vi "NMS_1_1_LTbridge_DiagonalLinearSweep.vi"(1 "Offset":dbl, 4 "b, pF":dbl, 5 "k, pF/V":dbl, 6 "LT bridge\ncalibration":bool, 7 "sweep rate, /min":dbl, 8 "sweep to:":dbl, 9 "sweep":T3(radio)) -> (2 "intercept":dbl, 3 "slope":dbl)   [LabVIEW 2010]
uses:
  Users/Geliang/geliang 1/Desktop/NMS_1_0/Channel.ctl
  Users/Geliang/geliang 1/Desktop/NMS_1_0/Measure.ctl
  Users/Geliang/geliang 1/Desktop/NMS_1_0/HULK SMS/SMScontrols.ctl
  Users/Geliang/geliang 1/Desktop/NMS_1_0/Source.ctl
  <vilib>/Utility/file.llb/Write To Spreadsheet File (DBL).vi
  <vilib>/gmath/NI_Gmath.lvlib
  <vilib>/Analysis/NI_AALPro.lvlib
panel:
  in  "DC bias neg (V)":dbl
  in  "wait to set voltage, msec":u32=3000
  in  "2182A 4":bool
  in  "2182A 3":bool
  in  "2182A 2":bool
  in  "2182A 1":bool
  in  "Slave Channel":T1
  in  "DC bias pos (V)":dbl
  in  "DC_resistance":bool
  in  "Slope":dbl
  in  "Double Sweep":bool
  out "read buffer MercuryIPS":string
  out "MercuryIPS_Error":errorcluster
  in  "MercuryITC":refnum<visa-resource-name>
  in  "MercuryIPS":refnum<visa-resource-name>
  in  "MercuryIPS":bool
  out "x-y*floor(x/y)":i32
  out "XY Graph 2":T2(graph)
  out "R-square total":dbl
  out "XY Graph":T2(graph)
  out "off-zero voltage":dbl
  out "C sample, pF":dbl
  out "R-square":dbl
  in  "pm":dbl=0.04
  in  "points":i16
  in  "C ref, pF":dbl=0.24169
  in  "V exc sample":dbl=0.2
  in  "V exc ref (SR830_2)":dbl=0.18
  in  "LT bridge":bool
  out "Word from HULK!":string
  out "CRYogenic:(":errorcluster
  in  "2182A 5 addr":u8=15
  in  "Hulk_B_meas (Vnano)":bool
  in  "Hulk_SMS_addr":refnum<visa-resource-name>="TCPIP0::10.99.75.17::inst0::INSTR"
  in  "lower limit":dbl
  in  "upper limit":dbl
  in  "continuous":bool
  in  "auto\nrange B":bool
  out "status 2":bool
  out "status":bool
  in  "Show cursor":bool
  in  "time/point, sec":dbl
  out "sweep value":dbl
  out "time delay, ms":dbl
  out "current time":timestamp format="%<%H:%M:%S%1u>T"
  in  "Pause":bool
  in  "LS332 A":bool
  in  "LS332 B":bool
  in  "LS332 addr":u8=28
  in  "LS340 B":bool
  in  "LS340 A":bool
  in  "LS340 addr":u8=28
  in  "AH2700A addr":u8=29
  in  "AH2700A C and L":bool
  in  "AH2500 addr":u8=28
  in  "AH2500 C and L":bool
  in  "2182A 4 ch2":bool
  in  "2182A 4 ch1":bool
  in  "2182A 3 ch2":bool
  in  "2182A 3 ch1":bool
  in  "2182A 2 ch2":bool
  in  "2182A 2 ch1":bool
  in  "2182A 4 addr":u8=18
  in  "2182A 3 addr":u8=17
  in  "2182A 2 addr":u8=16
  in  "2182A 1 addr":u8=15
  in  "2182A 1 ch2":bool
  in  "2182A 1 ch1":bool
  in  "2400 3 addr":u8=14
  in  "2400 2 addr":u8=13
  in  "2400 1 addr":u8=12
  in  "2336A addr":refnum<visa-resource-name>="TCPIP0::10.99.75.17::inst0::INSTR"
  in  "measure time":bool
  in  "2636A smub meas i":bool
  in  "2636A smub meas v":bool
  in  "2636A smua meas i":bool
  in  "2636A smua meas v":bool
  in  "2400 3 meas i":bool
  in  "2400 2 meas i":bool
  in  "2400 2 meas v":bool
  in  "2400 3 meas v":bool
  in  "2400 1 meas i":bool
  in  "2400 1 meas v":bool
  in  "auto\nrange A":bool
  in  "SR830 5 oop":bool
  in  "SR830 5 ip":bool
  in  "SR830 4 oop":bool
  in  "SR830 4 ip":bool
  in  "SR830 3 oop":bool
  in  "SR830 3 ip":bool
  in  "SR830 2 oop":bool
  in  "SR830 2 ip":bool
  in  "SR830 1 oop":bool
  in  "SR830 1 ip":bool
  in  "SR830 5 addr":u8=5
  in  "SR830 4 addr":u8=4
  in  "SR830 3 addr":u8=3
  in  "SR830 2 addr":u8=2
  in  "SR830 1 addr":u8=1
  in  "Y_axis_formula":string
  in  "X_axis_formula":string
  in  "formula_variables":string[](array[string])
  in  "stop":bool
  in  "ready/go":bool
  in  "oldStyle":bool
  out "Data file:":path=path "C:/Users/Artem/data/Year2012/July2012/Jul1312/Jul1312x034.dat"
  in  "Yaxis":u16(ring) caption="Y-axis:" items=["V_sweep_2636a_smub", "2636A_smua_v", "2636A_smua_i", "2636A_smub_v", "2636A_smub_i", "formula"]
  out "data":dbl[](array[numeric])
  out "XY Graph":cluster{dbl[], dbl[]}(graph)
  in  "Xaxis":u16(ring) caption="X-axis:" items=["V_sweep_2636a_smub", "2636A_smua_v", "2636A_smua_i", "2636A_smub_v", "2636A_smub_i", "formula"]
  out "Figure_axis":string[](array[string])
  out "data_caption":string
  # "measure DC res (commute)"
  # "source 2400_2"
  # "SourceMeters"
  # "address"
  # "Hulk_SMS"
  # "MercuryIPS"
  # "2400_1"
  # "2400_2"
  # "2400_3"
  # "2636A_smua"
  # "2636A_smub"
  # "time"
  # "sweep"
  # "measure"
  # "voltage (_v)"
  # "measure with\n2182A_5_ch1"
  # "Field"
  # "current (_i)"
  # "Temperature"
  # "for 2636A_smub slave"
  # "address"
  # "measure"
  # "LS332"
  # "LS340"
  # "MercuryITC"
  # "input A (_A)"
  # "input B (_B)"
  # "LT capacitance bridge on chip"
  # "Capacitance"
  # "with SR830_1"
  # "address"
  # "LTbridge"
  # "measure"
  # "AH2500"
  # "AH2700A"
  # "capacitance (_c)"
  # "and loss (_l)"
  # "every"
  # "Nanovoltmeters"
  # "address"
  # "measure"
  # "2182A_1"
  # "2182A_2"
  # "2182A_3"
  # "2182A_4"
  # "channel 1 (_ch1)"
  # "channel 2 (_ch2)"
  # "(not recommended, slow)"
  # "Lock-in amplifiers"
  # "address"
  # "measure"
  # "SR830_1"
  # "SR830_2"
  # "SR830_3"
  # "SR830_4"
  # "SR830_5"
  # "in phase (_ip)"
  # "out of phase (_oop)"
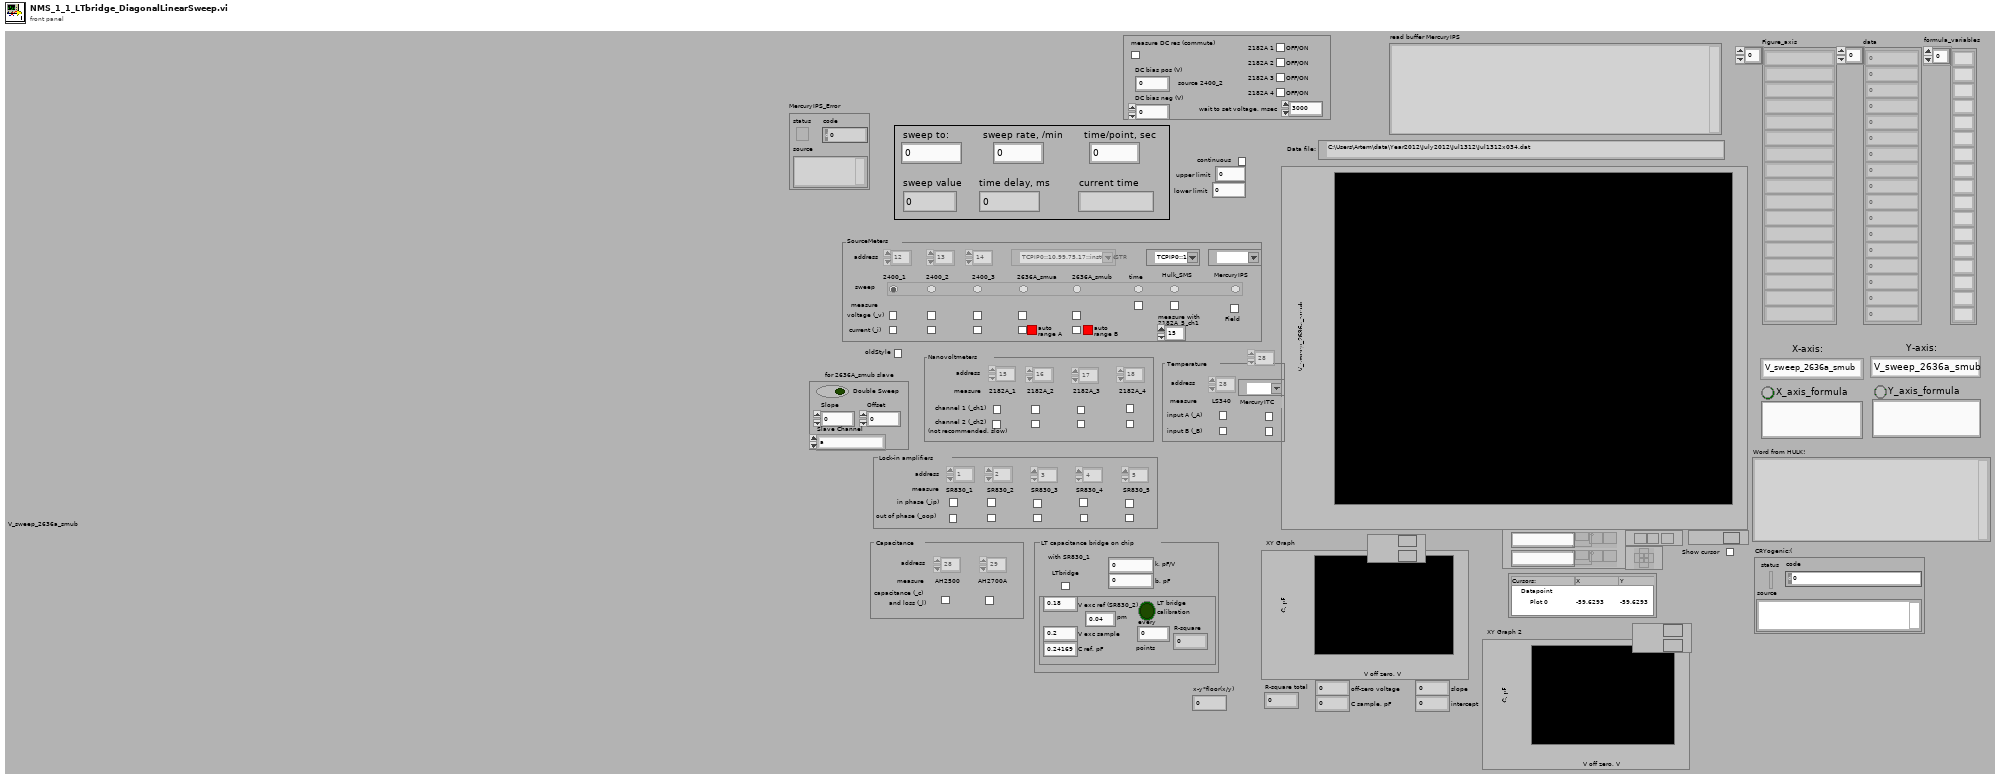
[diagram p1: front panel]
types:
  T1 = typedef "Channel.ctl" = enum16{"a", "b"}
  T2 = cluster{"emty array for LT bridge calibration":dbl[], "Best Linear Fit":dbl[]}[]
  T3 = enum32{"Radio Selection 1", "Radio Selection 2", "Radio Selection 3", "Radio Selection 4", "Radio Selection 5", "Radio Selection 6", "Radio Selection 7", "Radio Selection 8"}
  T4 = typedef "Measure.ctl" = enum16{"Voltage", "Current", "Resistance", "Power"}
  T5 = typedef "SMScontrols.ctl" = enum16{"UPDATE", "GET OUTPUT", "RAMP ZERO", "RAMP MID", "RAMP MAX", "RAMP STATUS", "PAUSE OFF", "PAUSE ON", "HEATER OFF", "HEATER ON", "TESLA OFF", "TESLA ON", "DIRECTION +", "DIRECTION -", "DIRECTION 0", "SET MID", "SET MAX", "SET RAMP", "SET LIMIT", "SET TPA", "SET HEATER"}
  T6 = enum8{"Enabled", "Disabled", "Disabled and Grayed Out"}
  T7 = enum32{"Radio Selection 1", "Radio Selection 2", "Radio Selection 3", "Radio Selection 4", "Radio Selection 5", "Radio Selection 6", "Radio Selection 7"}
  T8 = typedef "Source.ctl" = enum16{"Current", "Voltage"}
  T9 = cluster{"emty array for LT bridge calibration":dbl[], "emty array for LT bridge calibration":dbl[]}
  T10 = cluster{"emty array for LT bridge calibration":dbl[], "Best Linear Fit":dbl[]}
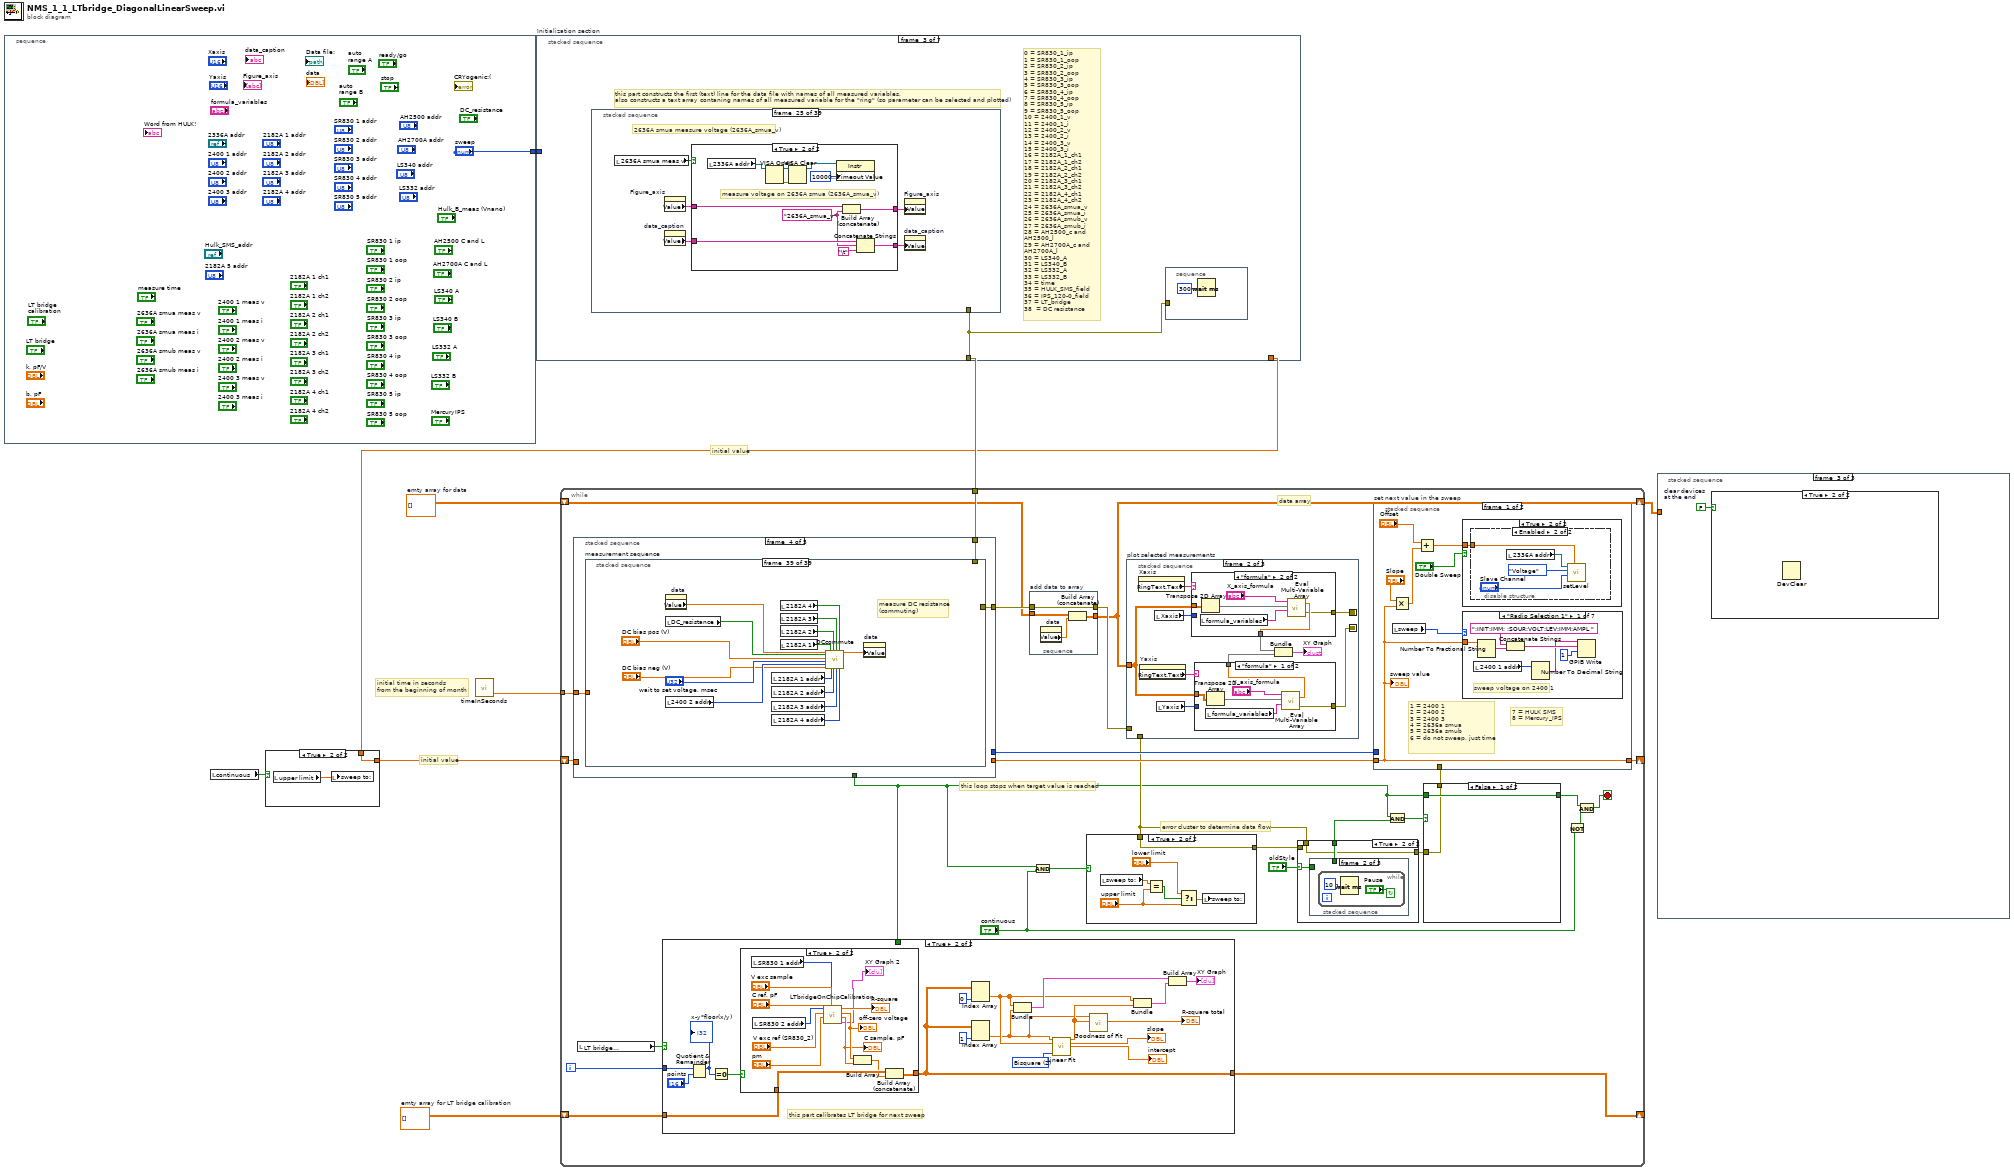
[diagram p0: block diagram]
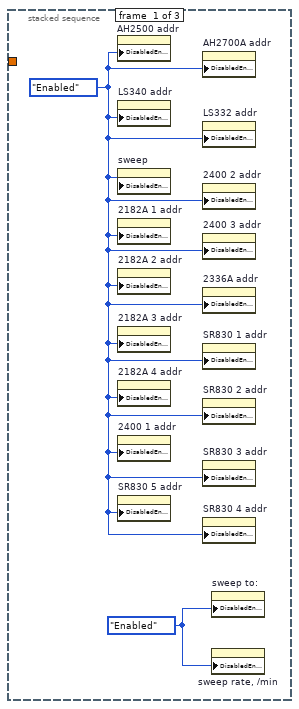
[diagram p3: hidden frame]
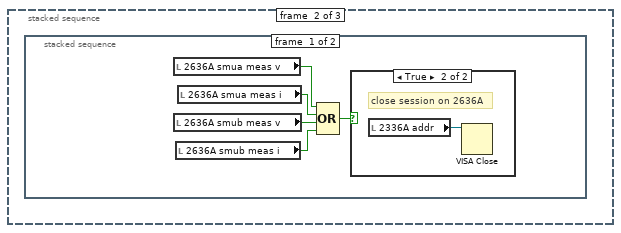
[diagram p4: hidden frame]
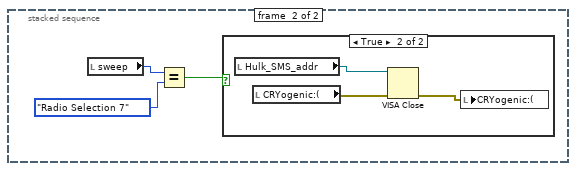
[diagram p6: hidden frame]
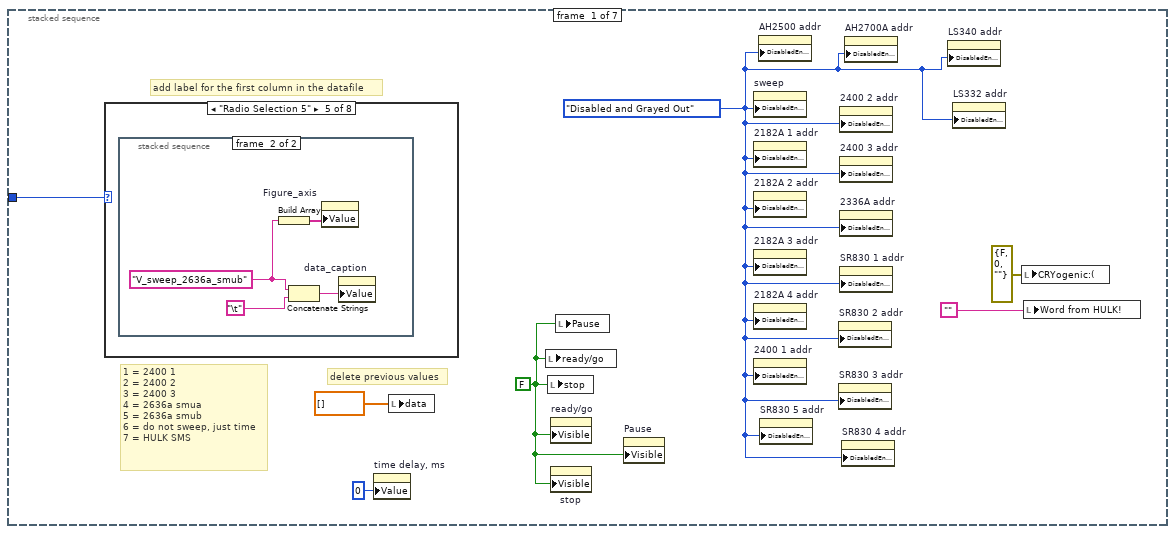
[diagram p9: hidden frame]
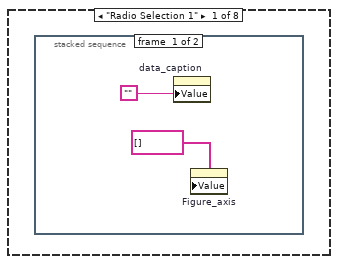
[diagram p10: hidden frame]
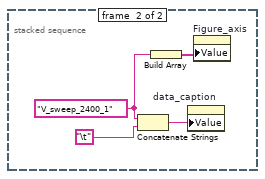
[diagram p11: hidden frame]
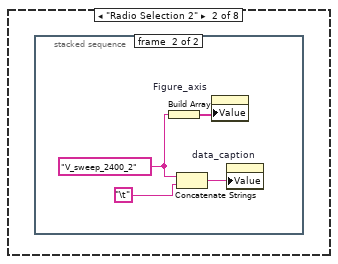
[diagram p12: hidden frame]
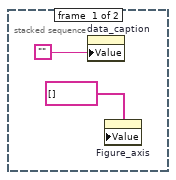
[diagram p13: hidden frame]
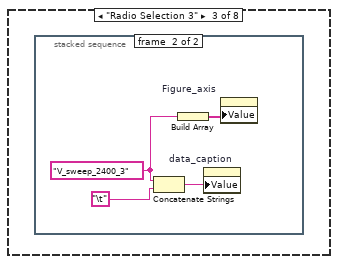
[diagram p14: hidden frame]
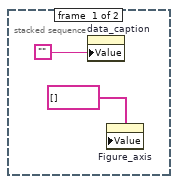
[diagram p15: hidden frame]
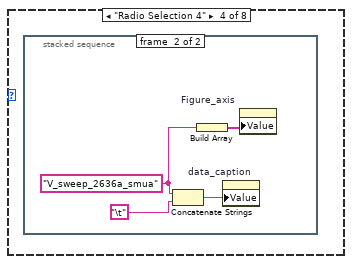
[diagram p16: hidden frame]
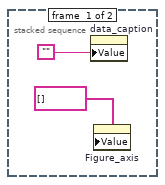
[diagram p17: hidden frame]
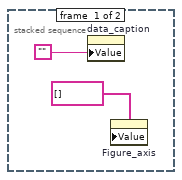
[diagram p18: hidden frame]
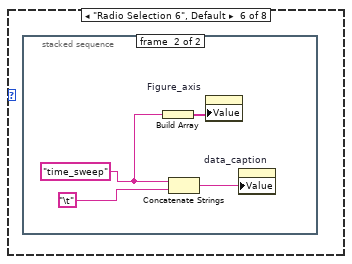
[diagram p19: hidden frame]
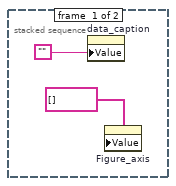
[diagram p20: hidden frame]
diagram:
  w1 = dbl[][] []  # emty array for LT bridge calibration
  w8 = dbl[][] []  # emty array for data
  # "initial value"
  # "initial value"
  # "initial time in seconds\nfrom the beginning of month"
  n1 = stacked-sequence {
    tunnel: ["sweep"] -> w6
    frame #0 {
    }
  }
  n2 = local read "continuous"() -> (w4:bool)
  n3 = call "timeInSeconds.vi"() -> ("Numeric"=w7:dbl)  [unwired: 2 in, 1 out]
  n4 = stacked-sequence "Initialization section" {
    tunnel: [_ _ w79 _ _ _ _] -> w9
    tunnel: [_ _ _ w672 _ _ _] -> w3
    tunnel: w6 -> [w16 _ _ _ _ _ _]
    frame #0 {
      w14 = T6."Disabled and Grayed Out" ("Disabled")
      w15 = FALSE ("stop")
      # "add label for the first column in the datafile"
      # "1 = 2400 1\n2 = 2400 2\n3 = 2400 3\n4 = 2636a smua\n5 = 2636a smub\n6 = do not sweep, just time\n7 = HULK SMS"
      # "delete previous values"
      n5 = case shown="\"Radio Selection 5\"" w16 {
        frame "Radio Selection 1" {
          n6 = stacked-sequence {
            frame #0 {
              n7 = property on="data_caption" class="Str"("Value"="") -> ()  [unwired: 2 in, 2 out]
              n8 = property on="Figure_axis" class="Arr (strict)"("Value"=string[] [] ("Figure_axis_string")) -> ()  [unwired: 2 in, 2 out]
            }
            frame #1 {
              w20 = "V_sweep_2400_1" ("V_sweep")
              n9 = Concatenate Strings(w20, "\t") -> (w22:string)
              n10 = Build Array(w20) -> (w21:string[])
              n11 = property on="data_caption" class="Str"("Value"=w22) -> ()  [unwired: 2 in, 2 out]
              n12 = property on="Figure_axis" class="Arr (strict)"("Value"=w21) -> ()  [unwired: 2 in, 2 out]
            }
          }
        }
        frame "Radio Selection 2" {
          n13 = stacked-sequence {
            frame #0 {
              n14 = property on="data_caption" class="Str"("Value"="") -> ()  [unwired: 2 in, 2 out]
              n15 = property on="Figure_axis" class="Arr (strict)"("Value"=string[] [] ("Figure_axis_string")) -> ()  [unwired: 2 in, 2 out]
            }
            frame #1 {
              w26 = "V_sweep_2400_2" ("V_sweep")
              n16 = Build Array(w26) -> (w27:string[])
              n17 = Concatenate Strings(w26, "\t") -> (w29:string)
              n18 = property on="Figure_axis" class="Arr (strict)"("Value"=w27) -> ()  [unwired: 2 in, 2 out]
              n19 = property on="data_caption" class="Str"("Value"=w29) -> ()  [unwired: 2 in, 2 out]
            }
          }
        }
        frame "Radio Selection 3" {
          n20 = stacked-sequence {
            frame #0 {
              n21 = property on="data_caption" class="Str"("Value"="") -> ()  [unwired: 2 in, 2 out]
              n22 = property on="Figure_axis" class="Arr (strict)"("Value"=string[] [] ("Figure_axis_string")) -> ()  [unwired: 2 in, 2 out]
            }
            frame #1 {
              w32 = "V_sweep_2400_3" ("V_sweep")
              n23 = Concatenate Strings(w32, "\t") -> (w35:string)
              n24 = Build Array(w32) -> (w33:string[])
              n25 = property on="data_caption" class="Str"("Value"=w35) -> ()  [unwired: 2 in, 2 out]
              n26 = property on="Figure_axis" class="Arr (strict)"("Value"=w33) -> ()  [unwired: 2 in, 2 out]
            }
          }
        }
        frame "Radio Selection 4" {
          n27 = stacked-sequence {
            frame #0 {
              n28 = property on="data_caption" class="Str"("Value"="") -> ()  [unwired: 2 in, 2 out]
              n29 = property on="Figure_axis" class="Arr (strict)"("Value"=string[] [] ("Figure_axis_string")) -> ()  [unwired: 2 in, 2 out]
            }
            frame #1 {
              w38 = "V_sweep_2636a_smua" ("V_sweep")
              n30 = Concatenate Strings(w38, "\t") -> (w41:string)
              n31 = Build Array(w38) -> (w39:string[])
              n32 = property on="data_caption" class="Str"("Value"=w41) -> ()  [unwired: 2 in, 2 out]
              n33 = property on="Figure_axis" class="Arr (strict)"("Value"=w39) -> ()  [unwired: 2 in, 2 out]
            }
          }
        }
        frame "Radio Selection 5" {
          n34 = stacked-sequence {
            frame #0 {
              n35 = property on="data_caption" class="Str"("Value"="") -> ()  [unwired: 2 in, 2 out]
              n36 = property on="Figure_axis" class="Arr (strict)"("Value"=string[] [] ("Figure_axis_string")) -> ()  [unwired: 2 in, 2 out]
            }
            frame #1 {
              w44 = "V_sweep_2636a_smub" ("V_sweep")
              n37 = Build Array(w44) -> (w45:string[])
              n38 = Concatenate Strings(w44, "\t") -> (w47:string)
              n39 = property on="Figure_axis" class="Arr (strict)"("Value"=w45) -> ()  [unwired: 2 in, 2 out]
              n40 = property on="data_caption" class="Str"("Value"=w47) -> ()  [unwired: 2 in, 2 out]
            }
          }
        }
        frame "Radio Selection 6", Default {
          n41 = stacked-sequence {
            frame #0 {
              n42 = property on="data_caption" class="Str"("Value"="") -> ()  [unwired: 2 in, 2 out]
              n43 = property on="Figure_axis" class="Arr (strict)"("Value"=string[] [] ("Figure_axis_string")) -> ()  [unwired: 2 in, 2 out]
            }
            frame #1 {
              w50 = "time_sweep" ("V_sweep")
              n44 = Build Array(w50) -> (w51:string[])
              n45 = Concatenate Strings(w50, "\t") -> (w52:string)
              n46 = property on="Figure_axis" class="Arr (strict)"("Value"=w51) -> ()  [unwired: 2 in, 2 out]
              n47 = property on="data_caption" class="Str"("Value"=w52) -> ()  [unwired: 2 in, 2 out]
            }
          }
        }
        frame "Radio Selection 7" {
          # "sweep Hulk SMS"
          n48 = stacked-sequence {
            frame #0 {
              n49 = property on="data_caption" class="Str"("Value"="") -> ()  [unwired: 2 in, 2 out]
              n50 = property on="Figure_axis" class="Arr (strict)"("Value"=string[] [] ("Figure_axis_string")) -> ()  [unwired: 2 in, 2 out]
            }
            frame #1 {
              w56 = "HULK_SMS_output" ("V_sweep")
              n51 = Build Array(w56) -> (w57:string[])
              n52 = Concatenate Strings(w56, "\t") -> (w59:string)
              n53 = property on="Figure_axis" class="Arr (strict)"("Value"=w57) -> ()  [unwired: 2 in, 2 out]
              n54 = property on="data_caption" class="Str"("Value"=w59) -> ()  [unwired: 2 in, 2 out]
            }
          }
        }
        frame "Radio Selection 8" {
          # "sweep Mercury IPS"
          n55 = stacked-sequence {
            frame #0 {
              n56 = property on="data_caption" class="Str"("Value"="") -> ()  [unwired: 2 in, 2 out]
              n57 = property on="Figure_axis" class="Arr (strict)"("Value"=string[] [] ("Figure_axis_string")) -> ()  [unwired: 2 in, 2 out]
            }
            frame #1 {
              w62 = "B_Sweep_Mercury_IPS" ("V_sweep")
              n58 = Build Array(w62) -> (w63:string[])
              n59 = Concatenate Strings(w62, "\t") -> (w65:string)
              n60 = property on="Figure_axis" class="Arr (strict)"("Value"=w63) -> ()  [unwired: 2 in, 2 out]
              n61 = property on="data_caption" class="Str"("Value"=w65) -> ()  [unwired: 2 in, 2 out]
            }
          }
        }
      }
      n62 = property on="time delay, ms" class="DigNum (strict)"("Value"=u32 0 ("delib time delay")) -> ()  [unwired: 2 in, 2 out]
      n63 = local write "data"(dbl[] [] ("data")) -> ()
      n64 = local write "ready/go"(w15) -> ()
      n65 = local write "stop"(w15) -> ()
      n66 = property on="ready/go" class="Bool (strict)"("Visible"=w15) -> ()  [unwired: 2 in, 2 out]
      n67 = property on="stop" class="Bool (strict)"("Visible"=w15) -> ()  [unwired: 2 in, 2 out]
      n68 = local write "Pause"(w15) -> ()
      n69 = property on="Pause" class="Bool (strict)"("Visible"=w15) -> ()  [unwired: 2 in, 2 out]
      n70 = property on="sweep" class="RadioBtnsControl (strict)"("DisabledEnum"=w14) -> ()  [unwired: 2 in, 2 out]
      n71 = property on="2182A 1 addr" class="DigNum (strict)"("DisabledEnum"=w14) -> ()  [unwired: 2 in, 2 out]
      n72 = property on="2182A 2 addr" class="DigNum (strict)"("DisabledEnum"=w14) -> ()  [unwired: 2 in, 2 out]
      n73 = property on="2182A 3 addr" class="DigNum (strict)"("DisabledEnum"=w14) -> ()  [unwired: 2 in, 2 out]
      n74 = property on="2182A 4 addr" class="DigNum (strict)"("DisabledEnum"=w14) -> ()  [unwired: 2 in, 2 out]
      n75 = property on="2400 1 addr" class="DigNum (strict)"("DisabledEnum"=w14) -> ()  [unwired: 2 in, 2 out]
      n76 = property on="AH2500 addr" class="DigNum (strict)"("DisabledEnum"=w14) -> ()  [unwired: 2 in, 2 out]
      n77 = property on="SR830 5 addr" class="DigNum (strict)"("DisabledEnum"=w14) -> ()  [unwired: 2 in, 2 out]
      n78 = property on="SR830 2 addr" class="DigNum (strict)"("DisabledEnum"=w14) -> ()  [unwired: 2 in, 2 out]
      n79 = property on="SR830 3 addr" class="DigNum (strict)"("DisabledEnum"=w14) -> ()  [unwired: 2 in, 2 out]
      n80 = property on="2400 2 addr" class="DigNum (strict)"("DisabledEnum"=w14) -> ()  [unwired: 2 in, 2 out]
      n81 = property on="2400 3 addr" class="DigNum (strict)"("DisabledEnum"=w14) -> ()  [unwired: 2 in, 2 out]
      n82 = property on="2336A addr" class="VISAName"("DisabledEnum"=w14) -> ()  [unwired: 2 in, 2 out]
      n83 = property on="SR830 1 addr" class="DigNum (strict)"("DisabledEnum"=w14) -> ()  [unwired: 2 in, 2 out]
      n84 = property on="SR830 4 addr" class="DigNum (strict)"("DisabledEnum"=w14) -> ()  [unwired: 2 in, 2 out]
      n85 = property on="AH2700A addr" class="DigNum (strict)"("DisabledEnum"=w14) -> ()  [unwired: 2 in, 2 out]
      n86 = property on="LS340 addr" class="DigNum (strict)"("DisabledEnum"=w14) -> ()  [unwired: 2 in, 2 out]
      n87 = property on="LS332 addr" class="DigNum (strict)"("DisabledEnum"=w14) -> ()  [unwired: 2 in, 2 out]
      n88 = local write "CRYogenic:("(errorcluster {"status"=FALSE, "code"=0, "source"=""} ("CRYogenic:(")) -> ()
      n89 = local write "Word from HULK!"("") -> ()
    }
    frame #1 {
      n90 = local read "2636A smua meas v"() -> (w71:bool)
      n91 = local read "2636A smub meas v"() -> (w69:bool)
      n92 = local read "2636A smub meas i"() -> (w68:bool)
      n93 = local read "2636A smua meas i"() -> (w70:bool)
      n94 = Compound Arithmetic op=OR(w71, w70, w69, w68) -> (w67:bool)
      n95 = case shown="True" w67 {
        frame False {
        }
        frame True {
          # "opens session for 2636a system sourcemeter"
          n96 = local read "2336A addr"() -> (w78:refnum<visa-resource-name>)
          n97 = VISA Close(VISA resource name=w78) -> ()  [unwired: 1 in, 1 out]
        }
      }
      n98 = local read "MercuryIPS"() -> (w66:bool)
      n99 = case shown="True" w66 {
        frame False {
        }
        frame True {
          n100 = local read "MercuryIPS"() -> (w74:refnum<visa-resource-name>)
          n101 = VISA Close(VISA resource name=w74) -> (error out=w73:errorcluster)  [unwired: 1 in]
          n102 = flat-sequence {
            tunnel: w73 -> [w76]
            tunnel: [w76] -> w72
            frame #0 {
              n103 = Wait (ms)(milliseconds to wait=u32 200) -> ()  [unwired: 1 out]
            }
          }
          n104 = VISA Open(error in (no error)=w72, VISA resource name=w74) -> (error out=w75:errorcluster)  [unwired: 3 in, 1 out]
          n105 = local write "MercuryIPS_Error"(w75) -> ()
        }
      }
    }
    frame #2 {
      # "0 = SR830_1_ip\n1 = SR830_1_oop\n2 = SR830_2_ip\n3 = SR830_2_oop\n4 = SR830_3_ip\n5 = SR830_3_oop\n6 = SR830_4_ip \n7 = SR830_4_oop \n8 = SR830_5_ip \n9 = SR830_5_oop \n10 = 2400_1_v \n11 = 2400_1_i \n12 = 2400_2_v\n13 = 2400_2_i \n14 = 2400_3_v \n15 = 2400_3_i \n16 = 2182A_1_ch1 \n17 = 2182A_1_ch2 \n18 = 2182A_2_ch1 \n19 = 2182A_2_ch2\n20 = 2182A_3_ch1 \n21 = 2182A_3_ch2 \n22 = 2182A_4_ch1 \n23 = 2182A_4_ch2 \n24 = 2636A_smua_v \n25 = 2636A_smua_i \n26 = 2636A_smub_v \n27 = 2636A_smub_i \n28 = AH2500_c and AH2500_l \n29 = AH2700A_c and AH2700A_l\n30 = LS340_A\n31 = LS340_B\n32 = LS332_A\n33 = LS332_B\n34 = time\n35 = HULK_SMS_field\n36 = IPS_120-0_field\n37 = LT_bridge\n38  = DC resistance"
      # "this part constructs the first (text) line for the data file with names of all measured variables,\nalso constructs a text array contaning names of all measured variable for the \"ring\" (so parameter can be selected and plotted)"
      n106 = stacked-sequence {
        tunnel: [w81 _ _ _ _ _ _ _ _ _ _ _ _ _ _ _ _ _ _ _ _ _ _ _ _ _ _ _ _ _ _ _ _ _ _ _ _ _ _] -> w79
        frame #0 {
          # "SR830 1 in phase (SR830_1_ip)"
          n107 = local read "SR830 1 ip"() -> (w86:bool)
          n108 = property on="Figure_axis" class="Arr (strict)"() -> ("Value"=w83:string[])  [unwired: 2 in, 2 out]
          n109 = property on="data_caption" class="Str"() -> ("Value"=w85:string)  [unwired: 2 in, 2 out]
          n110 = case shown="True" w86 {
            tunnel: w85 -> [w88 w94]
            tunnel: [w88 w93] -> w84
            tunnel: w83 -> [w87 w91]
            tunnel: [w87 w89] -> w82
            frame False {
              # "not measure SR830 1 in phase signal (SR830_1_ip)"
            }
            frame True {
              w90 = "SR830_1_ip"
              # "measure SR830 1 in phase signal (SR830_1_ip)"
              n111 = local read "SR830 1 addr"() -> (w95:u8)
              n112 = Number To Decimal String(number=w95) -> (decimal integer string=w96:string)  [unwired: 1 in]
              n113 = GPIB Clear(3:w96) -> ()  [unwired: 1 in, 2 out]
              n114 = Build Array (concatenate)(w91, w90) -> (w89:string[])
              n115 = Concatenate Strings(w94, w90, "\t") -> (w93:string)
            }
          }
          n116 = property on="Figure_axis" class="Arr (strict)"("Value"=w82) -> ()  [unwired: 2 in, 2 out]
          n117 = property on="data_caption" class="Str"("Value"=w84) -> (error out=w81:errorcluster)  [unwired: 2 in, 1 out]
        }
        frame #1 {
          # "SR830 1 out of phase (SR830_1_oop)"
          n118 = local read "SR830 1 oop"() -> (w101:bool)
          n119 = property on="Figure_axis" class="Arr (strict)"() -> ("Value"=w98:string[])  [unwired: 2 in, 2 out]
          n120 = property on="data_caption" class="Str"() -> ("Value"=w100:string)  [unwired: 2 in, 2 out]
          n121 = case shown="True" w101 {
            tunnel: w100 -> [w103 w109]
            tunnel: [w103 w108] -> w99
            tunnel: w98 -> [w102 w106]
            tunnel: [w102 w104] -> w97
            frame False {
              # "not measure SR830 1 out of phase signal (SR830_1_oop)"
            }
            frame True {
              w105 = "SR830_1_oop"
              # "measure SR830 1 out of phase signal (SR830_1_oop)"
              n122 = local read "SR830 1 addr"() -> (w110:u8)
              n123 = Number To Decimal String(number=w110) -> (decimal integer string=w111:string)  [unwired: 1 in]
              n124 = GPIB Clear(3:w111) -> ()  [unwired: 1 in, 2 out]
              n125 = Build Array (concatenate)(w106, w105) -> (w104:string[])
              n126 = Concatenate Strings(w109, w105, "\t") -> (w108:string)
            }
          }
          n127 = property on="Figure_axis" class="Arr (strict)"("Value"=w97) -> ()  [unwired: 2 in, 2 out]
          n128 = property on="data_caption" class="Str"("Value"=w99) -> ()  [unwired: 2 in, 2 out]
        }
        frame #2 {
          # "SR830 2 in phase (SR830_2_ip)"
          n129 = local read "SR830 2 ip"() -> (w116:bool)
          n130 = property on="Figure_axis" class="Arr (strict)"() -> ("Value"=w113:string[])  [unwired: 2 in, 2 out]
          n131 = property on="data_caption" class="Str"() -> ("Value"=w115:string)  [unwired: 2 in, 2 out]
          n132 = case shown="False" w116 {
            tunnel: w115 -> [w118 w124]
            tunnel: [w118 w123] -> w114
            tunnel: w113 -> [w117 w121]
            tunnel: [w117 w119] -> w112
            frame False {
              # "not measure SR830 2 in phase signal (SR830_2_ip)"
            }
            frame True {
              w120 = "SR830_2_ip"
              # "measure SR830 2 in phase signal (SR830_2_ip)"
              n133 = local read "SR830 2 addr"() -> (w125:u8)
              n134 = Number To Decimal String(number=w125) -> (decimal integer string=w126:string)  [unwired: 1 in]
              n135 = GPIB Clear(3:w126) -> ()  [unwired: 1 in, 2 out]
              n136 = Build Array (concatenate)(w121, w120) -> (w119:string[])
              n137 = Concatenate Strings(w124, w120, "\t") -> (w123:string)
            }
          }
          n138 = property on="Figure_axis" class="Arr (strict)"("Value"=w112) -> ()  [unwired: 2 in, 2 out]
          n139 = property on="data_caption" class="Str"("Value"=w114) -> ()  [unwired: 2 in, 2 out]
        }
        frame #3 {
          # "SR830 2 out of phase (SR830_2_oop)"
          n140 = local read "SR830 2 oop"() -> (w131:bool)
          n141 = property on="Figure_axis" class="Arr (strict)"() -> ("Value"=w128:string[])  [unwired: 2 in, 2 out]
          n142 = property on="data_caption" class="Str"() -> ("Value"=w130:string)  [unwired: 2 in, 2 out]
          n143 = case shown="True" w131 {
            tunnel: w130 -> [w133 w139]
            tunnel: [w133 w138] -> w129
            tunnel: w128 -> [w132 w136]
            tunnel: [w132 w134] -> w127
            frame False {
              # "not measure SR830 2 out of phase signal (SR830_2_oop)"
            }
            frame True {
              w135 = "SR830_2_oop"
              # "measure SR830 2 out of phase signal (SR830_2_oop)"
              n144 = local read "SR830 2 addr"() -> (w140:u8)
              n145 = Number To Decimal String(number=w140) -> (decimal integer string=w141:string)  [unwired: 1 in]
              n146 = GPIB Clear(3:w141) -> ()  [unwired: 1 in, 2 out]
              n147 = Build Array (concatenate)(w136, w135) -> (w134:string[])
              n148 = Concatenate Strings(w139, w135, "\t") -> (w138:string)
            }
          }
          n149 = property on="Figure_axis" class="Arr (strict)"("Value"=w127) -> ()  [unwired: 2 in, 2 out]
          n150 = property on="data_caption" class="Str"("Value"=w129) -> ()  [unwired: 2 in, 2 out]
        }
        frame #4 {
          # "SR830 3 in phase (SR830_3_ip)"
          n151 = local read "SR830 3 ip"() -> (w146:bool)
          n152 = property on="Figure_axis" class="Arr (strict)"() -> ("Value"=w143:string[])  [unwired: 2 in, 2 out]
          n153 = property on="data_caption" class="Str"() -> ("Value"=w145:string)  [unwired: 2 in, 2 out]
          n154 = case shown="False" w146 {
            tunnel: w145 -> [w148 w154]
            tunnel: [w148 w153] -> w144
            tunnel: w143 -> [w147 w151]
            tunnel: [w147 w149] -> w142
            frame False {
              # "not measure SR830 3 in phase signal (SR830_3_ip)"
            }
            frame True {
              w150 = "SR830_3_ip"
              # "measure SR830 3 in phase signal (SR830_3_ip)"
              n155 = local read "SR830 3 addr"() -> (w155:u8)
              n156 = Number To Decimal String(number=w155) -> (decimal integer string=w156:string)  [unwired: 1 in]
              n157 = GPIB Clear(3:w156) -> ()  [unwired: 1 in, 2 out]
              n158 = Build Array (concatenate)(w151, w150) -> (w149:string[])
              n159 = Concatenate Strings(w154, w150, "\t") -> (w153:string)
            }
          }
          n160 = property on="Figure_axis" class="Arr (strict)"("Value"=w142) -> ()  [unwired: 2 in, 2 out]
          n161 = property on="data_caption" class="Str"("Value"=w144) -> ()  [unwired: 2 in, 2 out]
        }
        frame #5 {
          # "SR830 3 out of phase (SR830_3_oop)"
          n162 = local read "SR830 3 oop"() -> (w161:bool)
          n163 = property on="Figure_axis" class="Arr (strict)"() -> ("Value"=w158:string[])  [unwired: 2 in, 2 out]
          n164 = property on="data_caption" class="Str"() -> ("Value"=w160:string)  [unwired: 2 in, 2 out]
          n165 = case shown="True" w161 {
            tunnel: w160 -> [w163 w169]
            tunnel: [w163 w168] -> w159
            tunnel: w158 -> [w162 w166]
            tunnel: [w162 w164] -> w157
            frame False {
              # "not measure SR830 3 out of phase signal (SR830_3_oop)"
            }
            frame True {
              w165 = "SR830_3_oop"
              # "measure SR830 3 out phase signal (SR830_3_oop)"
              n166 = local read "SR830 3 addr"() -> (w170:u8)
              n167 = Number To Decimal String(number=w170) -> (decimal integer string=w171:string)  [unwired: 1 in]
              n168 = GPIB Clear(3:w171) -> ()  [unwired: 1 in, 2 out]
              n169 = Build Array (concatenate)(w166, w165) -> (w164:string[])
              n170 = Concatenate Strings(w169, w165, "\t") -> (w168:string)
            }
          }
          n171 = property on="Figure_axis" class="Arr (strict)"("Value"=w157) -> ()  [unwired: 2 in, 2 out]
          n172 = property on="data_caption" class="Str"("Value"=w159) -> ()  [unwired: 2 in, 2 out]
        }
        frame #6 {
          # "SR830 4 in phase (SR830_4_ip)"
          n173 = local read "SR830 4 ip"() -> (w176:bool)
          n174 = property on="Figure_axis" class="Arr (strict)"() -> ("Value"=w173:string[])  [unwired: 2 in, 2 out]
          n175 = property on="data_caption" class="Str"() -> ("Value"=w175:string)  [unwired: 2 in, 2 out]
          n176 = case shown="True" w176 {
            tunnel: w175 -> [w178 w184]
            tunnel: [w178 w183] -> w174
            tunnel: w173 -> [w177 w181]
            tunnel: [w177 w179] -> w172
            frame False {
              # "not measure SR830 4 in phase signal (SR830_4_ip)"
            }
            frame True {
              w180 = "SR830_4_ip"
              # "measure SR830 4 in phase signal (SR830_4_ip)"
              n177 = local read "SR830 4 addr"() -> (w185:u8)
              n178 = Number To Decimal String(number=w185) -> (decimal integer string=w186:string)  [unwired: 1 in]
              n179 = GPIB Clear(3:w186) -> ()  [unwired: 1 in, 2 out]
              n180 = Build Array (concatenate)(w181, w180) -> (w179:string[])
              n181 = Concatenate Strings(w184, w180, "\t") -> (w183:string)
            }
          }
          n182 = property on="Figure_axis" class="Arr (strict)"("Value"=w172) -> ()  [unwired: 2 in, 2 out]
          n183 = property on="data_caption" class="Str"("Value"=w174) -> ()  [unwired: 2 in, 2 out]
        }
        frame #7 {
          # "SR830 4 out of phase (SR830_4_oop)"
          n184 = local read "SR830 4 oop"() -> (w191:bool)
          n185 = property on="Figure_axis" class="Arr (strict)"() -> ("Value"=w188:string[])  [unwired: 2 in, 2 out]
          n186 = property on="data_caption" class="Str"() -> ("Value"=w190:string)  [unwired: 2 in, 2 out]
          n187 = case shown="True" w191 {
            tunnel: w190 -> [w193 w199]
            tunnel: [w193 w198] -> w189
            tunnel: w188 -> [w192 w196]
            tunnel: [w192 w194] -> w187
            frame False {
              # "not measure SR830 4 out of phase signal (SR830_4_oop)"
            }
            frame True {
              w195 = "SR830_4_oop"
              # "measure SR830 4 out of phase signal (SR830_4_oop)"
              n188 = local read "SR830 4 addr"() -> (w200:u8)
              n189 = Number To Decimal String(number=w200) -> (decimal integer string=w201:string)  [unwired: 1 in]
              n190 = GPIB Clear(3:w201) -> ()  [unwired: 1 in, 2 out]
              n191 = Build Array (concatenate)(w196, w195) -> (w194:string[])
              n192 = Concatenate Strings(w199, w195, "\t") -> (w198:string)
            }
          }
          n193 = property on="Figure_axis" class="Arr (strict)"("Value"=w187) -> ()  [unwired: 2 in, 2 out]
          n194 = property on="data_caption" class="Str"("Value"=w189) -> ()  [unwired: 2 in, 2 out]
        }
        frame #8 {
          # "SR830 5 in phase (SR830_5_ip)"
          n195 = local read "SR830 5 ip"() -> (w206:bool)
          n196 = property on="Figure_axis" class="Arr (strict)"() -> ("Value"=w203:string[])  [unwired: 2 in, 2 out]
          n197 = property on="data_caption" class="Str"() -> ("Value"=w205:string)  [unwired: 2 in, 2 out]
          n198 = case shown="True" w206 {
            tunnel: w205 -> [w208 w214]
            tunnel: [w208 w213] -> w204
            tunnel: w203 -> [w207 w211]
            tunnel: [w207 w209] -> w202
            frame False {
              # "not measure SR830 5 in phase signal (SR830_5_ip)"
            }
            frame True {
              w210 = "SR830_5_ip"
              # "measure SR830 5 in phase signal (SR830_5_ip)"
              n199 = local read "SR830 5 addr"() -> (w215:u8)
              n200 = Number To Decimal String(number=w215) -> (decimal integer string=w216:string)  [unwired: 1 in]
              n201 = GPIB Clear(3:w216) -> ()  [unwired: 1 in, 2 out]
              n202 = Build Array (concatenate)(w211, w210) -> (w209:string[])
              n203 = Concatenate Strings(w214, w210, "\t") -> (w213:string)
            }
          }
          n204 = property on="Figure_axis" class="Arr (strict)"("Value"=w202) -> ()  [unwired: 2 in, 2 out]
          n205 = property on="data_caption" class="Str"("Value"=w204) -> ()  [unwired: 2 in, 2 out]
        }
        frame #9 {
          # "SR830 5 out of phase (SR830_5_oop)"
          n206 = local read "SR830 5 oop"() -> (w221:bool)
          n207 = property on="Figure_axis" class="Arr (strict)"() -> ("Value"=w218:string[])  [unwired: 2 in, 2 out]
          n208 = property on="data_caption" class="Str"() -> ("Value"=w220:string)  [unwired: 2 in, 2 out]
          n209 = case shown="False" w221 {
            tunnel: w220 -> [w223 w229]
            tunnel: [w223 w228] -> w219
            tunnel: w218 -> [w222 w226]
            tunnel: [w222 w224] -> w217
            frame False {
              # "not measure SR830 5 out of phase signal (SR830_5_oop)"
            }
            frame True {
              w225 = "SR830_5_oop"
              # "measure SR830 5 out of phase signal (SR830_5_oop)"
              n210 = local read "SR830 5 addr"() -> (w230:u8)
              n211 = Number To Decimal String(number=w230) -> (decimal integer string=w231:string)  [unwired: 1 in]
              n212 = GPIB Clear(3:w231) -> ()  [unwired: 1 in, 2 out]
              n213 = Build Array (concatenate)(w226, w225) -> (w224:string[])
              n214 = Concatenate Strings(w229, w225, "\t") -> (w228:string)
            }
          }
          n215 = property on="Figure_axis" class="Arr (strict)"("Value"=w217) -> ()  [unwired: 2 in, 2 out]
          n216 = property on="data_caption" class="Str"("Value"=w219) -> ()  [unwired: 2 in, 2 out]
        }
        frame #10 {
          # "2400 1 voltage measure (2400_1_v)"
          n217 = local read "2400 1 meas v"() -> (w236:bool)
          n218 = property on="Figure_axis" class="Arr (strict)"() -> ("Value"=w233:string[])  [unwired: 2 in, 2 out]
          n219 = property on="data_caption" class="Str"() -> ("Value"=w235:string)  [unwired: 2 in, 2 out]
          n220 = case shown="True" w236 {
            tunnel: w235 -> [w238 w244]
            tunnel: [w238 w243] -> w234
            tunnel: w233 -> [w237 w241]
            tunnel: [w237 w239] -> w232
            frame False {
              # "not measure 2400 1 voltage (2400_1_v)"
            }
            frame True {
              w240 = "2400_1_v"
              # "measure 2400 1 voltage (2400_1_v)"
              n221 = local read "2400 1 addr"() -> (w245:u8)
              n222 = Number To Decimal String(number=w245) -> (decimal integer string=w246:string)  [unwired: 1 in]
              n223 = GPIB Clear(3:w246) -> ()  [unwired: 1 in, 2 out]
              n224 = Build Array (concatenate)(w241, w240) -> (w239:string[])
              n225 = Concatenate Strings(w244, w240, "\t") -> (w243:string)
            }
          }
          n226 = property on="Figure_axis" class="Arr (strict)"("Value"=w232) -> ()  [unwired: 2 in, 2 out]
          n227 = property on="data_caption" class="Str"("Value"=w234) -> ()  [unwired: 2 in, 2 out]
        }
        frame #11 {
          # "2400 1 current measure (2400_1_i)"
          n228 = local read "2400 1 meas i"() -> (w251:bool)
          n229 = property on="Figure_axis" class="Arr (strict)"() -> ("Value"=w248:string[])  [unwired: 2 in, 2 out]
          n230 = property on="data_caption" class="Str"() -> ("Value"=w250:string)  [unwired: 2 in, 2 out]
          n231 = case shown="True" w251 {
            tunnel: w250 -> [w253 w259]
            tunnel: [w253 w258] -> w249
            tunnel: w248 -> [w252 w256]
            tunnel: [w252 w254] -> w247
            frame False {
              # "not measure 2400 1 current (2400_1_i)"
            }
            frame True {
              w255 = "2400_1_i"
              # "measure 2400 1 current (2400_1_i)"
              n232 = local read "2400 1 addr"() -> (w260:u8)
              n233 = Number To Decimal String(number=w260) -> (decimal integer string=w261:string)  [unwired: 1 in]
              n234 = GPIB Clear(3:w261) -> ()  [unwired: 1 in, 2 out]
              n235 = Build Array (concatenate)(w256, w255) -> (w254:string[])
              n236 = Concatenate Strings(w259, w255, "\t") -> (w258:string)
            }
          }
          n237 = property on="Figure_axis" class="Arr (strict)"("Value"=w247) -> ()  [unwired: 2 in, 2 out]
          n238 = property on="data_caption" class="Str"("Value"=w249) -> ()  [unwired: 2 in, 2 out]
        }
        frame #12 {
          # "2400 2 voltage measure (2400_2_v)"
          n239 = local read "2400 2 meas v"() -> (w266:bool)
          n240 = property on="Figure_axis" class="Arr (strict)"() -> ("Value"=w263:string[])  [unwired: 2 in, 2 out]
          n241 = property on="data_caption" class="Str"() -> ("Value"=w265:string)  [unwired: 2 in, 2 out]
          n242 = case shown="True" w266 {
            tunnel: w265 -> [w268 w274]
            tunnel: [w268 w273] -> w264
            tunnel: w263 -> [w267 w271]
            tunnel: [w267 w269] -> w262
            frame False {
              # "not measure 2400 2 voltage (2400_2_v)"
            }
            frame True {
              w270 = "2400_2_v"
              # "measure 2400 2 voltage (2400_2_v)"
              n243 = local read "2400 2 addr"() -> (w275:u8)
              n244 = Number To Decimal String(number=w275) -> (decimal integer string=w276:string)  [unwired: 1 in]
              n245 = GPIB Clear(3:w276) -> ()  [unwired: 1 in, 2 out]
              n246 = Build Array (concatenate)(w271, w270) -> (w269:string[])
              n247 = Concatenate Strings(w274, w270, "\t") -> (w273:string)
            }
          }
          n248 = property on="Figure_axis" class="Arr (strict)"("Value"=w262) -> ()  [unwired: 2 in, 2 out]
          n249 = property on="data_caption" class="Str"("Value"=w264) -> ()  [unwired: 2 in, 2 out]
        }
        frame #13 {
          # "2400 2 current measure (2400_2_i)"
          n250 = local read "2400 2 meas i"() -> (w281:bool)
          n251 = property on="Figure_axis" class="Arr (strict)"() -> ("Value"=w278:string[])  [unwired: 2 in, 2 out]
          n252 = property on="data_caption" class="Str"() -> ("Value"=w280:string)  [unwired: 2 in, 2 out]
          n253 = case shown="True" w281 {
            tunnel: w280 -> [w283 w289]
            tunnel: [w283 w288] -> w279
            tunnel: w278 -> [w282 w286]
            tunnel: [w282 w284] -> w277
            frame False {
              # "not measure 2400 2 current (2400_2_i)"
            }
            frame True {
              w285 = "2400_2_i"
              # "measure 2400 2 current (2400_2_i)"
              n254 = local read "2400 2 addr"() -> (w290:u8)
              n255 = Number To Decimal String(number=w290) -> (decimal integer string=w291:string)  [unwired: 1 in]
              n256 = GPIB Clear(3:w291) -> ()  [unwired: 1 in, 2 out]
              n257 = Build Array (concatenate)(w286, w285) -> (w284:string[])
              n258 = Concatenate Strings(w289, w285, "\t") -> (w288:string)
            }
          }
          n259 = property on="Figure_axis" class="Arr (strict)"("Value"=w277) -> ()  [unwired: 2 in, 2 out]
          n260 = property on="data_caption" class="Str"("Value"=w279) -> ()  [unwired: 2 in, 2 out]
        }
        frame #14 {
          # "2400 3 voltage measure (2400_3_v)"
          n261 = local read "2400 3 meas v"() -> (w296:bool)
          n262 = property on="Figure_axis" class="Arr (strict)"() -> ("Value"=w293:string[])  [unwired: 2 in, 2 out]
          n263 = property on="data_caption" class="Str"() -> ("Value"=w295:string)  [unwired: 2 in, 2 out]
          n264 = case shown="False" w296 {
            tunnel: w295 -> [w298 w304]
            tunnel: [w298 w303] -> w294
            tunnel: w293 -> [w297 w301]
            tunnel: [w297 w299] -> w292
            frame False {
              # "not measure 2400 3 voltage (2400_3_v)"
            }
            frame True {
              w300 = "2400_3_v"
              # "measure 2400 3 voltage (2400_3_v)"
              n265 = local read "2400 3 addr"() -> (w305:u8)
              n266 = Number To Decimal String(number=w305) -> (decimal integer string=w306:string)  [unwired: 1 in]
              n267 = GPIB Clear(3:w306) -> ()  [unwired: 1 in, 2 out]
              n268 = Build Array (concatenate)(w301, w300) -> (w299:string[])
              n269 = Concatenate Strings(w304, w300, "\t") -> (w303:string)
            }
          }
          n270 = property on="Figure_axis" class="Arr (strict)"("Value"=w292) -> ()  [unwired: 2 in, 2 out]
          n271 = property on="data_caption" class="Str"("Value"=w294) -> ()  [unwired: 2 in, 2 out]
        }
        frame #15 {
          # "2400 3 current measure (2400_3_i)"
          n272 = local read "2400 3 meas i"() -> (w311:bool)
          n273 = property on="Figure_axis" class="Arr (strict)"() -> ("Value"=w308:string[])  [unwired: 2 in, 2 out]
          n274 = property on="data_caption" class="Str"() -> ("Value"=w310:string)  [unwired: 2 in, 2 out]
          n275 = case shown="True" w311 {
            tunnel: w310 -> [w313 w319]
            tunnel: [w313 w318] -> w309
            tunnel: w308 -> [w312 w316]
            tunnel: [w312 w314] -> w307
            frame False {
              # "not measure 2400 3 current (2400_3_i)"
            }
            frame True {
              w315 = "2400_3_i"
              # "measure 2400 3 current (2400_3_i)"
              n276 = local read "2400 3 addr"() -> (w320:u8)
              n277 = Number To Decimal String(number=w320) -> (decimal integer string=w321:string)  [unwired: 1 in]
              n278 = GPIB Clear(3:w321) -> ()  [unwired: 1 in, 2 out]
              n279 = Build Array (concatenate)(w316, w315) -> (w314:string[])
              n280 = Concatenate Strings(w319, w315, "\t") -> (w318:string)
            }
          }
          n281 = property on="Figure_axis" class="Arr (strict)"("Value"=w307) -> ()  [unwired: 2 in, 2 out]
          n282 = property on="data_caption" class="Str"("Value"=w309) -> ()  [unwired: 2 in, 2 out]
        }
        frame #16 {
          # "2182A 1 channel 1 measure (2182A_1_ch1)"
          n283 = local read "2182A 1 ch1"() -> (w326:bool)
          n284 = property on="Figure_axis" class="Arr (strict)"() -> ("Value"=w323:string[])  [unwired: 2 in, 2 out]
          n285 = property on="data_caption" class="Str"() -> ("Value"=w325:string)  [unwired: 2 in, 2 out]
          n286 = case shown="False" w326 {
            tunnel: w325 -> [w328 w334]
            tunnel: [w328 w333] -> w324
            tunnel: w323 -> [w327 w331]
            tunnel: [w327 w329] -> w322
            frame False {
              # "not measure 2182A 1 channel 1 (2182A_1_ch1)"
            }
            frame True {
              w330 = "2182A_1_ch1"
              # "measure 2182A 1 channel 1 (2182A_1_ch1)"
              n287 = local read "2182A 1 addr"() -> (w335:u8)
              n288 = Number To Decimal String(number=w335) -> (decimal integer string=w336:string)  [unwired: 1 in]
              n289 = GPIB Clear(3:w336) -> ()  [unwired: 1 in, 2 out]
              n290 = Build Array (concatenate)(w331, w330) -> (w329:string[])
              n291 = Concatenate Strings(w334, w330, "\t") -> (w333:string)
            }
          }
          n292 = property on="Figure_axis" class="Arr (strict)"("Value"=w322) -> ()  [unwired: 2 in, 2 out]
          n293 = property on="data_caption" class="Str"("Value"=w324) -> ()  [unwired: 2 in, 2 out]
        }
        frame #17 {
          # "2182A 1 channel 2 measure (2182A_1_ch2)"
          n294 = local read "2182A 1 ch2"() -> (w341:bool)
          n295 = property on="Figure_axis" class="Arr (strict)"() -> ("Value"=w338:string[])  [unwired: 2 in, 2 out]
          n296 = property on="data_caption" class="Str"() -> ("Value"=w340:string)  [unwired: 2 in, 2 out]
          n297 = case shown="True" w341 {
            tunnel: w340 -> [w343 w349]
            tunnel: [w343 w348] -> w339
            tunnel: w338 -> [w342 w346]
            tunnel: [w342 w344] -> w337
            frame False {
              # "not measure 2182A 1 channel 2 (2182A_1_ch2)"
            }
            frame True {
              w345 = "2182A_1_ch2"
              # "measure 2182A 1 channel 2 (2182A_1_ch2)"
              n298 = local read "2182A 1 addr"() -> (w350:u8)
              n299 = Number To Decimal String(number=w350) -> (decimal integer string=w351:string)  [unwired: 1 in]
              n300 = GPIB Clear(3:w351) -> ()  [unwired: 1 in, 2 out]
              n301 = Build Array (concatenate)(w346, w345) -> (w344:string[])
              n302 = Concatenate Strings(w349, w345, "\t") -> (w348:string)
            }
          }
          n303 = property on="Figure_axis" class="Arr (strict)"("Value"=w337) -> ()  [unwired: 2 in, 2 out]
          n304 = property on="data_caption" class="Str"("Value"=w339) -> ()  [unwired: 2 in, 2 out]
        }
        frame #18 {
          # "2182A 2 channel 1 measure (2182A_2_ch1)"
          n305 = local read "2182A 2 ch1"() -> (w356:bool)
          n306 = property on="Figure_axis" class="Arr (strict)"() -> ("Value"=w353:string[])  [unwired: 2 in, 2 out]
          n307 = property on="data_caption" class="Str"() -> ("Value"=w355:string)  [unwired: 2 in, 2 out]
          n308 = case shown="True" w356 {
            tunnel: w355 -> [w358 w364]
            tunnel: [w358 w363] -> w354
            tunnel: w353 -> [w357 w361]
            tunnel: [w357 w359] -> w352
            frame False {
              # "not measure 2182A 2 channel 1 (2182A_2_ch1)"
            }
            frame True {
              w360 = "2182A_2_ch1"
              # "measure 2182A 2 channel 1 (2182A_2_ch1)"
              n309 = local read "2182A 2 addr"() -> (w365:u8)
              n310 = Number To Decimal String(number=w365) -> (decimal integer string=w366:string)  [unwired: 1 in]
              n311 = GPIB Clear(3:w366) -> ()  [unwired: 1 in, 2 out]
              n312 = Build Array (concatenate)(w361, w360) -> (w359:string[])
              n313 = Concatenate Strings(w364, w360, "\t") -> (w363:string)
            }
          }
          n314 = property on="Figure_axis" class="Arr (strict)"("Value"=w352) -> ()  [unwired: 2 in, 2 out]
          n315 = property on="data_caption" class="Str"("Value"=w354) -> ()  [unwired: 2 in, 2 out]
        }
        frame #19 {
          # "2182A 2 channel 2 measure (2182A_2_ch2)"
          n316 = local read "2182A 2 ch2"() -> (w371:bool)
          n317 = property on="Figure_axis" class="Arr (strict)"() -> ("Value"=w368:string[])  [unwired: 2 in, 2 out]
          n318 = property on="data_caption" class="Str"() -> ("Value"=w370:string)  [unwired: 2 in, 2 out]
          n319 = case shown="True" w371 {
            tunnel: w370 -> [w373 w379]
            tunnel: [w373 w378] -> w369
            tunnel: w368 -> [w372 w376]
            tunnel: [w372 w374] -> w367
            frame False {
              # "not measure 2182A 2 channel 2 (2182A_2_ch2)"
            }
            frame True {
              w375 = "2182A_2_ch2"
              # "measure 2182A 2 channel 2 (2182A_2_ch2)"
              n320 = local read "2182A 2 addr"() -> (w380:u8)
              n321 = Number To Decimal String(number=w380) -> (decimal integer string=w381:string)  [unwired: 1 in]
              n322 = GPIB Clear(3:w381) -> ()  [unwired: 1 in, 2 out]
              n323 = Build Array (concatenate)(w376, w375) -> (w374:string[])
              n324 = Concatenate Strings(w379, w375, "\t") -> (w378:string)
            }
          }
          n325 = property on="Figure_axis" class="Arr (strict)"("Value"=w367) -> ()  [unwired: 2 in, 2 out]
          n326 = property on="data_caption" class="Str"("Value"=w369) -> ()  [unwired: 2 in, 2 out]
        }
        frame #20 {
          # "2182A 3 channel 1 measure (2182A_3_ch1)"
          n327 = local read "2182A 3 ch1"() -> (w386:bool)
          n328 = property on="Figure_axis" class="Arr (strict)"() -> ("Value"=w383:string[])  [unwired: 2 in, 2 out]
          n329 = property on="data_caption" class="Str"() -> ("Value"=w385:string)  [unwired: 2 in, 2 out]
          n330 = case shown="True" w386 {
            tunnel: w385 -> [w388 w394]
            tunnel: [w388 w393] -> w384
            tunnel: w383 -> [w387 w391]
            tunnel: [w387 w389] -> w382
            frame False {
              # "not measure 2182A 3 channel 1 (2182A_3_ch1)"
            }
            frame True {
              w390 = "2182A_3_ch1"
              # "measure 2182A 3 channel 1 (2182A_3_ch1)"
              n331 = local read "2182A 3 addr"() -> (w395:u8)
              n332 = Number To Decimal String(number=w395) -> (decimal integer string=w396:string)  [unwired: 1 in]
              n333 = GPIB Clear(3:w396) -> ()  [unwired: 1 in, 2 out]
              n334 = Build Array (concatenate)(w391, w390) -> (w389:string[])
              n335 = Concatenate Strings(w394, w390, "\t") -> (w393:string)
            }
          }
          n336 = property on="Figure_axis" class="Arr (strict)"("Value"=w382) -> ()  [unwired: 2 in, 2 out]
          n337 = property on="data_caption" class="Str"("Value"=w384) -> ()  [unwired: 2 in, 2 out]
        }
        frame #21 {
          # "2182A 3 channel 2 measure (2182A_3_ch2)"
          n338 = local read "2182A 3 ch2"() -> (w401:bool)
          n339 = property on="Figure_axis" class="Arr (strict)"() -> ("Value"=w398:string[])  [unwired: 2 in, 2 out]
          n340 = property on="data_caption" class="Str"() -> ("Value"=w400:string)  [unwired: 2 in, 2 out]
          n341 = case shown="False" w401 {
            tunnel: w400 -> [w403 w409]
            tunnel: [w403 w408] -> w399
            tunnel: w398 -> [w402 w406]
            tunnel: [w402 w404] -> w397
            frame False {
              # "not measure 2182A 3 channel 2 (2182A_3_ch2)"
            }
            frame True {
              w405 = "2182A_3_ch2"
              # "measure 2182A 3 channel 2 (2182A_3_ch2)"
              n342 = local read "2182A 3 addr"() -> (w410:u8)
              n343 = Number To Decimal String(number=w410) -> (decimal integer string=w411:string)  [unwired: 1 in]
              n344 = GPIB Clear(3:w411) -> ()  [unwired: 1 in, 2 out]
              n345 = Build Array (concatenate)(w406, w405) -> (w404:string[])
              n346 = Concatenate Strings(w409, w405, "\t") -> (w408:string)
            }
          }
          n347 = property on="Figure_axis" class="Arr (strict)"("Value"=w397) -> ()  [unwired: 2 in, 2 out]
          n348 = property on="data_caption" class="Str"("Value"=w399) -> ()  [unwired: 2 in, 2 out]
        }
        frame #22 {
          # "2182A 4 channel 1 measure (2182A_4_ch1)"
          n349 = local read "2182A 4 ch1"() -> (w416:bool)
          n350 = property on="Figure_axis" class="Arr (strict)"() -> ("Value"=w413:string[])  [unwired: 2 in, 2 out]
          n351 = property on="data_caption" class="Str"() -> ("Value"=w415:string)  [unwired: 2 in, 2 out]
          n352 = case shown="True" w416 {
            tunnel: w415 -> [w418 w424]
            tunnel: [w418 w423] -> w414
            tunnel: w413 -> [w417 w421]
            tunnel: [w417 w419] -> w412
            frame False {
              # "not measure 2182A 4 channel 1 (2182A_4_ch1)"
            }
            frame True {
              w420 = "2182A_4_ch1"
              # "measure 2182A 4 channel 1 (2182A_4_ch1)"
              n353 = local read "2182A 4 addr"() -> (w425:u8)
              n354 = Number To Decimal String(number=w425) -> (decimal integer string=w426:string)  [unwired: 1 in]
              n355 = GPIB Clear(3:w426) -> ()  [unwired: 1 in, 2 out]
              n356 = Build Array (concatenate)(w421, w420) -> (w419:string[])
              n357 = Concatenate Strings(w424, w420, "\t") -> (w423:string)
            }
          }
          n358 = property on="Figure_axis" class="Arr (strict)"("Value"=w412) -> ()  [unwired: 2 in, 2 out]
          n359 = property on="data_caption" class="Str"("Value"=w414) -> ()  [unwired: 2 in, 2 out]
        }
        frame #23 {
          # "2182A 4 channel 2 measure (2182A_4_ch2)"
          n360 = local read "2182A 4 ch2"() -> (w431:bool)
          n361 = property on="Figure_axis" class="Arr (strict)"() -> ("Value"=w428:string[])  [unwired: 2 in, 2 out]
          n362 = property on="data_caption" class="Str"() -> ("Value"=w430:string)  [unwired: 2 in, 2 out]
          n363 = case shown="True" w431 {
            tunnel: w430 -> [w433 w439]
            tunnel: [w433 w438] -> w429
            tunnel: w428 -> [w432 w436]
            tunnel: [w432 w434] -> w427
            frame False {
              # "not measure 2182A 4 channel 2 (2182A_4_ch2)"
            }
            frame True {
              w435 = "2182A_4_ch2"
              # "measure 2182A 4 channel 2 (2182A_4_ch2)"
              n364 = local read "2182A 4 addr"() -> (w440:u8)
              n365 = Number To Decimal String(number=w440) -> (decimal integer string=w441:string)  [unwired: 1 in]
              n366 = GPIB Clear(3:w441) -> ()  [unwired: 1 in, 2 out]
              n367 = Build Array (concatenate)(w436, w435) -> (w434:string[])
              n368 = Concatenate Strings(w439, w435, "\t") -> (w438:string)
            }
          }
          n369 = property on="Figure_axis" class="Arr (strict)"("Value"=w427) -> ()  [unwired: 2 in, 2 out]
          n370 = property on="data_caption" class="Str"("Value"=w429) -> ()  [unwired: 2 in, 2 out]
        }
        frame #24 {
          # "2636A smua measure voltage (2636A_smua_v)"
          n371 = local read "2636A smua meas v"() -> (w446:bool)
          n372 = property on="Figure_axis" class="Arr (strict)"() -> ("Value"=w443:string[])  [unwired: 2 in, 2 out]
          n373 = property on="data_caption" class="Str"() -> ("Value"=w445:string)  [unwired: 2 in, 2 out]
          n374 = case shown="True" w446 {
            tunnel: w445 -> [w448 w459]
            tunnel: [w448 w458] -> w444
            tunnel: w443 -> [w447 w456]
            tunnel: [w447 w454] -> w442
            frame False {
              # "not measure voltage on 2636A smua (2636A_smua_v)"
            }
            frame True {
              w455 = "2636A_smua_v"
              # "measure voltage on 2636A smua (2636A_smua_v)"
              n375 = local read "2336A addr"() -> (w450:refnum<visa-resource-name>)
              n376 = VISA Open(VISA resource name=w450) -> (VISA resource name=w449:refnum<visa-resource-name>, error out=w451:errorcluster)  [unwired: 4 in]
              n377 = VISA Clear(VISA resource name=w449, error in (no error)=w451) -> (VISA resource name out=w453:refnum<visa-resource-name>)  [unwired: 1 out]
              n378 = property class="Instr"(reference=w453, "General Settings:Timeout Value"=u32 10000) -> ()  [unwired: 1 in, 2 out]
              n379 = Build Array (concatenate)(w456, w455) -> (w454:string[])
              n380 = Concatenate Strings(w459, w455, "\t") -> (w458:string)
            }
          }
          n381 = property on="Figure_axis" class="Arr (strict)"("Value"=w442) -> ()  [unwired: 2 in, 2 out]
          n382 = property on="data_caption" class="Str"("Value"=w444) -> ()  [unwired: 2 in, 2 out]
        }
        frame #25 {
          # "2636A smua measure current (2636A_smua_i)"
          n383 = local read "2636A smua meas i"() -> (w464:bool)
          n384 = property on="Figure_axis" class="Arr (strict)"() -> ("Value"=w461:string[])  [unwired: 2 in, 2 out]
          n385 = property on="data_caption" class="Str"() -> ("Value"=w463:string)  [unwired: 2 in, 2 out]
          n386 = case shown="True" w464 {
            tunnel: w463 -> [w466 w477]
            tunnel: [w466 w476] -> w462
            tunnel: w461 -> [w465 w474]
            tunnel: [w465 w472] -> w460
            frame False {
              # "not measure current on 2636A smua (2636A_smua_i)"
            }
            frame True {
              w473 = "2636A_smua_i"
              # "measure current on 2636A smua (2636A_smua_i)"
              n387 = local read "2336A addr"() -> (w469:refnum<visa-resource-name>)
              n388 = VISA Open(VISA resource name=w469) -> (VISA resource name=w468:refnum<visa-resource-name>, error out=w467:errorcluster)  [unwired: 4 in]
              n389 = VISA Clear(VISA resource name=w468, error in (no error)=w467) -> (VISA resource name out=w470:refnum<visa-resource-name>)  [unwired: 1 out]
              n390 = Build Array (concatenate)(w474, w473) -> (w472:string[])
              n391 = property class="Instr"(reference=w470, "General Settings:Timeout Value"=u32 10000) -> ()  [unwired: 1 in, 2 out]
              n392 = Concatenate Strings(w477, w473, "\t") -> (w476:string)
            }
          }
          n393 = property on="Figure_axis" class="Arr (strict)"("Value"=w460) -> ()  [unwired: 2 in, 2 out]
          n394 = property on="data_caption" class="Str"("Value"=w462) -> ()  [unwired: 2 in, 2 out]
        }
        frame #26 {
          # "2636A smub measure voltage (2636A_smub_v)"
          n395 = local read "2636A smub meas v"() -> (w482:bool)
          n396 = property on="Figure_axis" class="Arr (strict)"() -> ("Value"=w479:string[])  [unwired: 2 in, 2 out]
          n397 = property on="data_caption" class="Str"() -> ("Value"=w481:string)  [unwired: 2 in, 2 out]
          n398 = case shown="True" w482 {
            tunnel: w481 -> [w484 w495]
            tunnel: [w484 w494] -> w480
            tunnel: w479 -> [w483 w492]
            tunnel: [w483 w490] -> w478
            frame False {
              # "not measure voltage on 2636A smub (2636A_smub_v)"
            }
            frame True {
              w491 = "2636A_smub_v"
              # "measure voltage on 2636A smub (2636A_smub_v)"
              n399 = local read "2336A addr"() -> (w486:refnum<visa-resource-name>)
              n400 = VISA Open(VISA resource name=w486) -> (VISA resource name=w485:refnum<visa-resource-name>, error out=w487:errorcluster)  [unwired: 4 in]
              n401 = VISA Clear(VISA resource name=w485, error in (no error)=w487) -> (VISA resource name out=w488:refnum<visa-resource-name>)  [unwired: 1 out]
              n402 = Build Array (concatenate)(w492, w491) -> (w490:string[])
              n403 = property class="Instr"(reference=w488, "General Settings:Timeout Value"=u32 10000) -> ()  [unwired: 1 in, 2 out]
              n404 = Concatenate Strings(w495, w491, "\t") -> (w494:string)
            }
          }
          n405 = property on="Figure_axis" class="Arr (strict)"("Value"=w478) -> ()  [unwired: 2 in, 2 out]
          n406 = property on="data_caption" class="Str"("Value"=w480) -> ()  [unwired: 2 in, 2 out]
        }
        frame #27 {
          # "2636A smub measure current (2636A_smub_i)"
          n407 = local read "2636A smub meas i"() -> (w500:bool)
          n408 = property on="Figure_axis" class="Arr (strict)"() -> ("Value"=w497:string[])  [unwired: 2 in, 2 out]
          n409 = property on="data_caption" class="Str"() -> ("Value"=w499:string)  [unwired: 2 in, 2 out]
          n410 = case shown="True" w500 {
            tunnel: w499 -> [w502 w513]
            tunnel: [w502 w512] -> w498
            tunnel: w497 -> [w501 w510]
            tunnel: [w501 w508] -> w496
            frame False {
              # "not measure current on 2636A smub (2636A_smub_i)"
            }
            frame True {
              w509 = "2636A_smub_i"
              # "measure current on 2636A smub (2636A_smub_i)"
              n411 = local read "2336A addr"() -> (w503:refnum<visa-resource-name>)
              n412 = VISA Open(VISA resource name=w503) -> (VISA resource name=w504:refnum<visa-resource-name>, error out=w505:errorcluster)  [unwired: 4 in]
              n413 = VISA Clear(VISA resource name=w504, error in (no error)=w505) -> (VISA resource name out=w506:refnum<visa-resource-name>)  [unwired: 1 out]
              n414 = Build Array (concatenate)(w510, w509) -> (w508:string[])
              n415 = property class="Instr"(reference=w506, "General Settings:Timeout Value"=u32 10000) -> ()  [unwired: 1 in, 2 out]
              n416 = Concatenate Strings(w513, w509, "\t") -> (w512:string)
            }
          }
          n417 = property on="Figure_axis" class="Arr (strict)"("Value"=w496) -> ()  [unwired: 2 in, 2 out]
          n418 = property on="data_caption" class="Str"("Value"=w498) -> ()  [unwired: 2 in, 2 out]
        }
        frame #28 {
          # "presision capacitance bridge AH2500 measure capacitance and loss (AH2500_c) and (AH2500_l)"
          n419 = local read "AH2500 C and L"() -> (w518:bool)
          n420 = property on="Figure_axis" class="Arr (strict)"() -> ("Value"=w515:string[])  [unwired: 2 in, 2 out]
          n421 = property on="data_caption" class="Str"() -> ("Value"=w517:string)  [unwired: 2 in, 2 out]
          n422 = case shown="True" w518 {
            tunnel: w517 -> [w520 w527]
            tunnel: [w520 w526] -> w516
            tunnel: w515 -> [w519 w525]
            tunnel: [w519 w523] -> w514
            frame False {
              # "AH2700A measure neither capacitance (AH2700A_c)\nnor loss (AH2700A_l)"
            }
            frame True {
              w522 = "AH2500_l"
              w521 = "\t"
              w524 = "AH2500_c"
              # "measure AH2500 capacitance and loss \n(AH2500_c) and/or (AH2500_l)"
              n423 = local read "AH2500 addr"() -> (w528:u8)
              n424 = Number To Decimal String(number=w528) -> (decimal integer string=w529:string)  [unwired: 1 in]
              n425 = GPIB Clear(3:w529) -> ()  [unwired: 1 in, 2 out]
              n426 = Build Array (concatenate)(w525, w524, w522) -> (w523:string[])
              n427 = Concatenate Strings(w527, w524, w521, w522, w521) -> (w526:string)
            }
          }
          n428 = property on="Figure_axis" class="Arr (strict)"("Value"=w514) -> ()  [unwired: 2 in, 2 out]
          n429 = property on="data_caption" class="Str"("Value"=w516) -> ()  [unwired: 2 in, 2 out]
        }
        frame #29 {
          # "presision capacitance bridge AH2700A measure capacitance and loss (AH2700A_c) and (AH2700A_l)"
          n430 = local read "AH2700A C and L"() -> (w530:bool)
          n431 = property on="Figure_axis" class="Arr (strict)"() -> ("Value"=w532:string[])  [unwired: 2 in, 2 out]
          n432 = property on="data_caption" class="Str"() -> ("Value"=w534:string)  [unwired: 2 in, 2 out]
          n433 = case shown="True" w530 {
            tunnel: w534 -> [w536 w543]
            tunnel: [w536 w542] -> w533
            tunnel: w532 -> [w535 w541]
            tunnel: [w535 w539] -> w531
            frame False {
              # "AH2700A measure neither capacitance (AH2700A_c)\nnor loss (AH2700A_l)"
            }
            frame True {
              w538 = "AH2700A_l"
              w537 = "\t"
              w540 = "AH2700A_c"
              # "measure AH2700A capacitance and loss \n(AH2700A_c) and/or (AH2700A_l)"
              n434 = local read "AH2700A addr"() -> (w544:u8)
              n435 = Number To Decimal String(number=w544) -> (decimal integer string=w545:string)  [unwired: 1 in]
              n436 = GPIB Clear(3:w545) -> ()  [unwired: 1 in, 2 out]
              n437 = Build Array (concatenate)(w541, w540, w538) -> (w539:string[])
              n438 = Concatenate Strings(w543, w540, w537, w538, w537) -> (w542:string)
            }
          }
          n439 = property on="Figure_axis" class="Arr (strict)"("Value"=w531) -> ()  [unwired: 2 in, 2 out]
          n440 = property on="data_caption" class="Str"("Value"=w533) -> ()  [unwired: 2 in, 2 out]
        }
        frame #30 {
          # "measure temperature in K on LS340 input A (LS340_A)"
          n441 = local read "LS340 A"() -> (w546:bool)
          n442 = property on="Figure_axis" class="Arr (strict)"() -> ("Value"=w548:string[])  [unwired: 2 in, 2 out]
          n443 = property on="data_caption" class="Str"() -> ("Value"=w550:string)  [unwired: 2 in, 2 out]
          n444 = case shown="True" w546 {
            tunnel: w550 -> [w552 w558]
            tunnel: [w552 w557] -> w549
            tunnel: w548 -> [w551 w556]
            tunnel: [w551 w554] -> w547
            frame False {
              # "do not measure temperature in K on LS340 input A (LS340_A)"
            }
            frame True {
              w555 = "LS340_A"
              # "measure temperature in K on LS340 input A (LS340_A)"
              n445 = local read "LS340 addr"() -> (w559:u8)
              n446 = Number To Decimal String(number=w559) -> (decimal integer string=w560:string)  [unwired: 1 in]
              n447 = GPIB Clear(3:w560) -> ()  [unwired: 1 in, 2 out]
              n448 = Build Array (concatenate)(w556, w555) -> (w554:string[])
              n449 = Concatenate Strings(w558, w555, "\t") -> (w557:string)
            }
          }
          n450 = property on="Figure_axis" class="Arr (strict)"("Value"=w547) -> ()  [unwired: 2 in, 2 out]
          n451 = property on="data_caption" class="Str"("Value"=w549) -> ()  [unwired: 2 in, 2 out]
        }
        frame #31 {
          # "measure temperature in K on LS340 input B (LS340_B)"
          n452 = local read "LS340 B"() -> (w561:bool)
          n453 = property on="Figure_axis" class="Arr (strict)"() -> ("Value"=w563:string[])  [unwired: 2 in, 2 out]
          n454 = property on="data_caption" class="Str"() -> ("Value"=w565:string)  [unwired: 2 in, 2 out]
          n455 = case shown="True" w561 {
            tunnel: w565 -> [w567 w573]
            tunnel: [w567 w572] -> w564
            tunnel: w563 -> [w566 w571]
            tunnel: [w566 w569] -> w562
            frame False {
              # "do not measure temperature in K on LS340 input B (LS340_B)"
            }
            frame True {
              w570 = "LS340_B"
              # "measure temperature in K on LS340 input B (LS340_B)"
              n456 = local read "LS340 addr"() -> (w574:u8)
              n457 = Number To Decimal String(number=w574) -> (decimal integer string=w575:string)  [unwired: 1 in]
              n458 = GPIB Clear(3:w575) -> ()  [unwired: 1 in, 2 out]
              n459 = Build Array (concatenate)(w571, w570) -> (w569:string[])
              n460 = Concatenate Strings(w573, w570, "\t") -> (w572:string)
            }
          }
          n461 = property on="Figure_axis" class="Arr (strict)"("Value"=w562) -> ()  [unwired: 2 in, 2 out]
          n462 = property on="data_caption" class="Str"("Value"=w564) -> ()  [unwired: 2 in, 2 out]
        }
        frame #32 {
          # "measure temperature in K on LS332 input A (LS332_A)"
          n463 = local read "LS332 A"() -> (w576:bool)
          n464 = property on="Figure_axis" class="Arr (strict)"() -> ("Value"=w578:string[])  [unwired: 2 in, 2 out]
          n465 = property on="data_caption" class="Str"() -> ("Value"=w580:string)  [unwired: 2 in, 2 out]
          n466 = case shown="True" w576 {
            tunnel: w580 -> [w582 w588]
            tunnel: [w582 w587] -> w579
            tunnel: w578 -> [w581 w586]
            tunnel: [w581 w584] -> w577
            frame False {
              # "do not measure temperature in K on LS332 input A (LS332_A)"
            }
            frame True {
              w585 = "LS332_A"
              # "measure temperature in K on LS332 input A (LS332_A)"
              n467 = local read "LS332 addr"() -> (w589:u8)
              n468 = Number To Decimal String(number=w589) -> (decimal integer string=w590:string)  [unwired: 1 in]
              n469 = GPIB Clear(3:w590) -> ()  [unwired: 1 in, 2 out]
              n470 = Build Array (concatenate)(w586, w585) -> (w584:string[])
              n471 = Concatenate Strings(w588, w585, "\t") -> (w587:string)
            }
          }
          n472 = property on="Figure_axis" class="Arr (strict)"("Value"=w577) -> ()  [unwired: 2 in, 2 out]
          n473 = property on="data_caption" class="Str"("Value"=w579) -> ()  [unwired: 2 in, 2 out]
        }
        frame #33 {
          # "measure temperature in K on LS332 input B (LS332_B)"
          n474 = local read "LS332 B"() -> (w591:bool)
          n475 = property on="Figure_axis" class="Arr (strict)"() -> ("Value"=w593:string[])  [unwired: 2 in, 2 out]
          n476 = property on="data_caption" class="Str"() -> ("Value"=w595:string)  [unwired: 2 in, 2 out]
          n477 = case shown="True" w591 {
            tunnel: w595 -> [w597 w603]
            tunnel: [w597 w602] -> w594
            tunnel: w593 -> [w596 w601]
            tunnel: [w596 w599] -> w592
            frame False {
              # "do not measure temperature in K on LS332 input B (LS332_B)"
            }
            frame True {
              w600 = "LS332_B"
              # "measure temperature in K on LS332 input B (LS332_B)"
              n478 = local read "LS332 addr"() -> (w604:u8)
              n479 = Number To Decimal String(number=w604) -> (decimal integer string=w605:string)  [unwired: 1 in]
              n480 = GPIB Clear(3:w605) -> ()  [unwired: 1 in, 2 out]
              n481 = Build Array (concatenate)(w601, w600) -> (w599:string[])
              n482 = Concatenate Strings(w603, w600, "\t") -> (w602:string)
            }
          }
          n483 = property on="Figure_axis" class="Arr (strict)"("Value"=w592) -> ()  [unwired: 2 in, 2 out]
          n484 = property on="data_caption" class="Str"("Value"=w594) -> ()  [unwired: 2 in, 2 out]
        }
        frame #34 {
          # "measure time"
          n485 = local read "measure time"() -> (w610:bool)
          n486 = property on="Figure_axis" class="Arr (strict)"() -> ("Value"=w607:string[])  [unwired: 2 in, 2 out]
          n487 = property on="data_caption" class="Str"() -> ("Value"=w609:string)  [unwired: 2 in, 2 out]
          n488 = case shown="True" w610 {
            tunnel: w609 -> [w612 w618]
            tunnel: [w612 w617] -> w608
            tunnel: w607 -> [w611 w615]
            tunnel: [w611 w613] -> w606
            frame False {
              # "not measuring time"
            }
            frame True {
              w614 = "time"
              # "measuring time"
              n489 = Build Array (concatenate)(w615, w614) -> (w613:string[])
              n490 = Concatenate Strings(w618, w614, "\t") -> (w617:string)
            }
          }
          n491 = property on="Figure_axis" class="Arr (strict)"("Value"=w606) -> ()  [unwired: 2 in, 2 out]
          n492 = property on="data_caption" class="Str"("Value"=w608) -> ()  [unwired: 2 in, 2 out]
        }
        frame #35 {
          # "2182A 5 channel 1 to measure HULK SMS field"
          n493 = local read "Hulk_B_meas (Vnano)"() -> (w623:bool)
          n494 = property on="Figure_axis" class="Arr (strict)"() -> ("Value"=w620:string[])  [unwired: 2 in, 2 out]
          n495 = property on="data_caption" class="Str"() -> ("Value"=w622:string)  [unwired: 2 in, 2 out]
          n496 = case shown="True" w623 {
            tunnel: w622 -> [w625 w631]
            tunnel: [w625 w630] -> w621
            tunnel: w620 -> [w624 w628]
            tunnel: [w624 w626] -> w619
            frame False {
              # "do not use 2182A 5 channel 1 to measure HULK SMS field"
            }
            frame True {
              w627 = "HULK_SMS_field"
              # "use 2182A 5 channel 1 to measure HULK SMS field"
              n497 = local read "2182A 5 addr"() -> (w632:u8)
              n498 = Number To Decimal String(number=w632) -> (decimal integer string=w633:string)  [unwired: 1 in]
              n499 = GPIB Clear(3:w633) -> ()  [unwired: 1 in, 2 out]
              n500 = Build Array (concatenate)(w628, w627) -> (w626:string[])
              n501 = Concatenate Strings(w631, w627, "\t") -> (w630:string)
            }
          }
          n502 = property on="Figure_axis" class="Arr (strict)"("Value"=w619) -> ()  [unwired: 2 in, 2 out]
          n503 = property on="data_caption" class="Str"("Value"=w621) -> ()  [unwired: 2 in, 2 out]
        }
        frame #36 {
          # "Measure magnetic field on IPS120-0"
          n504 = local read "MercuryIPS"() -> (w638:bool)
          n505 = property on="Figure_axis" class="Arr (strict)"() -> ("Value"=w635:string[])  [unwired: 2 in, 2 out]
          n506 = property on="data_caption" class="Str"() -> ("Value"=w637:string)  [unwired: 2 in, 2 out]
          n507 = case shown="True" w638 {
            tunnel: w637 -> [w640 w646]
            tunnel: [w640 w645] -> w636
            tunnel: w635 -> [w639 w643]
            tunnel: [w639 w641] -> w634
            frame False {
              # "do not Measure magnetic field on MercuryIPS"
            }
            frame True {
              w642 = "MercuryIPS_Field"
              # "Measure magnetic field on MercuryIPS"
              n508 = Build Array (concatenate)(w643, w642) -> (w641:string[])
              n509 = Concatenate Strings(w646, w642, "\t") -> (w645:string)
            }
          }
          n510 = property on="Figure_axis" class="Arr (strict)"("Value"=w634) -> ()  [unwired: 2 in, 2 out]
          n511 = property on="data_caption" class="Str"("Value"=w636) -> ()  [unwired: 2 in, 2 out]
        }
        frame #37 {
          # "measure capacitance with LT bridge"
          n512 = local read "LT bridge\ncalibration"() -> (w650:bool)
          n513 = local read "LT bridge"() -> (w648:bool)
          n514 = property on="Figure_axis" class="Arr (strict)"() -> ("Value"=w652:string[])  [unwired: 2 in, 2 out]
          n515 = property on="data_caption" class="Str"() -> ("Value"=w654:string)  [unwired: 2 in, 2 out]
          n516 = Not(x=w650) -> (.not. x?=w649:bool)
          n517 = And(x=w649, y=w648) -> (x .and. y?=w647:bool)
          n518 = case shown="True" w647 {
            tunnel: w654 -> [w656 w662]
            tunnel: [w656 w661] -> w653
            tunnel: w652 -> [w655 w659]
            tunnel: [w655 w657] -> w651
            frame False {
              # "not measuring capacitance with LT bridge"
            }
            frame True {
              w658 = "LT_bridge"
              # "measuring capacitance with LT bridge"
              n519 = Build Array (concatenate)(w659, w658) -> (w657:string[])
              n520 = Concatenate Strings(w662, w658, "\t") -> (w661:string)
            }
          }
          n521 = property on="Figure_axis" class="Arr (strict)"("Value"=w651) -> ()  [unwired: 2 in, 2 out]
          n522 = property on="data_caption" class="Str"("Value"=w653) -> ()  [unwired: 2 in, 2 out]
        }
        frame #38 {
          # "measure DC resistance"
          n523 = property on="Figure_axis" class="Arr (strict)"() -> ("Value"=w667:string[])  [unwired: 2 in, 2 out]
          n524 = property on="data_caption" class="Str"() -> ("Value"=w664:string)  [unwired: 2 in, 2 out]
          n525 = local read "DC_resistance"() -> (w665:bool)
          n526 = call "DCcommuteLabels.vi"("2182A 4"="2182A 4", "2182A 2"="2182A 2", "2182A 3"="2182A 3", "2182A 1"="2182A 1", "DC_resistance"=w665, "FigureCaptionsIn"=w667, "AxesCaptionsIn"=w664) -> ("FigureCaptionsOut"=w666:string[], "AxesCaptionsOut"=w663:string)  [unwired: 3 in]
          n527 = property on="data_caption" class="Str"("Value"=w663) -> ()  [unwired: 2 in, 2 out]
          n528 = property on="Figure_axis" class="Arr (strict)"("Value"=w666) -> ()  [unwired: 2 in, 2 out]
        }
      }
      n529 = stacked-sequence {
        tunnel: w79 -> [_]
        frame #0 {
          n530 = Wait (ms)(milliseconds to wait=u32 300) -> ()  [unwired: 1 out]
        }
      }
    }
    frame #3 {
      # "1 = 2400 1\n2 = 2400 2\n3 = 2400 3\n4 = 2636a smua\n5 = 2636a smub\n6 = do not sweep, just time\n7 = HULK SMS"
      n531 = local read "sweep"() -> (w673:T3)
      n532 = case "reads current value from instrument which will be sweeping" shown="\"Radio Selection 5\"" w673 {
        tunnel: [w674 w683 w692 w701 w705 0.0 ("Measuremet") w710 w786] -> w672
        frame "Radio Selection 1", Default {
          # "reads the voltage on 2400 1"
          n533 = local read "2400 1 addr"() -> (w678:u8)
          n534 = Number To Decimal String(number=w678) -> (decimal integer string=w679:string)  [unwired: 1 in]
          n535 = GPIB Write(0:w679, 1:":READ?") -> (6:w675:errorcluster)  [unwired: 3 in, 1 out]
          n536 = GPIB Read(0:w679, 1:3200, 3:w675) -> (5:w681:string)  [unwired: 2 in, 2 out]
          n537 = String Subset(string=w681, length (rest)=13) -> (substring=w682:string)  [unwired: 1 in]
          n538 = Fract/Exp String To Number(string=w682) -> (number=w674:dbl)  [unwired: 3 in, 1 out]
        }
        frame "Radio Selection 2" {
          # "reads the voltage on 2400 2"
          n539 = local read "2400 2 addr"() -> (w687:u8)
          n540 = Number To Decimal String(number=w687) -> (decimal integer string=w688:string)  [unwired: 1 in]
          n541 = GPIB Write(0:w688, 1:":READ?") -> (6:w684:errorcluster)  [unwired: 3 in, 1 out]
          n542 = GPIB Read(0:w688, 1:3200, 3:w684) -> (5:w690:string)  [unwired: 2 in, 2 out]
          n543 = String Subset(string=w690, length (rest)=13) -> (substring=w691:string)  [unwired: 1 in]
          n544 = Fract/Exp String To Number(string=w691) -> (number=w683:dbl)  [unwired: 3 in, 1 out]
        }
        frame "Radio Selection 3" {
          # "reads the voltage on 2400 3"
          n545 = local read "2400 3 addr"() -> (w696:u8)
          n546 = Number To Decimal String(number=w696) -> (decimal integer string=w697:string)  [unwired: 1 in]
          n547 = GPIB Write(0:w697, 1:":READ?") -> (6:w693:errorcluster)  [unwired: 3 in, 1 out]
          n548 = GPIB Read(0:w697, 1:3200, 3:w693) -> (5:w699:string)  [unwired: 2 in, 2 out]
          n549 = String Subset(string=w699, length (rest)=13) -> (substring=w700:string)  [unwired: 1 in]
          n550 = Fract/Exp String To Number(string=w700) -> (number=w692:dbl)  [unwired: 3 in, 1 out]
        }
        frame "Radio Selection 4" {
          # "reads the voltage on 2636a smua"
          n551 = local read "2336A addr"() -> (w704:refnum<visa-resource-name>)
          n552 = call "SinglePointMeasurement.vi"("Measure"=Measure."Voltage", "Channel"=Channel."a", "VISA resource name 2"=w704) -> ("Measuremet"=w701:dbl)  [unwired: 3 in, 4 out]
        }
        frame "Radio Selection 5" {
          # "reads the voltage on 2636a smub"
          n553 = local read "2336A addr"() -> (w708:refnum<visa-resource-name>)
          n554 = call "SinglePointMeasurement.vi"("Measure"=Measure."Voltage", "Channel"=Channel."b", "VISA resource name 2"=w708) -> ("Measuremet"=w705:dbl)  [unwired: 3 in, 4 out]
        }
        frame "Radio Selection 6" {
        }
        frame "Radio Selection 7" {
          # "preparing HULK SMS!"
          n555 = stacked-sequence {
            tunnel: [_ _ _ _ _ _ _ w768 _] -> w710
            frame #0 {
              # "initialize interface of HULK SMS"
              n556 = local read "Hulk_SMS_addr"() -> (w717:refnum<visa-resource-name>)
              n557 = VISA Open(VISA resource name=w717) -> (VISA resource name=w716:refnum<visa-resource-name>, error out=w715:errorcluster)  [unwired: 4 in]
              n558 = VISA Clear(VISA resource name=w716, error in (no error)=w715) -> (VISA resource name out=w713:refnum<visa-resource-name>, error out=w712:errorcluster)
              n559 = property class="Instr"(reference=w713, error in=w712, "General Settings:Timeout Value"=u32 2000) -> (error out=w711:errorcluster)  [unwired: 1 out]
              n560 = local write "CRYogenic:("(w711) -> ()
            }
            frame #1 {
              w718 = SMScontrols."UPDATE" ("SMS controls")
              # "check intialization"
              n561 = local read "Hulk_SMS_addr"() -> (w722:refnum<visa-resource-name>)
              n562 = local read "CRYogenic:("() -> (w721:errorcluster)
              n563 = call "SMSsendCommand.vi"("HULK SMS address in"=w722, "SMS controls"=w718, "error in"=w721) -> ("HULK SMS address out"=w723:refnum<visa-resource-name>, "error out"=w724:errorcluster)  [unwired: 14 in, 1 out]
              n564 = call "WaitRS232.vi"("error in"=w724, "delay[160 ms]"=u32 1000) -> ("error out"=w726:errorcluster)  [unwired: 1 in]
              n565 = call "SMSread.vi"("HULK SMS address in"=w723, "SMS controls"=w718, "error in"=w726) -> ("read buffer"=w719:string, "error out"=w720:errorcluster)  [unwired: 11 in, 4 out]
              n566 = local write "Word from HULK!"(w719) -> ()
              n567 = local write "CRYogenic:("(w720) -> ()
            }
            frame #2 {
              n568 = Wait (ms)(milliseconds to wait=u32 200) -> ()  [unwired: 1 out]
            }
            frame #3 {
              w728 = SMScontrols."TESLA ON" ("SMS controls")
              # "set units to tesla"
              n569 = local read "Hulk_SMS_addr"() -> (w732:refnum<visa-resource-name>)
              n570 = local read "CRYogenic:("() -> (w731:errorcluster)
              n571 = call "SMSsendCommand.vi"("HULK SMS address in"=w732, "SMS controls"=w728, "error in"=w731) -> ("HULK SMS address out"=w733:refnum<visa-resource-name>, "error out"=w734:errorcluster)  [unwired: 14 in, 1 out]
              n572 = call "WaitRS232.vi"("error in"=w734, "delay[160 ms]"=u32 1000) -> ("error out"=w736:errorcluster)  [unwired: 1 in]
              n573 = call "SMSread.vi"("HULK SMS address in"=w733, "SMS controls"=w728, "error in"=w736) -> ("read buffer"=w729:string, "error out"=w730:errorcluster)  [unwired: 11 in, 4 out]
              n574 = local write "Word from HULK!"(w729) -> ()
              n575 = local write "CRYogenic:("(w730) -> ()
            }
            frame #4 {
              w737 = T6."Disabled and Grayed Out" ("Disabled")
              # "sorry, no control of sweep rate and target\nvalue during sweeping\n\n!!! do not forget to reactivate it in the PAUSE mode!!!"
              n576 = property on="sweep to:" class="DigNum (strict)"("DisabledEnum"=w737) -> ()  [unwired: 2 in, 2 out]
              n577 = property on="sweep rate, /min" class="DigNum (strict)"("DisabledEnum"=w737) -> ()  [unwired: 2 in, 2 out]
            }
            frame #5 {
              w741 = SMScontrols."SET RAMP" ("SMS controls")
              # "actual sweep rate"
              # "1sec delay\nbecause HULK is not very bright"
              # "sets sweep rate for HULK SMS"
              n578 = local read "sweep rate, /min"() -> (w755:dbl)
              n579 = local read "Hulk_SMS_addr"() -> (w754:refnum<visa-resource-name>)
              n580 = local read "CRYogenic:("() -> (w752:errorcluster)
              n581 = call "SweepRateConversion.vi"("RAMP rate in"=w755, "T/min to A/s (True)"=TRUE) -> ("RAMP rate out"=w753:dbl)
              n582 = call "SMSsendCommand.vi"("HULK SMS address in"=w754, "SMS controls"=w741, "error in"=w752, "RAMP rate"=w753) -> ("HULK SMS address out"=w748:refnum<visa-resource-name>, "error out"=w749:errorcluster)  [unwired: 13 in, 1 out]
              n583 = call "WaitRS232.vi"("error in"=w749, "delay[160 ms]"=u32 1000) -> ("error out"=w751:errorcluster)  [unwired: 1 in]
              n584 = call "SMSread.vi"("HULK SMS address in"=w748, "SMS controls"=w741, "error in"=w751) -> ("read buffer"=w744:string, "error out"=w745:errorcluster)  [unwired: 11 in, 4 out]
              n585 = Match Pattern(string=w744, regular expression="RAMP RATE:") -> (after substring=w747:string)  [unwired: 1 in, 3 out]
              n586 = local write "Word from HULK!"(w744) -> ()
              n587 = Scan From String(format string="%.f", input string=w747, error in=w745) -> (error out=w742:errorcluster, output 1=w740:dbl)  [unwired: 2 in, 2 out]
              n588 = local write "CRYogenic:("(w742) -> ()
              n589 = call "SweepRateConversion.vi"("RAMP rate in"=w740, "T/min to A/s (True)"=FALSE) -> ("RAMP rate out"=w738:dbl)
              n590 = local write "sweep rate, /min"(w738) -> ()
            }
            frame #6 {
              w757 = SMScontrols."SET MID" ("SMS controls")
              # "sets target value for B field sweep"
              n591 = local read "Hulk_SMS_addr"() -> (w760:refnum<visa-resource-name>)
              n592 = local read "CRYogenic:("() -> (w761:errorcluster)
              n593 = local read "sweep to:"() -> (w759:dbl)
              n594 = call "SMSsendCommand.vi"("HULK SMS address in"=w760, "SMS controls"=w757, "error in"=w761, "MID field value"=w759) -> ("HULK SMS address out"=w765:refnum<visa-resource-name>, "error out"=w763:errorcluster)  [unwired: 13 in, 1 out]
              n595 = call "WaitRS232.vi"("error in"=w763, "delay[160 ms]"=u32 1000) -> ("error out"=w764:errorcluster)  [unwired: 1 in]
              n596 = call "SMSread.vi"("HULK SMS address in"=w765, "SMS controls"=w757, "error in"=w764) -> ("read buffer"=w758:string, "error out"=w762:errorcluster)  [unwired: 11 in, 4 out]
              n597 = local write "CRYogenic:("(w762) -> ()
              n598 = local write "Word from HULK!"(w758) -> ()
            }
            frame #7 {
              # "acquires current output value"
              n599 = local read "Hulk_SMS_addr"() -> (w771:refnum<visa-resource-name>)
              n600 = local read "CRYogenic:("() -> (w770:errorcluster)
              n601 = call "SMS_GET_OUTPUT.vi"("CRYogenic:("=w770, "Hulk_SMS_addr"=w771) -> ("error IO"=w767:errorcluster, "read buffer"=w769:string, "Numeric"=w768:dbl)
              n602 = local write "Word from HULK!"(w769) -> ()
              n603 = local write "CRYogenic:("(w767) -> ()
            }
            frame #8 {
              # "activates ramping"
              n604 = local read "sweep to:"() -> (w779:dbl)
              n605 = Equal?(x=w779, y=0.0) -> (x = y?=w777:bool)
              n606 = Select(t=SMScontrols."RAMP ZERO" ("SMS controls"), s=w777, f=SMScontrols."RAMP MID" ("SMS controls")) -> (s? t:f=w774:T5)
              n607 = local read "Hulk_SMS_addr"() -> (w781:refnum<visa-resource-name>)
              n608 = local read "CRYogenic:("() -> (w780:errorcluster)
              n609 = call "SMSsendCommand.vi"("HULK SMS address in"=w781, "SMS controls"=w774, "error in"=w780) -> ("HULK SMS address out"=w784:refnum<visa-resource-name>, "error out"=w783:errorcluster)  [unwired: 14 in, 1 out]
              n610 = call "WaitRS232.vi"("error in"=w783, "delay[160 ms]"=u32 1000) -> ("error out"=w785:errorcluster)  [unwired: 1 in]
              n611 = call "SMSread.vi"("HULK SMS address in"=w784, "SMS controls"=w774, "error in"=w785) -> ("read buffer"=w772:string, "error out"=w773:errorcluster)  [unwired: 11 in, 4 out]
              n612 = local write "Word from HULK!"(w772) -> ()
              n613 = local write "CRYogenic:("(w773) -> ()
            }
          }
        }
        frame "Radio Selection 8" {
          n614 = local read "MercuryIPS"() -> (w788:refnum<visa-resource-name>)
          n615 = VISA Clear(VISA resource name=w788) -> (VISA resource name out=w792:refnum<visa-resource-name>, error out=w791:errorcluster)  [unwired: 1 in]
          n616 = Concatenate Strings("READ:DEV:GRPZ:PSU" ("string"), "\r", "\n") -> (w801:string)
          n617 = VISA Write(VISA resource name=w792, write buffer=w801, error in (no error)=w791) -> (VISA resource name out=w793:refnum<visa-resource-name>, error out=w794:errorcluster)  [unwired: 1 out]
          n618 = VISA Read(VISA resource name=w793, byte count=u32 450, error in (no error)=w794) -> (read buffer=w787:string, error out=w789:errorcluster)  [unwired: 2 out]
          n619 = Match Pattern(string=w787, regular expression=":PCUR:") -> (after substring=w797:string)  [unwired: 1 in, 3 out]
          n620 = Match Pattern(string=w787, regular expression=":ATOB:") -> (after substring=w799:string)  [unwired: 1 in, 3 out]
          n621 = Fract/Exp String To Number(string=w797) -> (number=w796:dbl)  [unwired: 3 in, 1 out]
          n622 = Fract/Exp String To Number(string=w799) -> (number=w795:dbl)  [unwired: 3 in, 1 out]
          n623 = Divide(x=w796, y=w795) -> (x/y=w786:dbl)
          n624 = local write "read buffer MercuryIPS"(w787) -> ()
          n625 = local write "MercuryIPS_Error"(w789) -> ()
        }
      }
    }
    frame #4 {
      w809 = path "C:/Users/Artem/data"  # Location of "data" folder
      # "Reserve a name for new data file:"
      n626 = call "AutoNamerDatExtraArtem.vi"("ExtraString"="", "Custom User Path"=w809) -> ("String"=w807:string, "Path"=w808:path)
      n627 = Path To String(path=w808) -> (string=w812:string)
      n628 = Concatenate Strings(w812, "\\", w807) -> (w810:string)
      n629 = String To Path(string=w810) -> (path=w805:path)
      n630 = local write "Data file:"(w805) -> ()
    }
    frame #5 {
      # "add \"formula\" string to the axis rings"
      n631 = property on="Figure_axis" class="Arr (strict)"() -> ("Value"=w815:string[])  [unwired: 2 in, 2 out]
      n632 = Build Array (concatenate)(w815, "formula") -> (w813:string[])
      n633 = property on="Figure_axis" class="Arr (strict)"("Value"=w813) -> ()  [unwired: 2 in, 2 out]
    }
    frame #6 {
      # "passes array to ring"
      # "records the fist line into the data file"
      n634 = property on="data_caption" class="Str"() -> ("Value"=w817:string)  [unwired: 2 in, 2 out]
      n635 = local read "Data file:"() -> (w818:path)
      n636 = Concatenate Strings(w817, "\r") -> (w820:string)
      n637 = Write to Text File(file (use dialog)=w818, text=w820) -> ()  [unwired: 2 in, 3 out]
      n638 = property on="Figure_axis" class="Arr (strict)"() -> ("Value"=w816:string[])  [unwired: 2 in, 2 out]
      n639 = property on="Xaxis" class="Ring (strict)"("Strings []"=w816) -> ()  [unwired: 2 in, 2 out]
      n640 = property on="Yaxis" class="Ring (strict)"("Strings []"=w816) -> ()  [unwired: 2 in, 2 out]
    }
  }
  n641 = case shown="True" w4 {
    tunnel: w3 -> [w821 w822]
    tunnel: [w821 w822] -> w2
    frame False {
    }
    frame True {
      n642 = local read "upper limit"() -> (w823:dbl)
      n643 = local write "sweep to:"(w823) -> ()
    }
  }
  n644 = while {
    tunnel: w9 -> [w850]
    shift-right: [w846] -> w5
    shift-left: w8 -> [w847]
    shift-right: [w844] -> _
    shift-left: w2 -> [w843]
    tunnel: w7 -> [w841]
    shift-right: [w824] -> _
    shift-left: w1 -> [w825]
    i -> [w827]
    stop <- w834 stop-if-true
    # "data array"
    # "this loop stops when target value is reached"
    # "error cluster to determine data flow"
    n645 = stacked-sequence {
      tunnel: w850 -> [_ _ _ w950 _]
      tunnel: [_ _ _ w949 _] -> w849
      tunnel: [_ _ w926 _ _] -> w826
      tunnel: [_ _ w925 _ _] -> w845
      tunnel: w843 -> [_ _ w919 _ _]
      tunnel: [w914 _ _ _ _] -> w842
      tunnel: w841 -> [_ _ _ w948 _]
      frame #0 {
        # "time is measured at the beginning\nand at the end of the cycle to\ncalculate delay time required to\nkeep set sweep rate"
        n646 = flat-sequence {
          tunnel: [w916] -> w914
          frame #0 {
            n647 = property on="time delay, ms" class="DigNum (strict)"() -> ("Value"=w915:dbl)  [unwired: 2 in, 2 out]
            n648 = Wait (ms)(milliseconds to wait=w915) -> ()  [unwired: 1 out]
          }
          frame #1 {
            n649 = Tick Count (ms)() -> (millisecond timer value=w916:u32)
          }
        }
      }
      frame #1 {
        w917 = dbl[] []  # Empty array for data
        # "clear data array before each measurement cycle"
        n650 = property on="data" class="Arr (strict)"("Value"=w917) -> ()  [unwired: 2 in, 2 out]
      }
      frame #2 {
        # "add next sweep value to the data array"
        n651 = local read "sweep"() -> (w922:T3)
        n652 = Equal?(x=w922, y=T7."Radio Selection 7" ("sweep")) -> (x = y?=w920:bool)
        n653 = case shown="False" w920 {
          tunnel: [w927 w944] -> w926
          tunnel: [w928 w943] -> w925
          tunnel: w919 -> [_ w941]
          tunnel: [w928 w941] -> w918
          frame True {
            # "sweeping magnetic field of Hulk"
            n654 = stacked-sequence {
              tunnel: [_ w931 _] -> w928
              tunnel: [_ _ w936] -> w927
              frame #0 {
                n655 = local read "Hulk_SMS_addr"() -> (w930:refnum<visa-resource-name>)
                n656 = VISA Clear(VISA resource name=w930) -> (error out=w929:errorcluster)  [unwired: 1 in, 1 out]
                n657 = local write "CRYogenic:("(w929) -> ()
              }
              frame #1 {
                # "acquires current output value"
                n658 = local read "Hulk_SMS_addr"() -> (w932:refnum<visa-resource-name>)
                n659 = local read "CRYogenic:("() -> (w933:errorcluster)
                n660 = call "SMS_GET_OUTPUT.vi"("CRYogenic:("=w933, "Hulk_SMS_addr"=w932) -> ("error IO"=w935:errorcluster, "read buffer"=w934:string, "Numeric"=w931:dbl)
                n661 = local write "Word from HULK!"(w934) -> ()
                n662 = local write "CRYogenic:("(w935) -> ()
              }
              frame #2 {
                # "checks, wheter ramp was finished"
                n663 = local read "Hulk_SMS_addr"() -> (w937:refnum<visa-resource-name>)
                n664 = local read "CRYogenic:("() -> (w938:errorcluster)
                n665 = call "SMS_RAMP_STATUS.vi"("CRYogenic:("=w938, "Hulk_SMS_addr"=w937) -> ("error out"=w939:errorcluster, "selection"=w936:bool, "read buffer"=w940:string)
                n666 = local write "Word from HULK!"(w940) -> ()
                n667 = local write "CRYogenic:("(w939) -> ()
              }
            }
          }
          frame False {
            # "calculate next value"
            n668 = call "CalculateNextValue.vi"("Target a 2"="sweep to:", "Channel a source value"=w941, "Ch a sweep rate units/min"="sweep rate, /min", "time between points, sec"="time/point, sec", "Source a"=Source."Voltage") -> ("Target a"=w943:dbl, "Boolean"=w944:bool)
          }
        }
        n669 = property on="data" class="Arr (strict)"() -> ("Value"=w924:dbl[])  [unwired: 2 in, 2 out]
        n670 = Build Array (concatenate)(w924, w918) -> (w923:dbl[])
        n671 = property on="data" class="Arr (strict)"("Value"=w923) -> ()  [unwired: 2 in, 2 out]
      }
      frame #3 {
        n672 = stacked-sequence "measurement sequence" {
          tunnel: w950 -> [_ _ _ _ _ _ _ _ _ _ _ _ _ _ _ _ _ _ _ _ _ _ _ _ _ _ _ _ _ _ _ _ _ _ w1481 _ _ _ _]
          tunnel: [_ _ _ _ _ _ _ _ _ _ _ _ _ _ _ _ _ _ _ _ _ _ _ _ _ _ _ _ _ _ _ _ _ _ w1481 _ _ _ _] -> w949
          tunnel: w948 -> [_ _ _ _ _ _ _ _ _ _ _ _ _ _ _ _ _ _ _ _ _ _ _ _ _ _ _ _ _ _ _ _ _ _ w1482 _ _ _ _]
          frame #0 {
            # "check if in-phase\nsignal on lock-in 1 \nis to be measured"
            n673 = property on="data" class="Arr (strict)"() -> ("Value"=w952:dbl[])  [unwired: 2 in, 2 out]
            n674 = local read "SR830 1 ip"() -> (w951:bool)
            n675 = case shown="True" w951 {
              tunnel: w952 -> [w954 w963]
              tunnel: [w954 w962] -> w953
              frame False {
                # "we are not measuring in phase signal on lock-in 1 (SR830_1_ip)"
              }
              frame True {
                # "we are  measuring lock-in 1, in phase (SR830_1_ip)"
                n676 = local read "SR830 1 addr"() -> (w956:u8)
                n677 = Number To Decimal String(number=w956) -> (decimal integer string=w955:string)  [unwired: 1 in]
                n678 = GPIB Write(0:w955, 1:"OUTP?1") -> (6:w961:errorcluster)  [unwired: 3 in, 1 out]
                n679 = GPIB Read(0:w955, 1:3200, 3:w961) -> (5:w959:string)  [unwired: 2 in, 2 out]
                n680 = Fract/Exp String To Number(string=w959) -> (number=w958:dbl)  [unwired: 3 in, 1 out]
                n681 = Build Array (concatenate)(w963, w958) -> (w962:dbl[])
              }
            }
            n682 = property on="data" class="Arr (strict)"("Value"=w953) -> ()  [unwired: 2 in, 2 out]
          }
          frame #1 {
            # "check if out-of-phase\nsignal on lock-in 1 \nis to be measured"
            n683 = property on="data" class="Arr (strict)"() -> ("Value"=w965:dbl[])  [unwired: 2 in, 2 out]
            n684 = local read "SR830 1 oop"() -> (w964:bool)
            n685 = case shown="True" w964 {
              tunnel: w965 -> [w967 w976]
              tunnel: [w967 w975] -> w966
              frame False {
                # "we are not measuring out of phase signal on lock-in 1 (SR830_1_oop)"
              }
              frame True {
                # "we are  measuring lock-in 1, out of phase (SR830_1_oop)"
                n686 = local read "SR830 1 addr"() -> (w969:u8)
                n687 = Number To Decimal String(number=w969) -> (decimal integer string=w968:string)  [unwired: 1 in]
                n688 = GPIB Write(0:w968, 1:"OUTP?2") -> (6:w974:errorcluster)  [unwired: 3 in, 1 out]
                n689 = GPIB Read(0:w968, 1:3200, 3:w974) -> (5:w972:string)  [unwired: 2 in, 2 out]
                n690 = Fract/Exp String To Number(string=w972) -> (number=w971:dbl)  [unwired: 3 in, 1 out]
                n691 = Build Array (concatenate)(w976, w971) -> (w975:dbl[])
              }
            }
            n692 = property on="data" class="Arr (strict)"("Value"=w966) -> ()  [unwired: 2 in, 2 out]
          }
          frame #2 {
            # "check if in-phase\nsignal on lock-in 2 \nis to be measured"
            n693 = property on="data" class="Arr (strict)"() -> ("Value"=w978:dbl[])  [unwired: 2 in, 2 out]
            n694 = local read "SR830 2 ip"() -> (w977:bool)
            n695 = case shown="False" w977 {
              tunnel: w978 -> [w980 w989]
              tunnel: [w980 w988] -> w979
              frame False {
                # "we are not measuring in phase signal on lock-in 2 (SR830_2_ip)"
              }
              frame True {
                # "we are  measuring lock-in 2, in phase (SR830_2_ip)"
                n696 = local read "SR830 2 addr"() -> (w982:u8)
                n697 = Number To Decimal String(number=w982) -> (decimal integer string=w981:string)  [unwired: 1 in]
                n698 = GPIB Write(0:w981, 1:"OUTP?1") -> (6:w987:errorcluster)  [unwired: 3 in, 1 out]
                n699 = GPIB Read(0:w981, 1:3200, 3:w987) -> (5:w985:string)  [unwired: 2 in, 2 out]
                n700 = Fract/Exp String To Number(string=w985) -> (number=w984:dbl)  [unwired: 3 in, 1 out]
                n701 = Build Array (concatenate)(w989, w984) -> (w988:dbl[])
              }
            }
            n702 = property on="data" class="Arr (strict)"("Value"=w979) -> ()  [unwired: 2 in, 2 out]
          }
          frame #3 {
            # "check if out-of-phase\nsignal on lock-in 2 \nis to be measured"
            n703 = property on="data" class="Arr (strict)"() -> ("Value"=w991:dbl[])  [unwired: 2 in, 2 out]
            n704 = local read "SR830 2 oop"() -> (w990:bool)
            n705 = case shown="True" w990 {
              tunnel: w991 -> [w993 w1002]
              tunnel: [w993 w1001] -> w992
              frame False {
                # "we are not measuring out of phase signal on lock-in 2 (SR830_2_oop)"
              }
              frame True {
                # "we are  measuring lock-in 2, out of phase (SR830_2_oop)"
                n706 = local read "SR830 2 addr"() -> (w995:u8)
                n707 = Number To Decimal String(number=w995) -> (decimal integer string=w994:string)  [unwired: 1 in]
                n708 = GPIB Write(0:w994, 1:"OUTP?2") -> (6:w1000:errorcluster)  [unwired: 3 in, 1 out]
                n709 = GPIB Read(0:w994, 1:3200, 3:w1000) -> (5:w998:string)  [unwired: 2 in, 2 out]
                n710 = Fract/Exp String To Number(string=w998) -> (number=w997:dbl)  [unwired: 3 in, 1 out]
                n711 = Build Array (concatenate)(w1002, w997) -> (w1001:dbl[])
              }
            }
            n712 = property on="data" class="Arr (strict)"("Value"=w992) -> ()  [unwired: 2 in, 2 out]
          }
          frame #4 {
            # "check if in-phase\nsignal on lock-in 3 \nis to be measured"
            n713 = property on="data" class="Arr (strict)"() -> ("Value"=w1004:dbl[])  [unwired: 2 in, 2 out]
            n714 = local read "SR830 3 ip"() -> (w1003:bool)
            n715 = case shown="True" w1003 {
              tunnel: w1004 -> [w1006 w1015]
              tunnel: [w1006 w1014] -> w1005
              frame False {
                # "we are not measuring in phase signal on lock-in 3 (SR830_3_ip)"
              }
              frame True {
                # "we are  measuring lock-in 3, in phase (SR830_3_ip)"
                n716 = local read "SR830 3 addr"() -> (w1008:u8)
                n717 = Number To Decimal String(number=w1008) -> (decimal integer string=w1007:string)  [unwired: 1 in]
                n718 = GPIB Write(0:w1007, 1:"OUTP?1") -> (6:w1013:errorcluster)  [unwired: 3 in, 1 out]
                n719 = GPIB Read(0:w1007, 1:3200, 3:w1013) -> (5:w1011:string)  [unwired: 2 in, 2 out]
                n720 = Fract/Exp String To Number(string=w1011) -> (number=w1010:dbl)  [unwired: 3 in, 1 out]
                n721 = Build Array (concatenate)(w1015, w1010) -> (w1014:dbl[])
              }
            }
            n722 = property on="data" class="Arr (strict)"("Value"=w1005) -> ()  [unwired: 2 in, 2 out]
          }
          frame #5 {
            # "check if out-of-phase\nsignal on lock-in 3 \nis to be measured"
            n723 = property on="data" class="Arr (strict)"() -> ("Value"=w1017:dbl[])  [unwired: 2 in, 2 out]
            n724 = local read "SR830 3 oop"() -> (w1016:bool)
            n725 = case shown="True" w1016 {
              tunnel: w1017 -> [w1019 w1028]
              tunnel: [w1019 w1027] -> w1018
              frame False {
                # "we are not measuring out of phase signal on lock-in 3 (SR830_3_oop)"
              }
              frame True {
                # "we are  measuring lock-in 3, out of phase (SR830_3_oop)"
                n726 = local read "SR830 3 addr"() -> (w1021:u8)
                n727 = Number To Decimal String(number=w1021) -> (decimal integer string=w1020:string)  [unwired: 1 in]
                n728 = GPIB Write(0:w1020, 1:"OUTP?2") -> (6:w1026:errorcluster)  [unwired: 3 in, 1 out]
                n729 = GPIB Read(0:w1020, 1:3200, 3:w1026) -> (5:w1024:string)  [unwired: 2 in, 2 out]
                n730 = Fract/Exp String To Number(string=w1024) -> (number=w1023:dbl)  [unwired: 3 in, 1 out]
                n731 = Build Array (concatenate)(w1028, w1023) -> (w1027:dbl[])
              }
            }
            n732 = property on="data" class="Arr (strict)"("Value"=w1018) -> ()  [unwired: 2 in, 2 out]
          }
          frame #6 {
            # "check if in-phase\nsignal on lock-in 4 \nis to be measured"
            n733 = property on="data" class="Arr (strict)"() -> ("Value"=w1030:dbl[])  [unwired: 2 in, 2 out]
            n734 = local read "SR830 4 ip"() -> (w1029:bool)
            n735 = case shown="True" w1029 {
              tunnel: w1030 -> [w1032 w1041]
              tunnel: [w1032 w1040] -> w1031
              frame False {
                # "we are not measuring in phase signal on lock-in 4 (SR830_4_ip)"
              }
              frame True {
                # "we are  measuring lock-in 4, in phase (SR830_4_ip)"
                n736 = local read "SR830 4 addr"() -> (w1034:u8)
                n737 = Number To Decimal String(number=w1034) -> (decimal integer string=w1033:string)  [unwired: 1 in]
                n738 = GPIB Write(0:w1033, 1:"OUTP?1") -> (6:w1039:errorcluster)  [unwired: 3 in, 1 out]
                n739 = GPIB Read(0:w1033, 1:3200, 3:w1039) -> (5:w1037:string)  [unwired: 2 in, 2 out]
                n740 = Fract/Exp String To Number(string=w1037) -> (number=w1036:dbl)  [unwired: 3 in, 1 out]
                n741 = Build Array (concatenate)(w1041, w1036) -> (w1040:dbl[])
              }
            }
            n742 = property on="data" class="Arr (strict)"("Value"=w1031) -> ()  [unwired: 2 in, 2 out]
          }
          frame #7 {
            # "check if out-of-phase\nsignal on lock-in 4 \nis to be measured"
            n743 = property on="data" class="Arr (strict)"() -> ("Value"=w1043:dbl[])  [unwired: 2 in, 2 out]
            n744 = local read "SR830 4 oop"() -> (w1042:bool)
            n745 = case shown="True" w1042 {
              tunnel: w1043 -> [w1045 w1054]
              tunnel: [w1045 w1053] -> w1044
              frame False {
                # "we are not measuring out of phase signal on lock-in 4 (SR830_4_oop)"
              }
              frame True {
                # "we are  measuring lock-in 4, out of phase (SR830_4_oop)"
                n746 = local read "SR830 4 addr"() -> (w1047:u8)
                n747 = Number To Decimal String(number=w1047) -> (decimal integer string=w1046:string)  [unwired: 1 in]
                n748 = GPIB Write(0:w1046, 1:"OUTP?2") -> (6:w1052:errorcluster)  [unwired: 3 in, 1 out]
                n749 = GPIB Read(0:w1046, 1:3200, 3:w1052) -> (5:w1050:string)  [unwired: 2 in, 2 out]
                n750 = Fract/Exp String To Number(string=w1050) -> (number=w1049:dbl)  [unwired: 3 in, 1 out]
                n751 = Build Array (concatenate)(w1054, w1049) -> (w1053:dbl[])
              }
            }
            n752 = property on="data" class="Arr (strict)"("Value"=w1044) -> ()  [unwired: 2 in, 2 out]
          }
          frame #8 {
            # "check if in-phase\nsignal on lock-in 5 \nis to be measured"
            n753 = property on="data" class="Arr (strict)"() -> ("Value"=w1056:dbl[])  [unwired: 2 in, 2 out]
            n754 = local read "SR830 5 ip"() -> (w1055:bool)
            n755 = case shown="True" w1055 {
              tunnel: w1056 -> [w1058 w1067]
              tunnel: [w1058 w1066] -> w1057
              frame False {
                # "we are not measuring in phase signal on lock-in 5 (SR830_5_ip)"
              }
              frame True {
                # "we are  measuring lock-in 5, in phase (SR830_5_ip)"
                n756 = local read "SR830 5 addr"() -> (w1060:u8)
                n757 = Number To Decimal String(number=w1060) -> (decimal integer string=w1059:string)  [unwired: 1 in]
                n758 = GPIB Write(0:w1059, 1:"OUTP?1") -> (6:w1065:errorcluster)  [unwired: 3 in, 1 out]
                n759 = GPIB Read(0:w1059, 1:3200, 3:w1065) -> (5:w1063:string)  [unwired: 2 in, 2 out]
                n760 = Fract/Exp String To Number(string=w1063) -> (number=w1062:dbl)  [unwired: 3 in, 1 out]
                n761 = Build Array (concatenate)(w1067, w1062) -> (w1066:dbl[])
              }
            }
            n762 = property on="data" class="Arr (strict)"("Value"=w1057) -> ()  [unwired: 2 in, 2 out]
          }
          frame #9 {
            # "check if out-of-phase\nsignal on lock-in 5 \nis to be measured"
            n763 = property on="data" class="Arr (strict)"() -> ("Value"=w1069:dbl[])  [unwired: 2 in, 2 out]
            n764 = local read "SR830 5 oop"() -> (w1068:bool)
            n765 = case shown="True" w1068 {
              tunnel: w1069 -> [w1071 w1080]
              tunnel: [w1071 w1079] -> w1070
              frame False {
                # "we are not measuring out of phase signal on lock-in 5 (SR830_5_oop)"
              }
              frame True {
                # "we are  measuring lock-in 5, out of phase (SR830_5_oop)"
                n766 = local read "SR830 5 addr"() -> (w1073:u8)
                n767 = Number To Decimal String(number=w1073) -> (decimal integer string=w1072:string)  [unwired: 1 in]
                n768 = GPIB Write(0:w1072, 1:"OUTP?2") -> (6:w1078:errorcluster)  [unwired: 3 in, 1 out]
                n769 = GPIB Read(0:w1072, 1:3200, 3:w1078) -> (5:w1076:string)  [unwired: 2 in, 2 out]
                n770 = Fract/Exp String To Number(string=w1076) -> (number=w1075:dbl)  [unwired: 3 in, 1 out]
                n771 = Build Array (concatenate)(w1080, w1075) -> (w1079:dbl[])
              }
            }
            n772 = property on="data" class="Arr (strict)"("Value"=w1070) -> ()  [unwired: 2 in, 2 out]
          }
          frame #10 {
            # "check if voltage \non 2400 SouceMeter 1\nis to be measured"
            n773 = property on="data" class="Arr (strict)"() -> ("Value"=w1082:dbl[])  [unwired: 2 in, 2 out]
            n774 = local read "2400 1 meas v"() -> (w1081:bool)
            n775 = case shown="True" w1081 {
              tunnel: w1082 -> [w1084 w1095]
              tunnel: [w1084 w1094] -> w1083
              frame False {
                # "we are not measuring 2400 1, voltage (2400_1_v)"
              }
              frame True {
                # "we are  measuring 2400 1, voltage (2400_1_v)"
                n776 = local read "2400 1 addr"() -> (w1089:u8)
                n777 = Number To Decimal String(number=w1089) -> (decimal integer string=w1088:string)  [unwired: 1 in]
                n778 = GPIB Write(0:w1088, 1:":READ?") -> (6:w1093:errorcluster)  [unwired: 3 in, 1 out]
                n779 = GPIB Read(0:w1088, 1:3200, 3:w1093) -> (5:w1086:string)  [unwired: 2 in, 2 out]
                n780 = String Subset(string=w1086, length (rest)=13) -> (substring=w1085:string)  [unwired: 1 in]
                n781 = Fract/Exp String To Number(string=w1085) -> (number=w1091:dbl)  [unwired: 3 in, 1 out]
                n782 = Build Array (concatenate)(w1095, w1091) -> (w1094:dbl[])
              }
            }
            n783 = property on="data" class="Arr (strict)"("Value"=w1083) -> ()  [unwired: 2 in, 2 out]
          }
          frame #11 {
            # "check if current \non 2400 SouceMeter 1\nis to be measured"
            n784 = property on="data" class="Arr (strict)"() -> ("Value"=w1097:dbl[])  [unwired: 2 in, 2 out]
            n785 = local read "2400 1 meas i"() -> (w1096:bool)
            n786 = case shown="True" w1096 {
              tunnel: w1097 -> [w1099 w1111]
              tunnel: [w1099 w1110] -> w1098
              frame False {
                # "we are not measuring 2400 1, current (2400_1_i)"
              }
              frame True {
                # "we are  measuring 2400 1, current (2400_1_i)"
                n787 = local read "2400 1 addr"() -> (w1105:u8)
                n788 = Number To Decimal String(number=w1105) -> (decimal integer string=w1104:string)  [unwired: 1 in]
                n789 = GPIB Write(0:w1104, 1:":READ?") -> (6:w1109:errorcluster)  [unwired: 3 in, 1 out]
                n790 = GPIB Read(0:w1104, 1:3200, 3:w1109) -> (5:w1102:string)  [unwired: 2 in, 2 out]
                n791 = String Subset(string=w1102, offset (0)=14, length (rest)=13) -> (substring=w1101:string)
                n792 = Fract/Exp String To Number(string=w1101) -> (number=w1107:dbl)  [unwired: 3 in, 1 out]
                n793 = Build Array (concatenate)(w1111, w1107) -> (w1110:dbl[])
              }
            }
            n794 = property on="data" class="Arr (strict)"("Value"=w1098) -> ()  [unwired: 2 in, 2 out]
          }
          frame #12 {
            # "check if voltage \non 2400 SouceMeter 2\nis to be measured"
            n795 = property on="data" class="Arr (strict)"() -> ("Value"=w1113:dbl[])  [unwired: 2 in, 2 out]
            n796 = local read "2400 2 meas v"() -> (w1112:bool)
            n797 = case shown="True" w1112 {
              tunnel: w1113 -> [w1115 w1126]
              tunnel: [w1115 w1125] -> w1114
              frame False {
                # "we are not measuring 2400 2, voltage (2400_2_v)"
              }
              frame True {
                # "we are  measuring 2400 2, voltage (2400_2_v)"
                n798 = local read "2400 2 addr"() -> (w1120:u8)
                n799 = Number To Decimal String(number=w1120) -> (decimal integer string=w1119:string)  [unwired: 1 in]
                n800 = GPIB Write(0:w1119, 1:":READ?") -> (6:w1124:errorcluster)  [unwired: 3 in, 1 out]
                n801 = GPIB Read(0:w1119, 1:3200, 3:w1124) -> (5:w1117:string)  [unwired: 2 in, 2 out]
                n802 = String Subset(string=w1117, length (rest)=13) -> (substring=w1116:string)  [unwired: 1 in]
                n803 = Fract/Exp String To Number(string=w1116) -> (number=w1122:dbl)  [unwired: 3 in, 1 out]
                n804 = Build Array (concatenate)(w1126, w1122) -> (w1125:dbl[])
              }
            }
            n805 = property on="data" class="Arr (strict)"("Value"=w1114) -> ()  [unwired: 2 in, 2 out]
          }
          frame #13 {
            # "check if current \non 2400 SouceMeter 2\nis to be measured"
            n806 = property on="data" class="Arr (strict)"() -> ("Value"=w1128:dbl[])  [unwired: 2 in, 2 out]
            n807 = local read "2400 2 meas i"() -> (w1127:bool)
            n808 = case shown="True" w1127 {
              tunnel: w1128 -> [w1130 w1142]
              tunnel: [w1130 w1141] -> w1129
              frame False {
                # "we are not measuring 2400 2, current (2400_2_i)"
              }
              frame True {
                # "we are  measuring 2400 2, current (2400_2_i)"
                n809 = local read "2400 2 addr"() -> (w1136:u8)
                n810 = Number To Decimal String(number=w1136) -> (decimal integer string=w1135:string)  [unwired: 1 in]
                n811 = GPIB Write(0:w1135, 1:":READ?") -> (6:w1140:errorcluster)  [unwired: 3 in, 1 out]
                n812 = GPIB Read(0:w1135, 1:3200, 3:w1140) -> (5:w1133:string)  [unwired: 2 in, 2 out]
                n813 = String Subset(string=w1133, offset (0)=14, length (rest)=13) -> (substring=w1132:string)
                n814 = Fract/Exp String To Number(string=w1132) -> (number=w1138:dbl)  [unwired: 3 in, 1 out]
                n815 = Build Array (concatenate)(w1142, w1138) -> (w1141:dbl[])
              }
            }
            n816 = property on="data" class="Arr (strict)"("Value"=w1129) -> ()  [unwired: 2 in, 2 out]
          }
          frame #14 {
            # "check if voltage \non 2400 SouceMeter 3\nis to be measured"
            n817 = property on="data" class="Arr (strict)"() -> ("Value"=w1144:dbl[])  [unwired: 2 in, 2 out]
            n818 = local read "2400 3 meas v"() -> (w1143:bool)
            n819 = case shown="True" w1143 {
              tunnel: w1144 -> [w1146 w1157]
              tunnel: [w1146 w1156] -> w1145
              frame False {
                # "we are not measuring 2400 3, voltage (2400_3_v)"
              }
              frame True {
                # "we are  measuring 2400 3, voltage (2400_3_v)"
                n820 = local read "2400 3 addr"() -> (w1151:u8)
                n821 = Number To Decimal String(number=w1151) -> (decimal integer string=w1150:string)  [unwired: 1 in]
                n822 = GPIB Write(0:w1150, 1:":READ?") -> (6:w1155:errorcluster)  [unwired: 3 in, 1 out]
                n823 = GPIB Read(0:w1150, 1:3200, 3:w1155) -> (5:w1148:string)  [unwired: 2 in, 2 out]
                n824 = String Subset(string=w1148, length (rest)=13) -> (substring=w1147:string)  [unwired: 1 in]
                n825 = Fract/Exp String To Number(string=w1147) -> (number=w1153:dbl)  [unwired: 3 in, 1 out]
                n826 = Build Array (concatenate)(w1157, w1153) -> (w1156:dbl[])
              }
            }
            n827 = property on="data" class="Arr (strict)"("Value"=w1145) -> ()  [unwired: 2 in, 2 out]
          }
          frame #15 {
            # "check if current \non 2400 SouceMeter 3\nis to be measured"
            n828 = property on="data" class="Arr (strict)"() -> ("Value"=w1159:dbl[])  [unwired: 2 in, 2 out]
            n829 = local read "2400 3 meas i"() -> (w1158:bool)
            n830 = case shown="True" w1158 {
              tunnel: w1159 -> [w1161 w1173]
              tunnel: [w1161 w1172] -> w1160
              frame False {
                # "we are not measuring 2400 3, current (2400_3_i)"
              }
              frame True {
                # "we are  measuring 2400 3, current (2400_3_i)"
                n831 = local read "2400 3 addr"() -> (w1167:u8)
                n832 = Number To Decimal String(number=w1167) -> (decimal integer string=w1166:string)  [unwired: 1 in]
                n833 = GPIB Write(0:w1166, 1:":READ?") -> (6:w1171:errorcluster)  [unwired: 3 in, 1 out]
                n834 = GPIB Read(0:w1166, 1:3200, 3:w1171) -> (5:w1164:string)  [unwired: 2 in, 2 out]
                n835 = String Subset(string=w1164, offset (0)=14, length (rest)=13) -> (substring=w1163:string)
                n836 = Fract/Exp String To Number(string=w1163) -> (number=w1169:dbl)  [unwired: 3 in, 1 out]
                n837 = Build Array (concatenate)(w1173, w1169) -> (w1172:dbl[])
              }
            }
            n838 = property on="data" class="Arr (strict)"("Value"=w1160) -> ()  [unwired: 2 in, 2 out]
          }
          frame #16 {
            # "check if 1st channel \non Keithley 2182A 1\nis to be measured"
            n839 = property on="data" class="Arr (strict)"() -> ("Value"=w1175:dbl[])  [unwired: 2 in, 2 out]
            n840 = local read "2182A 1 ch1"() -> (w1174:bool)
            n841 = case shown="True" w1174 {
              tunnel: w1175 -> [w1177 w1186]
              tunnel: [w1177 w1185] -> w1176
              frame False {
                # "we are not measuring 2182A 1 channel 1 (2182A_1_ch1)"
              }
              frame True {
                # "we are  measuring 2182A 1 channel 1 (2182A_1_ch1)"
                n842 = local read "2182A 1 addr"() -> (w1180:u8)
                n843 = Number To Decimal String(number=w1180) -> (decimal integer string=w1179:string)  [unwired: 1 in]
                n844 = GPIB Write(0:w1179, 1:":SENSe:DATA:FRES?") -> (6:w1184:errorcluster)  [unwired: 3 in, 1 out]
                n845 = GPIB Read(0:w1179, 1:200, 3:w1184) -> (5:w1178:string)  [unwired: 2 in, 2 out]
                n846 = Fract/Exp String To Number(string=w1178) -> (number=w1182:dbl)  [unwired: 3 in, 1 out]
                n847 = Build Array (concatenate)(w1186, w1182) -> (w1185:dbl[])
              }
            }
            n848 = property on="data" class="Arr (strict)"("Value"=w1176) -> ()  [unwired: 2 in, 2 out]
          }
          frame #17 {
            # "check if 2nd channel \non Keithley 2182A 1\nis to be measured"
            n849 = property on="data" class="Arr (strict)"() -> ("Value"=w1188:dbl[])  [unwired: 2 in, 2 out]
            n850 = local read "2182A 1 ch2"() -> (w1187:bool)
            n851 = case shown="True" w1187 {
              tunnel: w1188 -> [w1190 w1203]
              tunnel: [w1190 w1202] -> w1189
              frame False {
                # "we are not measuring 2182A 1 channel 2 (2182A_1_ch2)"
              }
              frame True {
                # "switching to channel 2 and then\nback to channel 1"
                # "we are  measuring 2182A 1 channel 2 (2182A_1_ch2)"
                n852 = local read "2182A 1 addr"() -> (w1197:u8)
                n853 = Number To Decimal String(number=w1197) -> (decimal integer string=w1192:string)  [unwired: 1 in]
                n854 = GPIB Write(0:w1192, 1:":SENSe:CHAN 2") -> (6:w1194:errorcluster)  [unwired: 3 in, 1 out]
                n855 = GPIB Write(0:w1192, 1:":SENSe:DATA:FRES?", 3:w1194) -> (6:w1201:errorcluster)  [unwired: 2 in, 1 out]
                n856 = GPIB Read(0:w1192, 1:200, 3:w1201) -> (5:w1196:string, 7:w1193:errorcluster)  [unwired: 2 in, 1 out]
                n857 = GPIB Write(0:w1192, 1:":SENSe:CHAN 1", 3:w1193) -> ()  [unwired: 2 in, 2 out]
                n858 = Fract/Exp String To Number(string=w1196) -> (number=w1199:dbl)  [unwired: 3 in, 1 out]
                n859 = Build Array (concatenate)(w1203, w1199) -> (w1202:dbl[])
              }
            }
            n860 = property on="data" class="Arr (strict)"("Value"=w1189) -> ()  [unwired: 2 in, 2 out]
          }
          frame #18 {
            # "check if 1st channel \non Keithley 2182A 2\nis to be measured"
            n861 = property on="data" class="Arr (strict)"() -> ("Value"=w1205:dbl[])  [unwired: 2 in, 2 out]
            n862 = local read "2182A 2 ch1"() -> (w1204:bool)
            n863 = case shown="True" w1204 {
              tunnel: w1205 -> [w1207 w1216]
              tunnel: [w1207 w1215] -> w1206
              frame False {
                # "we are not measuring 2182A 2 channel 1 (2182A_2_ch1)"
              }
              frame True {
                # "we are  measuring 2182A 2 channel 1 (2182A_2_ch1)"
                n864 = local read "2182A 2 addr"() -> (w1210:u8)
                n865 = Number To Decimal String(number=w1210) -> (decimal integer string=w1209:string)  [unwired: 1 in]
                n866 = GPIB Write(0:w1209, 1:":SENSe:DATA:FRES?") -> (6:w1214:errorcluster)  [unwired: 3 in, 1 out]
                n867 = GPIB Read(0:w1209, 1:200, 3:w1214) -> (5:w1208:string)  [unwired: 2 in, 2 out]
                n868 = Fract/Exp String To Number(string=w1208) -> (number=w1212:dbl)  [unwired: 3 in, 1 out]
                n869 = Build Array (concatenate)(w1216, w1212) -> (w1215:dbl[])
              }
            }
            n870 = property on="data" class="Arr (strict)"("Value"=w1206) -> ()  [unwired: 2 in, 2 out]
          }
          frame #19 {
            # "check if 2nd channel \non Keithley 2182A 2\nis to be measured"
            n871 = property on="data" class="Arr (strict)"() -> ("Value"=w1218:dbl[])  [unwired: 2 in, 2 out]
            n872 = local read "2182A 2 ch2"() -> (w1217:bool)
            n873 = case shown="True" w1217 {
              tunnel: w1218 -> [w1220 w1233]
              tunnel: [w1220 w1232] -> w1219
              frame False {
                # "we are not measuring 2182A 2 channel 2 (2182A_2_ch2)"
              }
              frame True {
                # "switching to channel 2 and then\nback to channel 1"
                # "we are  measuring 2182A 2 channel 2 (2182A_2_ch2)"
                n874 = local read "2182A 2 addr"() -> (w1227:u8)
                n875 = Number To Decimal String(number=w1227) -> (decimal integer string=w1222:string)  [unwired: 1 in]
                n876 = GPIB Write(0:w1222, 1:":SENSe:CHAN 2") -> (6:w1224:errorcluster)  [unwired: 3 in, 1 out]
                n877 = GPIB Write(0:w1222, 1:":SENSe:DATA:FRES?", 3:w1224) -> (6:w1231:errorcluster)  [unwired: 2 in, 1 out]
                n878 = GPIB Read(0:w1222, 1:200, 3:w1231) -> (5:w1226:string, 7:w1223:errorcluster)  [unwired: 2 in, 1 out]
                n879 = GPIB Write(0:w1222, 1:":SENSe:CHAN 1", 3:w1223) -> ()  [unwired: 2 in, 2 out]
                n880 = Fract/Exp String To Number(string=w1226) -> (number=w1229:dbl)  [unwired: 3 in, 1 out]
                n881 = Build Array (concatenate)(w1233, w1229) -> (w1232:dbl[])
              }
            }
            n882 = property on="data" class="Arr (strict)"("Value"=w1219) -> ()  [unwired: 2 in, 2 out]
          }
          frame #20 {
            # "check if 1st channel \non Keithley 2182A 3\nis to be measured"
            n883 = property on="data" class="Arr (strict)"() -> ("Value"=w1235:dbl[])  [unwired: 2 in, 2 out]
            n884 = local read "2182A 3 ch1"() -> (w1234:bool)
            n885 = case shown="True" w1234 {
              tunnel: w1235 -> [w1237 w1246]
              tunnel: [w1237 w1245] -> w1236
              frame False {
                # "we are not measuring 2182A 3 channel 1 (2182A_3_ch1)"
              }
              frame True {
                # "we are  measuring 2182A 3 channel 1 (2182A_3_ch1)"
                n886 = local read "2182A 3 addr"() -> (w1240:u8)
                n887 = Number To Decimal String(number=w1240) -> (decimal integer string=w1239:string)  [unwired: 1 in]
                n888 = GPIB Write(0:w1239, 1:":SENSe:DATA:FRES?") -> (6:w1244:errorcluster)  [unwired: 3 in, 1 out]
                n889 = GPIB Read(0:w1239, 1:200, 3:w1244) -> (5:w1238:string)  [unwired: 2 in, 2 out]
                n890 = Fract/Exp String To Number(string=w1238) -> (number=w1242:dbl)  [unwired: 3 in, 1 out]
                n891 = Build Array (concatenate)(w1246, w1242) -> (w1245:dbl[])
              }
            }
            n892 = property on="data" class="Arr (strict)"("Value"=w1236) -> ()  [unwired: 2 in, 2 out]
          }
          frame #21 {
            # "check if 2nd channel \non Keithley 2182A 3\nis to be measured"
            n893 = property on="data" class="Arr (strict)"() -> ("Value"=w1248:dbl[])  [unwired: 2 in, 2 out]
            n894 = local read "2182A 3 ch2"() -> (w1247:bool)
            n895 = case shown="True" w1247 {
              tunnel: w1248 -> [w1250 w1263]
              tunnel: [w1250 w1262] -> w1249
              frame False {
                # "we are not measuring 2182A 3 channel 2 (2182A_3_ch2)"
              }
              frame True {
                # "switching to channel 2 and then\nback to channel 1"
                # "we are  measuring 2182A 3 channel 2 (2182A_3_ch2)"
                n896 = local read "2182A 3 addr"() -> (w1257:u8)
                n897 = Number To Decimal String(number=w1257) -> (decimal integer string=w1252:string)  [unwired: 1 in]
                n898 = GPIB Write(0:w1252, 1:":SENSe:CHAN 2") -> (6:w1254:errorcluster)  [unwired: 3 in, 1 out]
                n899 = GPIB Write(0:w1252, 1:":SENSe:DATA:FRES?", 3:w1254) -> (6:w1261:errorcluster)  [unwired: 2 in, 1 out]
                n900 = GPIB Read(0:w1252, 1:200, 3:w1261) -> (5:w1256:string, 7:w1253:errorcluster)  [unwired: 2 in, 1 out]
                n901 = GPIB Write(0:w1252, 1:":SENSe:CHAN 1", 3:w1253) -> ()  [unwired: 2 in, 2 out]
                n902 = Fract/Exp String To Number(string=w1256) -> (number=w1259:dbl)  [unwired: 3 in, 1 out]
                n903 = Build Array (concatenate)(w1263, w1259) -> (w1262:dbl[])
              }
            }
            n904 = property on="data" class="Arr (strict)"("Value"=w1249) -> ()  [unwired: 2 in, 2 out]
          }
          frame #22 {
            # "check if 1st channel \non Keithley 2182A 4\nis to be measured"
            n905 = property on="data" class="Arr (strict)"() -> ("Value"=w1265:dbl[])  [unwired: 2 in, 2 out]
            n906 = local read "2182A 4 ch1"() -> (w1264:bool)
            n907 = case shown="True" w1264 {
              tunnel: w1265 -> [w1267 w1276]
              tunnel: [w1267 w1275] -> w1266
              frame False {
                # "we are not measuring 2182A 4 channel 1 (2182A_4_ch1)"
              }
              frame True {
                # "we are  measuring 2182A 4 channel 1 (2182A_4_ch1)"
                n908 = local read "2182A 4 addr"() -> (w1270:u8)
                n909 = Number To Decimal String(number=w1270) -> (decimal integer string=w1269:string)  [unwired: 1 in]
                n910 = GPIB Write(0:w1269, 1:":SENSe:DATA:FRES?") -> (6:w1274:errorcluster)  [unwired: 3 in, 1 out]
                n911 = GPIB Read(0:w1269, 1:200, 3:w1274) -> (5:w1268:string)  [unwired: 2 in, 2 out]
                n912 = Fract/Exp String To Number(string=w1268) -> (number=w1272:dbl)  [unwired: 3 in, 1 out]
                n913 = Build Array (concatenate)(w1276, w1272) -> (w1275:dbl[])
              }
            }
            n914 = property on="data" class="Arr (strict)"("Value"=w1266) -> ()  [unwired: 2 in, 2 out]
          }
          frame #23 {
            # "check if 2nd channel \non Keithley 2182A 4\nis to be measured"
            n915 = property on="data" class="Arr (strict)"() -> ("Value"=w1278:dbl[])  [unwired: 2 in, 2 out]
            n916 = local read "2182A 4 ch2"() -> (w1277:bool)
            n917 = case shown="False" w1277 {
              tunnel: w1278 -> [w1280 w1293]
              tunnel: [w1280 w1292] -> w1279
              frame False {
                # "we are not measuring 2182A 4 channel 2 (2182A_4_ch2)"
              }
              frame True {
                # "switching to channel 2 and then\nback to channel 1"
                # "we are  measuring 2182A 4 channel 2 (2182A_4_ch2)"
                n918 = local read "2182A 4 addr"() -> (w1287:u8)
                n919 = Number To Decimal String(number=w1287) -> (decimal integer string=w1282:string)  [unwired: 1 in]
                n920 = GPIB Write(0:w1282, 1:":SENSe:CHAN 2") -> (6:w1284:errorcluster)  [unwired: 3 in, 1 out]
                n921 = GPIB Write(0:w1282, 1:":SENSe:DATA:FRES?", 3:w1284) -> (6:w1291:errorcluster)  [unwired: 2 in, 1 out]
                n922 = GPIB Read(0:w1282, 1:200, 3:w1291) -> (5:w1286:string, 7:w1283:errorcluster)  [unwired: 2 in, 1 out]
                n923 = GPIB Write(0:w1282, 1:":SENSe:CHAN 1", 3:w1283) -> ()  [unwired: 2 in, 2 out]
                n924 = Fract/Exp String To Number(string=w1286) -> (number=w1289:dbl)  [unwired: 3 in, 1 out]
                n925 = Build Array (concatenate)(w1293, w1289) -> (w1292:dbl[])
              }
            }
            n926 = property on="data" class="Arr (strict)"("Value"=w1279) -> ()  [unwired: 2 in, 2 out]
          }
          frame #24 {
            # "check if voltage on\nKeithley 2636A smua\nis to be measured"
            n927 = local read "2636A smua meas v"() -> (w1294:bool)
            n928 = property on="data" class="Arr (strict)"() -> ("Value"=w1295:dbl[])  [unwired: 2 in, 2 out]
            n929 = case shown="True" w1294 {
              tunnel: w1295 -> [w1297 w1303]
              tunnel: [w1297 w1302] -> w1296
              frame False {
                # "we are not measuring voltage on 2636A smua (2636A_smua_v)"
              }
              frame True {
                # "we are  measuring voltage on 2636A smua (2636A_smua_v)"
                n930 = local read "2336A addr"() -> (w1298:refnum<visa-resource-name>)
                n931 = call "SinglePointMeasurement.vi"("Measure"=Measure."Voltage", "Channel"=Channel."a", "VISA resource name 2"=w1298) -> ("Measuremet"=w1300:dbl)  [unwired: 3 in, 4 out]
                n932 = Build Array (concatenate)(w1303, w1300) -> (w1302:dbl[])
              }
            }
            n933 = property on="data" class="Arr (strict)"("Value"=w1296) -> ()  [unwired: 2 in, 2 out]
          }
          frame #25 {
            # "check if current on\nKeithley 2636A smua\nis to be measured"
            n934 = local read "2636A smua meas i"() -> (w1304:bool)
            n935 = property on="data" class="Arr (strict)"() -> ("Value"=w1305:dbl[])  [unwired: 2 in, 2 out]
            n936 = case shown="True" w1304 {
              tunnel: w1305 -> [w1307 w1310]
              tunnel: [w1307 w1309] -> w1306
              frame False {
                # "we are not measuring current on 2636A smua (2636A_smua_i)"
              }
              frame True {
                # "we are  measuring current on 2636A smua (2636A_smua_i)"
                n937 = stacked-sequence {
                  tunnel: [_ w1319] -> w1308
                  frame #0 {
                    n938 = local read "auto\nrange A"() -> (w1314:bool)
                    n939 = local read "2336A addr"() -> (w1317:refnum<visa-resource-name>)
                    n940 = Select(t="smua.AUTORANGE_ON", s=w1314, f="smua.AUTORANGE_OFF") -> (s? t:f=w1312:string)
                    n941 = Concatenate Strings("smua.measure.autorangei = ", w1312) -> (w1311:string)
                    n942 = VISA Write(VISA resource name=w1317, write buffer=w1311) -> ()  [unwired: 1 in, 3 out]
                  }
                  frame #1 {
                    n943 = local read "2336A addr"() -> (w1321:refnum<visa-resource-name>)
                    n944 = call "SinglePointMeasurement.vi"("Measure"=Measure."Current", "Channel"=Channel."a", "VISA resource name 2"=w1321) -> ("Measuremet"=w1319:dbl)  [unwired: 3 in, 4 out]
                  }
                }
                n945 = Build Array (concatenate)(w1310, w1308) -> (w1309:dbl[])
              }
            }
            n946 = property on="data" class="Arr (strict)"("Value"=w1306) -> ()  [unwired: 2 in, 2 out]
          }
          frame #26 {
            # "check if voltage on\nKeithley 2636A smub\nis to be measured"
            n947 = local read "2636A smub meas v"() -> (w1322:bool)
            n948 = property on="data" class="Arr (strict)"() -> ("Value"=w1323:dbl[])  [unwired: 2 in, 2 out]
            n949 = case shown="True" w1322 {
              tunnel: w1323 -> [w1325 w1331]
              tunnel: [w1325 w1330] -> w1324
              frame False {
                # "we are not measuring voltage on 2636A smub (2636A_smub_v)"
              }
              frame True {
                # "we are  measuring voltage on 2636A smub (2636A_smub_v)"
                n950 = local read "2336A addr"() -> (w1329:refnum<visa-resource-name>)
                n951 = call "SinglePointMeasurement.vi"("Measure"=Measure."Voltage", "Channel"=Channel."b", "VISA resource name 2"=w1329) -> ("Measuremet"=w1327:dbl)  [unwired: 3 in, 4 out]
                n952 = Build Array (concatenate)(w1331, w1327) -> (w1330:dbl[])
              }
            }
            n953 = property on="data" class="Arr (strict)"("Value"=w1324) -> ()  [unwired: 2 in, 2 out]
          }
          frame #27 {
            # "check if current on\nKeithley 2636A smub\nis to be measured"
            n954 = local read "2636A smub meas i"() -> (w1332:bool)
            n955 = property on="data" class="Arr (strict)"() -> ("Value"=w1333:dbl[])  [unwired: 2 in, 2 out]
            n956 = case shown="True" w1332 {
              tunnel: w1333 -> [w1335 w1338]
              tunnel: [w1335 w1337] -> w1334
              frame False {
                # "we are not measuring current on 2636A smub (2636A_smub_i)"
              }
              frame True {
                # "we are  measuring current on 2636A smub (2636A_smub_i)"
                n957 = stacked-sequence {
                  tunnel: [_ w1347] -> w1336
                  frame #0 {
                    n958 = local read "auto\nrange B"() -> (w1342:bool)
                    n959 = local read "2336A addr"() -> (w1345:refnum<visa-resource-name>)
                    n960 = Select(t="smub.AUTORANGE_ON", s=w1342, f="smub.AUTORANGE_OFF") -> (s? t:f=w1340:string)
                    n961 = Concatenate Strings("smub.measure.autorangei = ", w1340) -> (w1339:string)
                    n962 = VISA Write(VISA resource name=w1345, write buffer=w1339) -> ()  [unwired: 1 in, 3 out]
                  }
                  frame #1 {
                    n963 = local read "2336A addr"() -> (w1349:refnum<visa-resource-name>)
                    n964 = call "SinglePointMeasurement.vi"("Measure"=Measure."Current", "Channel"=Channel."b", "VISA resource name 2"=w1349) -> ("Measuremet"=w1347:dbl)  [unwired: 3 in, 4 out]
                  }
                }
                n965 = Build Array (concatenate)(w1338, w1336) -> (w1337:dbl[])
              }
            }
            n966 = property on="data" class="Arr (strict)"("Value"=w1334) -> ()  [unwired: 2 in, 2 out]
          }
          frame #28 {
            # "check if capacitance\nand loss on AH2500\nis to be measured"
            n967 = local read "AH2500 C and L"() -> (w1350:bool)
            n968 = property on="data" class="Arr (strict)"() -> ("Value"=w1351:dbl[])  [unwired: 2 in, 2 out]
            n969 = case shown="True" w1350 {
              tunnel: w1351 -> [w1353 w1360]
              tunnel: [w1353 w1354] -> w1352
              frame False {
                # "we are not measuring c and l from AH2500"
              }
              frame True {
                # "C"
                # "loss"
                # "we are  measuring c and l from AH2500"
                n970 = local read "AH2500 addr"() -> (w1359:u8)
                n971 = Number To Decimal String(number=w1359) -> (decimal integer string=w1358:string)  [unwired: 1 in]
                n972 = stacked-sequence {
                  seq-local: [w1363 _ _] -> [_ _ w1385]
                  tunnel: [_ _ w1379] -> w1355
                  tunnel: [_ _ w1380] -> w1357
                  tunnel: w1358 -> [w1362 w1365 w1374]
                  frame #0 {
                    # "causes bridge to take a single\nmeasurement"
                    n973 = GPIB Write(0:w1362, 1:"SINGLE" ("data"), 2:i16 0 ("mode (0)")) -> (6:w1363:errorcluster)  [unwired: 2 in, 1 out]
                  }
                  frame #1 {
                    n974 = while {
                      tunnel: w1365 -> [w1366]
                      stop <- w1368 continue-if-true
                      n975 = GPIB Serial Poll(0:w1366) -> (2:w1370:i16)  [unwired: 1 in, 2 out]
                      n976 = Less?(x=w1370, y=i16 128) -> (x < y?=w1368:bool)
                      n977 = Wait (ms)(milliseconds to wait=u32 50) -> ()  [unwired: 1 out]
                    }
                  }
                  frame #2 {
                    w1373 = i16 2 ("mode (0)")
                    n978 = GPIB Read(0:w1374, 1:200 ("byte count"), 2:i16 2 ("mode (0)"), 3:w1385, 4:20000 ("timeout ms (488.2 global)")) -> (5:w1378:string)  [unwired: 2 out]
                    n979 = Match Pattern(string=w1378, regular expression="C=") -> (after substring=w1377:string)  [unwired: 1 in, 3 out]
                    n980 = Match Pattern(string=w1377, regular expression="PF L=") -> (after substring=w1375:string)  [unwired: 1 in, 3 out]
                    n981 = Search/Split String(string=w1375, search string/char (-)=" ", offset (0)=w1373) -> (substring before match=w1381:string)  [unwired: 2 out]
                    n982 = Search/Split String(string=w1377, search string/char (-)=" ", offset (0)=w1373) -> (substring before match=w1382:string)  [unwired: 2 out]
                    n983 = Fract/Exp String To Number(string=w1381) -> (number=w1379:dbl)  [unwired: 3 in, 1 out]
                    n984 = Fract/Exp String To Number(string=w1382) -> (number=w1380:dbl)  [unwired: 3 in, 1 out]
                  }
                }
                n985 = Build Array (concatenate)(w1360, w1357) -> (w1356:dbl[])
                n986 = Build Array (concatenate)(w1356, w1355) -> (w1354:dbl[])
              }
            }
            n987 = property on="data" class="Arr (strict)"("Value"=w1352) -> ()  [unwired: 2 in, 2 out]
          }
          frame #29 {
            # "check if capacitance\nand loss on AH2700A\nis to be measured"
            n988 = local read "AH2700A C and L"() -> (w1388:bool)
            n989 = property on="data" class="Arr (strict)"() -> ("Value"=w1389:dbl[])  [unwired: 2 in, 2 out]
            n990 = case shown="True" w1388 {
              tunnel: w1389 -> [w1391 w1398]
              tunnel: [w1391 w1392] -> w1390
              frame False {
                # "we are not measuring c and l from AH2700A"
              }
              frame True {
                # "C"
                # "loss"
                # "we are  measuring c and l from AH2700A"
                n991 = local read "AH2700A addr"() -> (w1397:u8)
                n992 = Number To Decimal String(number=w1397) -> (decimal integer string=w1396:string)  [unwired: 1 in]
                n993 = stacked-sequence {
                  seq-local: [w1401 _ _] -> [_ _ w1422]
                  tunnel: [_ _ w1416] -> w1393
                  tunnel: [_ _ w1417] -> w1395
                  tunnel: w1396 -> [w1400 w1403 w1411]
                  frame #0 {
                    # "causes bridge to take a single\nmeasurement"
                    n994 = GPIB Write(0:w1400, 1:"SINGLE" ("data"), 2:i16 0 ("mode (0)")) -> (6:w1401:errorcluster)  [unwired: 2 in, 1 out]
                  }
                  frame #1 {
                    n995 = while {
                      tunnel: w1403 -> [w1404]
                      stop <- w1406 continue-if-true
                      n996 = GPIB Serial Poll(0:w1404) -> (2:w1408:i16)  [unwired: 1 in, 2 out]
                      n997 = Less?(x=w1408, y=i16 128) -> (x < y?=w1406:bool)
                      n998 = Wait (ms)(milliseconds to wait=u32 10) -> ()  [unwired: 1 out]
                    }
                  }
                  frame #2 {
                    w1410 = i16 2 ("mode (0)")
                    n999 = GPIB Read(0:w1411, 1:200 ("byte count"), 2:i16 2 ("mode (0)"), 3:w1422) -> (5:w1415:string)  [unwired: 1 in, 2 out]
                    n1000 = Match Pattern(string=w1415, regular expression="C=") -> (after substring=w1414:string)  [unwired: 1 in, 3 out]
                    n1001 = Match Pattern(string=w1414, regular expression="PF L=") -> (after substring=w1412:string)  [unwired: 1 in, 3 out]
                    n1002 = Search/Split String(string=w1412, search string/char (-)=" ", offset (0)=w1410) -> (substring before match=w1418:string)  [unwired: 2 out]
                    n1003 = Search/Split String(string=w1414, search string/char (-)=" ", offset (0)=w1410) -> (substring before match=w1419:string)  [unwired: 2 out]
                    n1004 = Fract/Exp String To Number(string=w1418) -> (number=w1416:dbl)  [unwired: 3 in, 1 out]
                    n1005 = Fract/Exp String To Number(string=w1419) -> (number=w1417:dbl)  [unwired: 3 in, 1 out]
                  }
                }
                n1006 = Build Array (concatenate)(w1398, w1395) -> (w1394:dbl[])
                n1007 = Build Array (concatenate)(w1394, w1393) -> (w1392:dbl[])
              }
            }
            n1008 = property on="data" class="Arr (strict)"("Value"=w1390) -> ()  [unwired: 2 in, 2 out]
          }
          frame #30 {
            # "check if temperature \non LS340 input A\nis to be measured"
            n1009 = property on="data" class="Arr (strict)"() -> ("Value"=w1426:dbl[])  [unwired: 2 in, 2 out]
            n1010 = local read "LS340 A"() -> (w1425:bool)
            n1011 = case shown="True" w1425 {
              tunnel: w1426 -> [w1428 w1437]
              tunnel: [w1428 w1435] -> w1427
              frame False {
                # "we are not measuring temperature in K on LS340 input A (LS340_A)"
              }
              frame True {
                # "input A temperature, K"
                # "we are measuring temperature in K on LS340 input A (LS340_A)"
                n1012 = local read "LS340 addr"() -> (w1436:u8)
                n1013 = Number To Decimal String(number=w1436) -> (decimal integer string=w1431:string)  [unwired: 1 in]
                n1014 = GPIB Write(0:w1431, 1:"KRDG? A") -> (6:w1433:errorcluster)  [unwired: 3 in, 1 out]
                n1015 = GPIB Read(0:w1431, 1:120, 3:w1433) -> (5:w1430:string)  [unwired: 2 in, 2 out]
                n1016 = Fract/Exp String To Number(string=w1430) -> (number=w1429:dbl)  [unwired: 3 in, 1 out]
                n1017 = Build Array (concatenate)(w1437, w1429) -> (w1435:dbl[])
              }
            }
            n1018 = property on="data" class="Arr (strict)"("Value"=w1427) -> ()  [unwired: 2 in, 2 out]
          }
          frame #31 {
            # "check if temperature \non LS340 input B\nis to be measured"
            n1019 = property on="data" class="Arr (strict)"() -> ("Value"=w1439:dbl[])  [unwired: 2 in, 2 out]
            n1020 = local read "LS340 B"() -> (w1438:bool)
            n1021 = case shown="True" w1438 {
              tunnel: w1439 -> [w1441 w1450]
              tunnel: [w1441 w1448] -> w1440
              frame False {
                # "we are not measuring temperature in K on LS340 input B (LS340_B)"
              }
              frame True {
                # "input B temperature, K"
                # "we are measuring temperature in K on LS340 input B (LS340_B)"
                n1022 = local read "LS340 addr"() -> (w1449:u8)
                n1023 = Number To Decimal String(number=w1449) -> (decimal integer string=w1444:string)  [unwired: 1 in]
                n1024 = GPIB Write(0:w1444, 1:"KRDG? B") -> (6:w1446:errorcluster)  [unwired: 3 in, 1 out]
                n1025 = GPIB Read(0:w1444, 1:120, 3:w1446) -> (5:w1443:string)  [unwired: 2 in, 2 out]
                n1026 = Fract/Exp String To Number(string=w1443) -> (number=w1442:dbl)  [unwired: 3 in, 1 out]
                n1027 = Build Array (concatenate)(w1450, w1442) -> (w1448:dbl[])
              }
            }
            n1028 = property on="data" class="Arr (strict)"("Value"=w1440) -> ()  [unwired: 2 in, 2 out]
          }
          frame #32 {
            # "check if temperature \non LS332 input A\nis to be measured"
            n1029 = property on="data" class="Arr (strict)"() -> ("Value"=w1452:dbl[])  [unwired: 2 in, 2 out]
            n1030 = local read "LS332 A"() -> (w1451:bool)
            n1031 = case shown="True" w1451 {
              tunnel: w1452 -> [w1454 w1467]
              tunnel: [w1454 w1466] -> w1453
              frame False {
                # "we are not measuring temperature in K on LS332 input A (LS332_A)"
              }
              frame True {
                # "we are measuring temperature in K on LS332 input A (LS332_A)"
                n1032 = Concatenate Strings("READ:DEV:MB1.T1:TEMP:SIG:TEMP" ("string"), "\r", "\n") -> (w1463:string)
                n1033 = VISA Write(VISA resource name="MercuryITC", write buffer=w1463) -> (VISA resource name out=w1458:refnum<visa-resource-name>, error out=w1459:errorcluster)  [unwired: 1 in, 1 out]
                n1034 = VISA Read(VISA resource name=w1458, byte count=u32 1024, error in (no error)=w1459) -> (read buffer=w1464:string)  [unwired: 3 out]
                n1035 = Fract/Exp String To Number(string=w1464, offset=30) -> (number=w1455:dbl)  [unwired: 2 in, 1 out]
                n1036 = Build Array (concatenate)(w1467, w1455) -> (w1466:dbl[])
              }
            }
            n1037 = property on="data" class="Arr (strict)"("Value"=w1453) -> ()  [unwired: 2 in, 2 out]
          }
          frame #33 {
            # "check if temperature \non LS332 input B\nis to be measured"
            n1038 = property on="data" class="Arr (strict)"() -> ("Value"=w1469:dbl[])  [unwired: 2 in, 2 out]
            n1039 = local read "LS332 B"() -> (w1468:bool)
            n1040 = case shown="True" w1468 {
              tunnel: w1469 -> [w1471 w1480]
              tunnel: [w1471 w1478] -> w1470
              frame False {
                # "we are not measuring temperature in K on LS332 input B (LS332_B)"
              }
              frame True {
                # "input B temperature, K"
                # "we are measuring temperature in K on LS332 input B (LS332_B)"
                n1041 = local read "LS332 addr"() -> (w1479:u8)
                n1042 = Number To Decimal String(number=w1479) -> (decimal integer string=w1474:string)  [unwired: 1 in]
                n1043 = GPIB Write(0:w1474, 1:"KRDG? B") -> (6:w1476:errorcluster)  [unwired: 3 in, 1 out]
                n1044 = GPIB Read(0:w1474, 1:120, 3:w1476) -> (5:w1473:string)  [unwired: 2 in, 2 out]
                n1045 = Fract/Exp String To Number(string=w1473) -> (number=w1472:dbl)  [unwired: 3 in, 1 out]
                n1046 = Build Array (concatenate)(w1480, w1472) -> (w1478:dbl[])
              }
            }
            n1047 = property on="data" class="Arr (strict)"("Value"=w1470) -> ()  [unwired: 2 in, 2 out]
          }
          frame #34 {
            # "check if time\nis to be measured"
            n1048 = property on="data" class="Arr (strict)"() -> ("Value"=w1484:dbl[])  [unwired: 2 in, 2 out]
            n1049 = local read "measure time"() -> (w1483:bool)
            n1050 = case shown="True" w1483 {
              tunnel: w1484 -> [w1486 w1492]
              tunnel: [w1486 w1491] -> w1485
              tunnel: w1482 -> [_ w1488]
              frame False {
                # "we are not measuring time"
              }
              frame True {
                # "seconds from the beginning of month"
                # "we are  measuring time"
                n1051 = call "timeInSeconds.vi"() -> ("Numeric"=w1489:dbl, "current time"=→"current time":timestamp)  [unwired: 2 in]
                n1052 = Subtract(x=w1489, y=w1488) -> (x-y=w1487:dbl)
                n1053 = Build Array (concatenate)(w1492, w1487) -> (w1491:dbl[])
              }
            }
            n1054 = property on="data" class="Arr (strict)"("Value"=w1485) -> ()  [unwired: 2 in, 2 out]
          }
          frame #35 {
            # "check if 1st channel \non Keithley 2182A 5\nis to be used\nto measure \nHULK SMS output"
            n1055 = local read "Hulk_B_meas (Vnano)"() -> (w1493:bool)
            n1056 = property on="data" class="Arr (strict)"() -> ("Value"=w1494:dbl[])  [unwired: 2 in, 2 out]
            n1057 = case shown="True" w1493 {
              tunnel: w1494 -> [w1496 w1509]
              tunnel: [w1496 w1508] -> w1495
              frame False {
                # "we are not using 2182A 5 channel 1 to measure HULK SMS field"
              }
              frame True {
                (unwired) 0.13783  # T/A
                (unwired) 0.051121833  # V/A
                # "temporarily remove \ncoefficients\nneed recalibration"
                # "2182A 5 channel 1 to measure HULK SMS field"
                n1058 = local read "2182A 5 addr"() -> (w1504:u8)
                n1059 = Number To Decimal String(number=w1504) -> (decimal integer string=w1503:string)  [unwired: 1 in]
                n1060 = GPIB Write(0:w1503, 1:":SENSe:DATA:FRES?") -> (6:w1507:errorcluster)  [unwired: 3 in, 1 out]
                n1061 = GPIB Read(0:w1503, 1:200, 3:w1507) -> (5:w1502:string)  [unwired: 2 in, 2 out]
                n1062 = Fract/Exp String To Number(string=w1502) -> (number=w1501:dbl)  [unwired: 3 in, 1 out]
                n1063 = Divide "A"(x=w1501, y=1.0) -> (x/y=w1500:dbl)
                n1064 = Multiply "T"(x=1.0, y=w1500) -> (x*y=w1499:dbl)
                n1065 = Build Array (concatenate)(w1509, w1499) -> (w1508:dbl[])
              }
            }
            n1066 = property on="data" class="Arr (strict)"("Value"=w1495) -> ()  [unwired: 2 in, 2 out]
          }
          frame #36 {
            n1067 = local read "MercuryIPS"() -> (w1510:bool)
            n1068 = property on="data" class="Arr (strict)"() -> ("Value"=w1511:dbl[])  [unwired: 2 in, 2 out]
            n1069 = case shown="True" w1510 {
              tunnel: w1511 -> [w1513 w1534]
              tunnel: [w1513 w1533] -> w1512
              frame False {
                # "we are not Measuring magnetic field on IPS120-0"
              }
              frame True {
                # "Measure magnetic field on MercuryIPS"
                n1070 = VISA Clear(VISA resource name="MercuryIPS") -> (VISA resource name out=w1516:refnum<visa-resource-name>, error out=w1515:errorcluster)  [unwired: 1 in]
                n1071 = Concatenate Strings("READ:DEV:GRPZ:PSU" ("string"), "\r", "\n") -> (w1529:string)
                n1072 = VISA Write(VISA resource name=w1516, write buffer=w1529, error in (no error)=w1515) -> (VISA resource name out=w1518:refnum<visa-resource-name>, error out=w1519:errorcluster)  [unwired: 1 out]
                n1073 = VISA Read(VISA resource name=w1518, byte count=u32 450, error in (no error)=w1519) -> (read buffer=w1520:string, error out=→"MercuryIPS_Error":errorcluster)  [unwired: 2 out]
                "read buffer MercuryIPS" <- w1520
                n1074 = Match Pattern(string=w1520, regular expression=":PCUR:") -> (after substring=w1525:string)  [unwired: 1 in, 3 out]
                n1075 = Match Pattern(string=w1520, regular expression=":ATOB:") -> (after substring=w1527:string)  [unwired: 1 in, 3 out]
                n1076 = Fract/Exp String To Number(string=w1525) -> (number=w1524:dbl)  [unwired: 3 in, 1 out]
                n1077 = Fract/Exp String To Number(string=w1527) -> (number=w1523:dbl)  [unwired: 3 in, 1 out]
                n1078 = Divide(x=w1524, y=w1523) -> (x/y=w1522:dbl)
                n1079 = Build Array (concatenate)(w1534, w1522) -> (w1533:dbl[])
              }
            }
            n1080 = property on="data" class="Arr (strict)"("Value"=w1512) -> ()  [unwired: 2 in, 2 out]
          }
          frame #37 {
            # "check if LT bridge\nis used to measure\ncapacitance"
            n1081 = local read "LT bridge\ncalibration"() -> (w1537:bool)
            n1082 = property on="data" class="Arr (strict)"() -> ("Value"=w1539:dbl[])  [unwired: 2 in, 2 out]
            n1083 = local read "LT bridge"() -> (w1536:bool)
            n1084 = Not(x=w1537) -> (.not. x?=w1538:bool)
            n1085 = And(x=w1536, y=w1538) -> (x .and. y?=w1535:bool)
            n1086 = case shown="True" w1535 {
              tunnel: w1539 -> [w1541 w1548]
              tunnel: [w1541 w1549] -> w1540
              frame False {
                # "we are not measuring capacitance with LT bridge on chip"
              }
              frame True {
                # "we are  measuring capacitance with LT bridge on chip"
                n1087 = local read "k, pF/V"() -> (w1543:dbl)
                n1088 = local read "b, pF"() -> (w1542:dbl)
                n1089 = Index Array(array=w1548, index=1) -> (element=w1546:dbl)
                n1090 = Multiply(x=w1546, y=w1543) -> (x*y=w1545:dbl)
                n1091 = Add(x=w1545, y=w1542) -> (x+y=w1544:dbl)
                n1092 = Build Array (concatenate)(w1548, w1544) -> (w1549:dbl[])
              }
            }
            n1093 = property on="data" class="Arr (strict)"("Value"=w1540) -> ()  [unwired: 2 in, 2 out]
          }
          frame #38 {
            # "measure DC resistance\n(commuting)"
            n1094 = property on="data" class="Arr (strict)"() -> ("Value"=w1554:dbl[])  [unwired: 2 in, 2 out]
            n1095 = local read "DC_resistance"() -> (w1552:bool)
            n1096 = local read "2400 2 addr"() -> (w1563:u8)
            n1097 = local read "2182A 1 addr"() -> (w1560:u8)
            n1098 = local read "2182A 2 addr"() -> (w1559:u8)
            n1099 = local read "2182A 3 addr"() -> (w1561:u8)
            n1100 = local read "2182A 4 addr"() -> (w1562:u8)
            n1101 = local read "2182A 4"() -> (w1558:bool)
            n1102 = local read "2182A 3"() -> (w1557:bool)
            n1103 = local read "2182A 2"() -> (w1556:bool)
            n1104 = local read "2182A 1"() -> (w1555:bool)
            n1105 = call "DCcommute.vi"("data in"=w1554, "DC_resistance"=w1552, "DC bias pos (V)"="DC bias pos (V)", "wait to set voltage, msec"="wait to set voltage, msec", "2400 2 addr"=w1563, "DC bias neg (V)"="DC bias neg (V)", "2182A 1"=w1555, "2182A 1 addr"=w1560, "2182A 2"=w1556, "2182A 2 addr"=w1559, "2182A 3"=w1557, "2182A 3 addr"=w1561, "2182A 4"=w1558, "2182A 4 addr"=w1562) -> ("data out"=w1553:dbl[])  [unwired: 5 in]
            n1106 = property on="data" class="Arr (strict)"("Value"=w1553) -> ()  [unwired: 2 in, 2 out]
          }
        }
      }
      frame #4 {
        # "this part appends last\nmeasured point to the \ndata file"
        n1107 = local read "Data file:"() -> (w1566:path)
        n1108 = property on="data" class="Arr (strict)"() -> ("Value"=w1565:dbl[])  [unwired: 2 in, 2 out]
        n1109 = call-poly <vilib>:"Write To Spreadsheet File.vi"("format (%.3f)"="%.6e", "append to file? (new file:F)"=TRUE, "1D data"=w1565, "file path (dialog if empty)"=w1566) -> ()  [unwired: 4 in, 1 out]
      }
    }
    n1110 = local read "LT bridge\ncalibration"() -> (w828:bool)
    n1111 = case shown="True" w828 {
      tunnel: w827 -> [_ w869]
      tunnel: w826 -> [_ _]
      tunnel: w825 -> [w851 w866]
      tunnel: [w851 w865] -> w824
      frame False {
      }
      frame True {
        w861 = u16 2 items=["Least Square", "Least Absolute Residual", "Bisquare"] ("method")
        # "this part calibrates LT bridge for next sweep"
        n1112 = Quotient & Remainder(x=w869, y="points") -> (x-y*floor(x/y)=w852:i32)  [unwired: 1 out]
        "x-y*floor(x/y)" <- w852
        n1113 = Equal To 0?(x=w852) -> (x = 0?=w867:bool)
        n1114 = case shown="True" w867 {
          tunnel: w866 -> [w870 w875]
          tunnel: [w870 w873] -> w865
          frame False {
          }
          frame True {
            n1115 = local read "SR830 1 addr"() -> (w879:u8)
            n1116 = local read "SR830 2 addr"() -> (w878:u8)
            n1117 = call "LTbridgeOnChipCalibration.vi"("C ref, pF"="C ref, pF", "V exc sample"="V exc sample", "SR830 1 addr"=w879, "pm"="pm", "V exc ref (SR830_2)"="V exc ref (SR830_2)", "SR830 2 addr"=w878) -> ("Array"=→"XY Graph 2":cluster{dbl[], "Best Linear Fit":dbl[]}[], "Numeric 2"=w876:dbl, "Numeric"=w877:dbl, "R-square"=→"R-square":dbl)  [unwired: 2 in]
            "C sample, pF" <- w876
            "off-zero voltage" <- w877
            n1118 = Build Array(w877, w876) -> (w874:dbl[])
            n1119 = Build Array (concatenate)(w875, w874) -> (w873:dbl[][])
          }
        }
        n1120 = Index Array(array=w865, index (col)=0 ("disabled index (col)")) -> (element=w860:dbl[])  [unwired: 1 in]
        n1121 = Index Array(array=w865, index (col)=1 ("disabled index (col)")) -> (element=w858:dbl[])  [unwired: 1 in]
        n1122 = Bundle("emty array for LT bridge calibration"=w860, "emty array for LT bridge calibration"=w858) -> (w862:T9)  [unwired: 1 in]
        n1123 = call <vilib>:"Linear Fit.vi"("Y"=w858, "X"=w860, "method"=w861) -> ("Best Linear Fit"=w859:dbl[], "slope"=→"slope":dbl, "intercept"=→"intercept":dbl)  [unwired: 8 in, 2 out]
        n1124 = call <vilib>:"Goodness of Fit.vi"("Best Fit"=w859, "Y"=w858) -> ("R-square"=→"R-square total":dbl)  [unwired: 6 in, 3 out]
        n1125 = Bundle("emty array for LT bridge calibration"=w860, "Best Linear Fit"=w859) -> (w857:T10)  [unwired: 1 in]
        n1126 = Build Array(w862, w857) -> (→"XY Graph":T2)
      }
    }
    n1127 = stacked-sequence "add data to array" {
      tunnel: w849 -> [w1630]
      tunnel: [w1630] -> w848
      tunnel: w847 -> [w1629]
      tunnel: [w1627] -> w846
      frame #0 {
        n1128 = property on="data" class="Arr (strict)"() -> ("Value"=w1628:dbl[])  [unwired: 2 in, 2 out]
        n1129 = Build Array (concatenate)(w1629, w1628) -> (w1627:dbl[][])
      }
    }
    n1130 = And(x=w826, y="continuous") -> (x .and. y?=w832:bool)
    n1131 = stacked-sequence "plot selected measurements" {
      seq-local: [_ w1639 _] -> [_ _ w1672]
      seq-local: [_ w1638 _] -> [_ _ w1670]
      tunnel: w848 -> [_ _ w1668]
      tunnel: w846 -> [_ w1643 _]
      tunnel: [_ _ w1668] -> w831
      frame #0 {
        n1132 = local read "Yaxis"() -> (w1632:u16)
        n1133 = local read "Xaxis"() -> (w1636:u16)
        n1134 = property on="XY Graph" class="XYGraph (strict)"("Cursor.Visible"="Show cursor") -> ()  [unwired: 2 in, 2 out]
        n1135 = property on="Figure_axis" class="Arr (strict)"() -> ("Value"=w1631:string[])  [unwired: 2 in, 2 out]
        n1136 = property on="Figure_axis" class="Arr (strict)"() -> ("Value"=w1635:string[])  [unwired: 2 in, 2 out]
        n1137 = Index Array(array=w1631, index=w1632) -> (element=w1633:string)
        n1138 = Index Array(array=w1635, index=w1636) -> (element=w1637:string)
        n1139 = property on="XY Graph" class="XYGraph (strict)"("YScale.NameLbl.Text"=w1633) -> ()  [unwired: 2 in, 2 out]
        n1140 = property on="XY Graph" class="XYGraph (strict)"("XScale.NameLbl.Text"=w1637) -> ()  [unwired: 2 in, 2 out]
      }
      frame #1 {
        n1141 = property on="Xaxis" class="Ring (strict)"() -> ("RingText.Text"=w1641:string)  [unwired: 2 in, 2 out]
        n1142 = property on="Yaxis" class="Ring (strict)"() -> ("RingText.Text"=w1640:string)  [unwired: 2 in, 2 out]
        n1143 = local read "Xaxis"() -> (w1642:u16)
        n1144 = local read "Yaxis"() -> (w1645:u16)
        n1145 = case shown="\"formula\"" w1641 {
          tunnel: [w1661 w1664] -> w1647
          tunnel: w1642 -> [w1660 _]
          tunnel: w1643 -> [w1659 w1666]
          tunnel: [errorcluster {"status"=FALSE, "code"=0, "source"=""} ("error out") w1662] -> w1639
          frame "0", Default {
            n1146 = Index Array(array=w1659, index (col)=w1660) -> (element=w1661:dbl[])  [unwired: 1 in]
          }
          frame "formula" {
            n1147 = local read "formula_variables"() -> (w1665:string[])
            n1148 = Transpose 2D Array(2D array=w1666) -> (transposed array=w1663:dbl[][])
            n1149 = call <vilib>:"Eval Multi-Variable Array.vi"("Variables"=w1665, "X Values"=w1663, "formula"="X_axis_formula") -> ("error out"=w1662:errorcluster, "Y Values"=w1664:dbl[])  [unwired: 1 in]
          }
        }
        n1150 = case shown="\"formula\"" w1640 {
          tunnel: [w1649 w1657] -> w1646
          tunnel: w1645 -> [_ w1656]
          tunnel: w1643 -> [w1650 w1655]
          tunnel: [w1648 errorcluster {"status"=FALSE, "code"=0, "source"=""} ("error out")] -> w1638
          frame "formula" {
            n1151 = local read "formula_variables"() -> (w1652:string[])
            n1152 = Transpose 2D Array(2D array=w1650) -> (transposed array=w1653:dbl[][])
            n1153 = call <vilib>:"Eval Multi-Variable Array.vi"("Variables"=w1652, "X Values"=w1653, "formula"="Y_axis_formula") -> ("error out"=w1648:errorcluster, "Y Values"=w1649:dbl[])  [unwired: 1 in]
          }
          frame "0", Default {
            n1154 = Index Array(array=w1655, index (col)=w1656) -> (element=w1657:dbl[])  [unwired: 1 in]
          }
        }
        n1155 = Bundle("Y Values"=w1647, "Y Values"=w1646) -> (→"XY Graph":cluster{"Y Values":dbl[], "Y Values":dbl[]})  [unwired: 1 in]
      }
      frame #2 {
        # "show if formula \nis wrong"
        n1156 = Unbundle By Name(w1670) -> ("status"=→"status 2":bool)
        n1157 = Unbundle By Name(w1672) -> ("status"=→"status":bool)
      }
    }
    n1158 = case shown="True" w832 {
      tunnel: w831 -> [w884 w885]
      tunnel: [w884 w885] -> w830
      frame False {
      }
      frame True {
        n1159 = local read "sweep to:"() -> (w886:dbl)
        n1160 = Equal?(x=w886, y="upper limit") -> (x = y?=w887:bool)
        n1161 = Select(t="lower limit", s=w887, f="upper limit") -> (s? t:f=w890:dbl)
        n1162 = local write "sweep to:"(w890) -> ()
      }
    }
    n1163 = case shown="True" "oldStyle" {
      selector: "oldStyle" -> [w892 w895]
      tunnel: [w892 w894] -> w838
      tunnel: w831 -> [w891 w893]
      tunnel: [w891 w893] -> w837
      tunnel: w830 -> [_ _]
      frame False {
      }
      frame True {
        n1164 = stacked-sequence {
          tunnel: w895 -> [_ _ w899]
          tunnel: [_ _ w899] -> w894
          frame #0 {
            n1165 = property on="Pause" class="Bool (strict)"("Visible"=TRUE) -> ()  [unwired: 2 in, 2 out]
          }
          frame #1 {
            n1166 = while {
              stop <- "Pause" continue-if-true
              n1167 = Wait (ms)(milliseconds to wait=u32 10) -> ()  [unwired: 1 out]
            }
          }
          frame #2 {
            n1168 = local write "Pause"(FALSE ("Pause")) -> ()
          }
        }
      }
    }
    n1169 = And(x=w826, y=w838) -> (x .and. y?=w840:bool)
    n1170 = case shown="False" w840 {
      tunnel: w826 -> [w902 _]
      tunnel: [w902 w904] -> w835
      tunnel: w837 -> [w901 w903]
      tunnel: [w901 w903] -> w836
      frame False {
      }
      frame True {
        n1171 = stacked-sequence {
          tunnel: [_ _ w913] -> w904
          frame #0 {
            w905 = TRUE ("Visible")
            w906 = FALSE ("ready/go")
            n1172 = local write "ready/go"(w906) -> ()
            n1173 = local write "stop"(w906) -> ()
            n1174 = property on="ready/go" class="Bool (strict)"("Visible"=w905) -> ()  [unwired: 2 in, 2 out]
            n1175 = property on="stop" class="Bool (strict)"("Visible"=w905) -> ()  [unwired: 2 in, 2 out]
          }
          frame #1 {
            n1176 = while {
              stop <- w908 stop-if-true
              # "wait for ready/go\nor stop"
              n1177 = local read "ready/go"() -> (w910:bool)
              n1178 = local read "stop"() -> (w907:bool)
              n1179 = Or(x=w907, y=w910) -> (x .or. y?=w908:bool)
              n1180 = Wait (ms)(milliseconds to wait=u32 50) -> ()  [unwired: 1 out]
            }
          }
          frame #2 {
            w912 = FALSE ("Visible")
            w911 = FALSE ("ready/go")
            n1181 = local write "ready/go"(w911) -> ()
            n1182 = local write "Pause"(w911) -> ()
            n1183 = property on="Pause" class="Bool (strict)"("Visible"=w912) -> ()  [unwired: 2 in, 2 out]
            n1184 = property on="stop" class="Bool (strict)"("Visible"=w912) -> ()  [unwired: 2 in, 2 out]
            n1185 = local read "stop"() -> (w913:bool)
            n1186 = property on="ready/go" class="Bool (strict)"("Visible"=w912) -> ()  [unwired: 2 in, 2 out]
          }
        }
      }
    }
    n1187 = stacked-sequence "set next value in the sweep" {
      tunnel: w845 -> [w1573 _]
      tunnel: [w1573 _] -> w844
      tunnel: w842 -> [_ w1621]
      tunnel: w836 -> [_ _]
      frame #0 {
        # "7 = HULK SMS\n8 = Mercury_IPS"
        # "1 = 2400 1\n2 = 2400 2\n3 = 2400 3\n4 = 2636a smua\n5 = 2636a smub\n6 = do not sweep, just time"
        n1188 = local read "sweep"() -> (w1575:T3)
        n1189 = Multiply(x="Slope", y=w1573) -> (x*y=w1570:dbl)
        n1190 = Add(x="Offset", y=w1570) -> (x+y=w1571:dbl)
        n1191 = case shown="True" "Double Sweep" {
          tunnel: w1571 -> [_ w1576]
          frame False {
          }
          frame True {
            n1192 = disable-structure shown="Enabled" {
              disable-tunnel: w1576 -> [w1577 w1584]
              frame Disabled {
                # "sweep voltage on 2400 2"
                n1193 = local read "2400 2 addr"() -> (w1578:u8)
                n1194 = Number To Fractional String(number=w1577) -> (F-format string=w1579:string)  [unwired: 3 in]
                n1195 = Concatenate Strings(":INIT:IMM; :SOUR:VOLT:LEV:IMM:AMPL " ("data"), w1579) -> (w1581:string)
                n1196 = Number To Decimal String(number=w1578) -> (decimal integer string=w1582:string)  [unwired: 1 in]
                n1197 = GPIB Write(0:w1582, 1:w1581, 2:i16 1 ("mode (0)")) -> ()  [unwired: 2 in, 2 out]
              }
              frame Enabled {
                n1198 = local read "2336A addr"() -> (w1587:refnum<visa-resource-name>)
                n1199 = call "setLevel.vi"("VISA resource name 2"=w1587, "Source"=Source."Voltage", "Channel"="Slave Channel", "SourceLevel"=w1584) -> ()  [unwired: 1 in, 3 out]
              }
            }
          }
        }
        n1200 = case shown="\"Radio Selection 1\"" w1575 {
          tunnel: w1573 -> [w1588 w1595 w1602 w1612 w1616 _ w1617]
          frame "Radio Selection 1" {
            # "sweep voltage on 2400 1"
            n1201 = local read "2400 1 addr"() -> (w1590:u8)
            n1202 = Number To Fractional String(number=w1588) -> (F-format string=w1594:string)  [unwired: 3 in]
            n1203 = Concatenate Strings(":INIT:IMM; :SOUR:VOLT:LEV:IMM:AMPL " ("data"), w1594) -> (w1592:string)
            n1204 = Number To Decimal String(number=w1590) -> (decimal integer string=w1589:string)  [unwired: 1 in]
            n1205 = GPIB Write(0:w1589, 1:w1592, 2:i16 1 ("mode (0)")) -> ()  [unwired: 2 in, 2 out]
          }
          frame "Radio Selection 2" {
            # "sweep voltage on 2400 2"
            n1206 = Number To Fractional String(number=w1595) -> (F-format string=w1601:string)  [unwired: 3 in]
            n1207 = local read "2400 2 addr"() -> (w1597:u8)
            n1208 = Concatenate Strings(":INIT:IMM; :SOUR:VOLT:LEV:IMM:AMPL " ("data"), w1601) -> (w1599:string)
            n1209 = Number To Decimal String(number=w1597) -> (decimal integer string=w1596:string)  [unwired: 1 in]
            n1210 = GPIB Write(0:w1596, 1:w1599, 2:i16 1 ("mode (0)")) -> ()  [unwired: 2 in, 2 out]
          }
          frame "Radio Selection 3" {
            # "sweep voltage on 2400 3"
            n1211 = local read "2400 3 addr"() -> (w1604:u8)
            n1212 = Number To Fractional String(number=w1602) -> (F-format string=w1608:string)  [unwired: 3 in]
            n1213 = Concatenate Strings(":INIT:IMM; :SOUR:VOLT:LEV:IMM:AMPL " ("data"), w1608) -> (w1606:string)
            n1214 = Number To Decimal String(number=w1604) -> (decimal integer string=w1603:string)  [unwired: 1 in]
            n1215 = GPIB Write(0:w1603, 1:w1606, 2:i16 1 ("mode (0)")) -> ()  [unwired: 2 in, 2 out]
          }
          frame "Radio Selection 4" {
            # "sweep voltage on 2636a smua"
            n1216 = local read "2336A addr"() -> (w1610:refnum<visa-resource-name>)
            n1217 = call "setLevel.vi"("VISA resource name 2"=w1610, "Source"=Source."Voltage", "Channel"=Channel."a", "SourceLevel"=w1612) -> ()  [unwired: 1 in, 3 out]
          }
          frame "Radio Selection 5" {
            # "sweep voltage on 2636b smua"
            n1218 = local read "2336A addr"() -> (w1613:refnum<visa-resource-name>)
            n1219 = call "setLevel.vi"("VISA resource name 2"=w1613, "Source"=Source."Voltage", "Channel"=Channel."b", "SourceLevel"=w1616) -> ()  [unwired: 1 in, 3 out]
          }
          frame "Radio Selection 6", Default {
            # "do not sweep, just time"
          }
          frame "Radio Selection 8" {
            n1220 = local read "MercuryIPS"() -> (w1618:refnum<visa-resource-name>)
            n1221 = call "MercuryIPSsput4SetField.vi"("FieldSetpoint"=w1617, "MercuryIPS"=w1618) -> ("error out"=w1619:errorcluster)
            n1222 = local write "MercuryIPS_Error"(w1619) -> ()
          }
        }
        "sweep value" <- w1573
      }
      frame #1 {
        # "calculate deliberate time delay for the next step"
        n1223 = Tick Count (ms)() -> (millisecond timer value=w1624:u32)
        n1224 = Subtract(x=w1624, y=w1621) -> (x-y=w1623:u32)
        n1225 = property on="time/point, sec" class="DigNum (strict)"() -> ("Value"=w1625:dbl)  [unwired: 2 in, 2 out]
        n1226 = Multiply(x=w1625, y=1000.0) -> (x*y=w1620:dbl)
        n1227 = Subtract(x=w1620, y=w1623) -> (x-y=→"time delay, ms":dbl)
      }
    }
    n1228 = Not(x="continuous") -> (.not. x?=w829:bool)
    n1229 = And(x=w835, y=w829) -> (x .and. y?=w834:bool)
  }
  n1230 = stacked-sequence {
    tunnel: w5 -> [_ _ _]
    frame #0 {
      w1673 = T6."Enabled" ("Disabled")
      w1674 = T6."Enabled" ("Disabled")
      n1231 = property on="AH2500 addr" class="DigNum (strict)"("DisabledEnum"=w1674) -> ()  [unwired: 2 in, 2 out]
      n1232 = property on="LS340 addr" class="DigNum (strict)"("DisabledEnum"=w1674) -> ()  [unwired: 2 in, 2 out]
      n1233 = property on="sweep" class="RadioBtnsControl (strict)"("DisabledEnum"=w1674) -> ()  [unwired: 2 in, 2 out]
      n1234 = property on="2182A 1 addr" class="DigNum (strict)"("DisabledEnum"=w1674) -> ()  [unwired: 2 in, 2 out]
      n1235 = property on="2182A 2 addr" class="DigNum (strict)"("DisabledEnum"=w1674) -> ()  [unwired: 2 in, 2 out]
      n1236 = property on="2182A 3 addr" class="DigNum (strict)"("DisabledEnum"=w1674) -> ()  [unwired: 2 in, 2 out]
      n1237 = property on="2182A 4 addr" class="DigNum (strict)"("DisabledEnum"=w1674) -> ()  [unwired: 2 in, 2 out]
      n1238 = property on="2400 1 addr" class="DigNum (strict)"("DisabledEnum"=w1674) -> ()  [unwired: 2 in, 2 out]
      n1239 = property on="SR830 5 addr" class="DigNum (strict)"("DisabledEnum"=w1674) -> ()  [unwired: 2 in, 2 out]
      n1240 = property on="AH2700A addr" class="DigNum (strict)"("DisabledEnum"=w1674) -> ()  [unwired: 2 in, 2 out]
      n1241 = property on="LS332 addr" class="DigNum (strict)"("DisabledEnum"=w1674) -> ()  [unwired: 2 in, 2 out]
      n1242 = property on="2400 2 addr" class="DigNum (strict)"("DisabledEnum"=w1674) -> ()  [unwired: 2 in, 2 out]
      n1243 = property on="2400 3 addr" class="DigNum (strict)"("DisabledEnum"=w1674) -> ()  [unwired: 2 in, 2 out]
      n1244 = property on="2336A addr" class="VISAName"("DisabledEnum"=w1674) -> ()  [unwired: 2 in, 2 out]
      n1245 = property on="SR830 1 addr" class="DigNum (strict)"("DisabledEnum"=w1674) -> ()  [unwired: 2 in, 2 out]
      n1246 = property on="SR830 2 addr" class="DigNum (strict)"("DisabledEnum"=w1674) -> ()  [unwired: 2 in, 2 out]
      n1247 = property on="SR830 3 addr" class="DigNum (strict)"("DisabledEnum"=w1674) -> ()  [unwired: 2 in, 2 out]
      n1248 = property on="SR830 4 addr" class="DigNum (strict)"("DisabledEnum"=w1674) -> ()  [unwired: 2 in, 2 out]
      n1249 = property on="sweep to:" class="DigNum (strict)"("DisabledEnum"=w1673) -> ()  [unwired: 2 in, 2 out]
      n1250 = property on="sweep rate, /min" class="DigNum (strict)"("DisabledEnum"=w1673) -> ()  [unwired: 2 in, 2 out]
    }
    frame #1 {
      n1251 = stacked-sequence {
        frame #0 {
          n1252 = local read "2636A smua meas v"() -> (w1679:bool)
          n1253 = local read "2636A smub meas v"() -> (w1677:bool)
          n1254 = local read "2636A smub meas i"() -> (w1676:bool)
          n1255 = local read "2636A smua meas i"() -> (w1678:bool)
          n1256 = Compound Arithmetic op=OR(w1679, w1678, w1677, w1676) -> (w1675:bool)
          n1257 = case shown="True" w1675 {
            frame False {
            }
            frame True {
              # "close session on 2636A"
              n1258 = local read "2336A addr"() -> (w1680:refnum<visa-resource-name>)
              n1259 = VISA Close(VISA resource name=w1680) -> ()  [unwired: 1 in, 1 out]
            }
          }
        }
        frame #1 {
          n1260 = local read "sweep"() -> (w1683:T3)
          n1261 = Equal?(x=w1683, y=T7."Radio Selection 7" ("sweep")) -> (x = y?=w1681:bool)
          n1262 = case shown="True" w1681 {
            frame False {
            }
            frame True {
              n1263 = local read "Hulk_SMS_addr"() -> (w1686:refnum<visa-resource-name>)
              n1264 = local read "CRYogenic:("() -> (w1685:errorcluster)
              n1265 = VISA Close(VISA resource name=w1686, error in (no error)=w1685) -> (error out=w1684:errorcluster)
              n1266 = local write "CRYogenic:("(w1684) -> ()
            }
          }
        }
      }
    }
    frame #2 {
      w1687 = FALSE  # clear devices  at the end
      n1267 = case shown="True" w1687 {
        frame False {
        }
        frame True {
          n1268 = DevClear() -> ()  [unwired: 3 in, 2 out]
        }
      }
    }
  }
